vi "Omniax_mDrive_XYZR_MM_BR_RES_2.vi"() -> ()   [LabVIEW 2009]
uses:
  <vilib>/Instr/_visa.llb/VISA Configure Serial Port (Instr).vi
panel:
  out "R Backlash steps/sec":i32
  out "R Backlash":i32
  out "R Holding Current %":i32
  out "R Run Current %":i32
  out "R offset deg":dbl
  out "R deg/rev":dbl
  out "R steps/rev":u32
  out "R velocity PV step/sec":i32
  out "R MINPOS":i32=-94296
  out "R MAXPOS":i32=-34296
  out "R COM PORT":refnum<visa-resource-name>="COM5"
  in  "R Scan set":bool
  in  "R Scan Velocity SP deg/sec":dbl
  in  "R Scan Length SP deg":dbl
  in  "R Move Set":bool
  out "Reset R Motor Steps":i32
  in  "Reset R Position deg":dbl
  out "R Velocity MVdeg/sec":dbl
  in  "R Velocity SP deg/sec":dbl
  in  "R Position SP deg":dbl
  out "R Position MV deg":dbl
  out "R Scan velocity MV deg/sec":dbl format="%#_6f"
  out "R Scan length MV deg":dbl
  in  "R Scan Length SP steps":i32 min=0 max=6144000 step=100
  in  "R Scan OK":bool
  in  "R Velocity SP step/sec":i32 min=1 max=102400
  in  "R Scan Velocity SP steps/sec":i32=1 min=1 max=102400 step=1
  in  "R Go":bool
  in  "R Step SP":i32=-20000 min=0 max=6144000 step=500
  out "R Position deg PV":dbl
  out "R Step PV":i32 max=2000
  out "R Backlash corr":bool
  out "R in Motion":bool
  out "R Scan":bool
  out "R in Range":bool
  out "Z COM PORT":refnum<visa-resource-name>="COM5"
  out "Z Backlash steps/sec":i32
  out "Z Backlash":i32
  out "Z Holding Current %":i32
  out "Z Run Current %":i32
  out "Z offset mm":dbl
  out "Z mm/rev":dbl
  out "Z steps/rev":u32
  out "Z  velocity PV step/sec":i32
  out "Z MINPOS":i32=-94296
  out "Z MAXPOS":i32=-34296
  in  "Z Scan set":bool
  in  "Z Scan Velocity SP mm/sec":dbl
  in  "Z Scan Length SP mm":dbl
  in  "Z Move Set":bool
  out "Reset Z Motor Steps":i32
  in  "Reset Z Position mm":dbl
  out "Z Velocity MV mm/sec":dbl
  in  "Z Velocity SP mm/sec":dbl
  in  "Z Position SP mm":dbl
  out "Z Position MV mm":dbl
  out "Z Scan velocity MV mm/sec":dbl format="%#_6f"
  out "Z Scan length MV mm":dbl
  in  "Z Scan Length SP steps":i32 min=0 max=2048000 step=100
  in  "Z Scan OK":bool
  in  "Z Velocity SP step/sec":i32 min=1 max=102400
  in  "Z Scan Velocity SP steps/sec":i32=1 min=1 max=102400 step=1
  in  "Z Go":bool
  in  "Z Step SP":i32=-20000 min=0 max=2048000 step=500
  out "Z Position mm PV":dbl
  out "Z Step PV":i32 max=2000
  out "Z Backlash corr":bool
  out "Z in Motion":bool
  out "Z Scan":bool
  out "Z in Range":bool
  out "Reset X Motor Steps":i32
  in  "Reset X Position mm":dbl
  out "X Backlash corr":bool
  out "X  in Motion":bool
  out "X Scan":bool
  out "X  in Range":bool
  out "X Step PV":i32 max=2000
  out "X Position mm PV":dbl
  out "X velocity PV step/sec":i32
  in  "X Scan set":bool
  in  "X Scan Velocity SP mm/sec":dbl
  in  "X Scan Length SP mm":dbl
  in  "X Move Set":bool
  out "X Velocity MV mm/sec":dbl
  in  "X Velocity SP mm/sec":dbl
  in  "X Position SP mm":dbl
  out "X Position MV mm":dbl
  out "X Scan velocity MV mm/sec":dbl format="%#_6f"
  out "X Scan length MV mm":dbl
  in  "X Scan Length SP steps":i32 min=-460800 max=460800 step=100
  in  "X Scan OK":bool
  in  "X Velocity SP step/sec":i32 min=1 max=102400
  in  "X Scan Velocity SP steps/sec":i32=1 min=1 max=102400 step=1
  in  "X Go":bool
  in  "X Step SP":i32=-20000 min=-460800 max=460800 step=500
  out "X Backlash steps/sec":i32
  out "X Backlash":i32
  out "X Holding Current %":i32
  out "X Run Current %":i32
  out "X offset mm":dbl
  out "X mm/rev":dbl
  out "X steps/rev":u32
  out "X MAXPOS":i32=-34296
  out "X MINPOS":i32=-94296
  out "X COM PORT":refnum<visa-resource-name>="COM5"
  out "Y Backlash corr":bool
  in  "Y Scan set":bool
  in  "Y Scan Velocity SP mm/sec":dbl
  in  "Y Scan Length SP mm":dbl
  in  "Y Move Set":bool
  out "Y Backlash steps/sec":i32
  out "Y Backlash":i32
  out "Y in Motion":bool
  in  "Reset":bool
  out "Reset Y Motor Steps":i32
  in  "Reset Y Position mm":dbl
  out "Y Velocity MV mm/sec":dbl
  in  "Y Velocity SP mm/sec":dbl
  in  "Y Position SP mm":dbl
  out "Y Position MV mm":dbl
  out "Y Holding Current %":i32
  out "Y Run Current %":i32
  out "Y Scan velocity MV mm/sec":dbl format="%#_6f"
  out "Y Scan length MV mm":dbl
  in  "Scan Cancel":bool
  out "Y Position mm PV":dbl
  out "Y offset mm":dbl
  out "Y mm/rev":dbl
  out "Y steps/rev":u32
  out "Y velocity PV step/sec":i32
  in  "Y Scan Length SP steps":i32 min=-460800 max=460800 step=100
  out "Y Scan":bool
  in  "Y Scan OK":bool
  in  "Scan Go":bool
  in  "Y Velocity SP step/sec":i32 min=1 max=102400
  in  "Y Scan Velocity SP steps/sec":i32=1 min=1 max=102400 step=1
  in  "Stop":bool
  out "Y in Range":bool
  out "Y Step PV":i32 max=2000
  in  "Y Go":bool
  in  "Y Step SP":i32=-20000 min=-460800 max=460800 step=500
  out "Y MINPOS":i32=-94296
  out "Y MAXPOS":i32=-34296
  out "Y COM PORT":refnum<visa-resource-name>="COM5"
  # "LM"
  # "MV"
  # "BL"
  # "SC"
  # "MX"
  # "MY"
  # "MZ"
  # "MR"
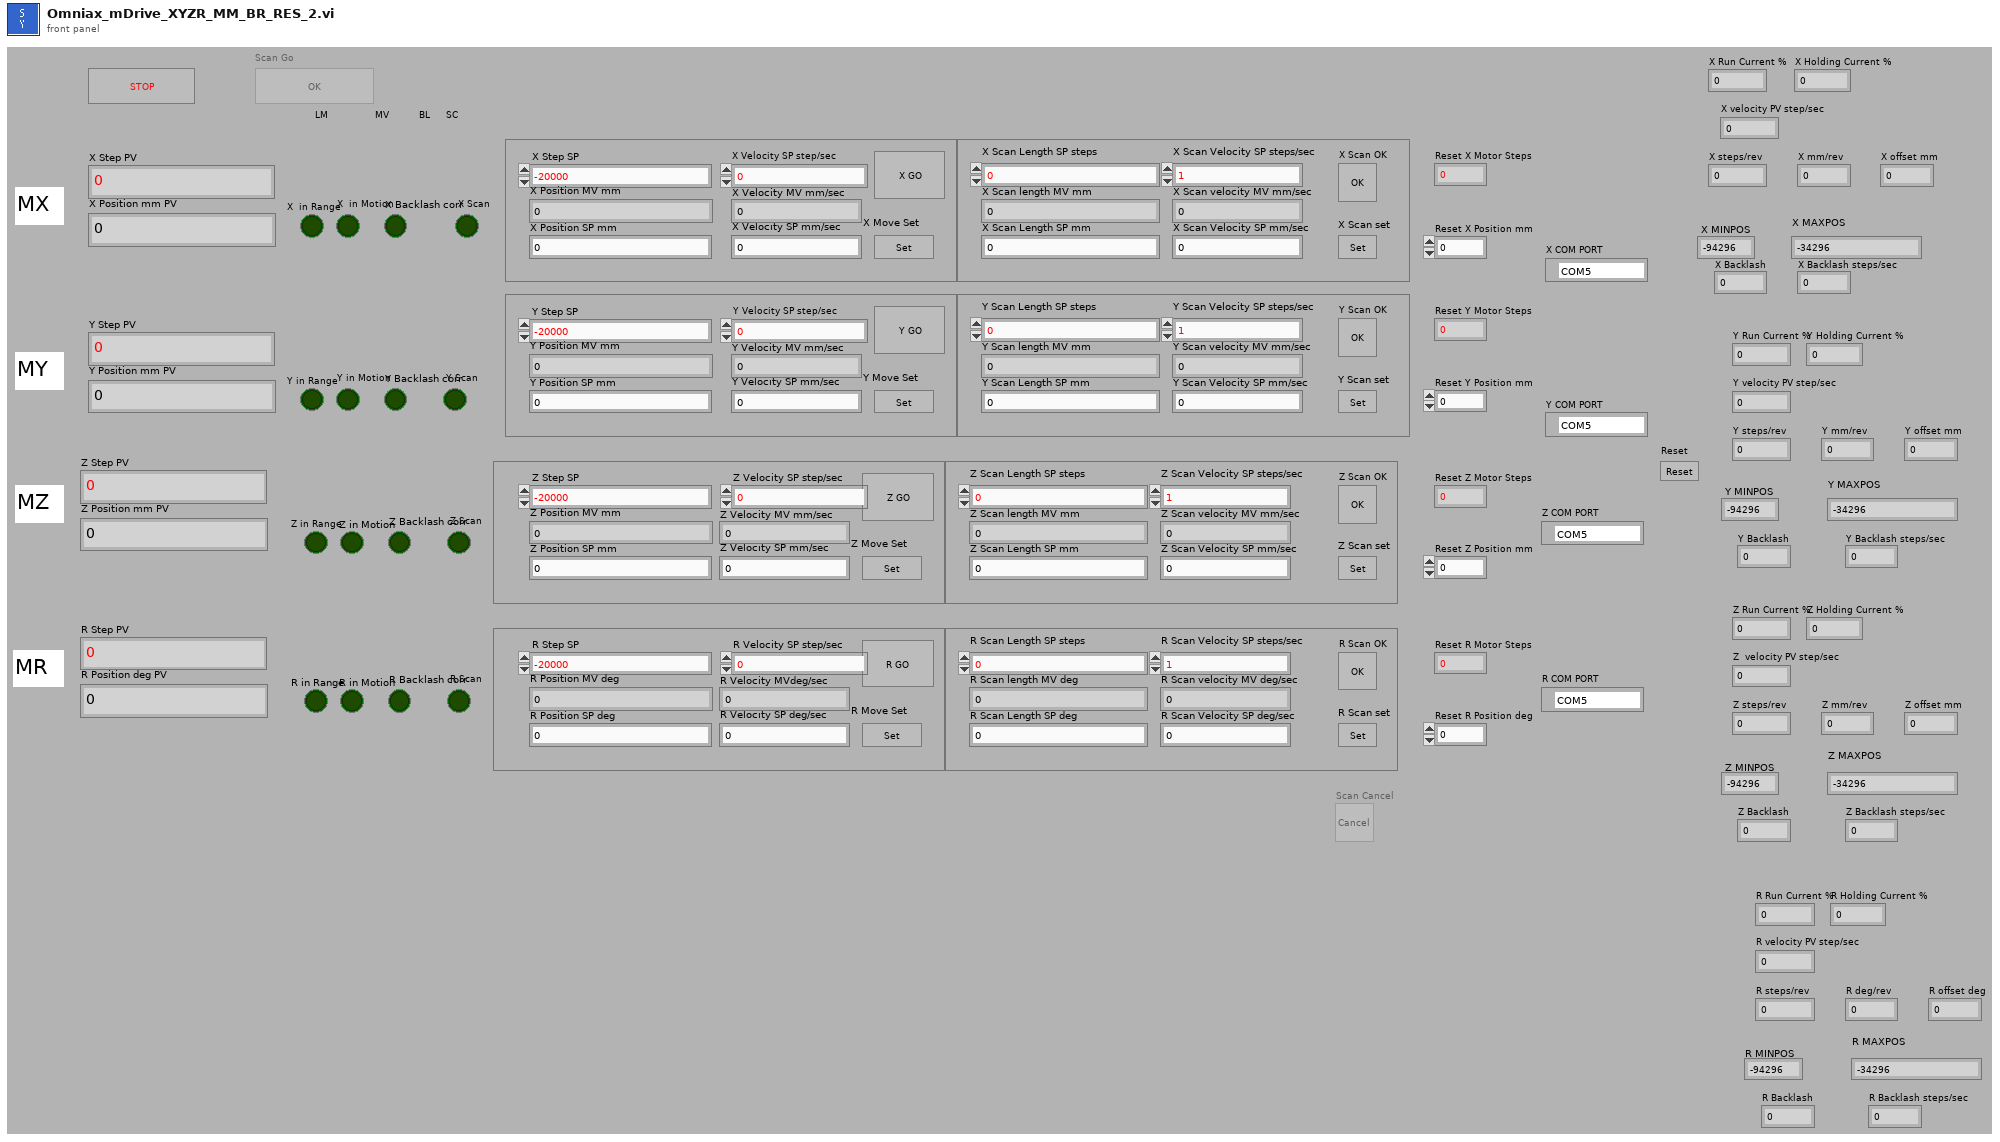
[diagram p1: front panel]
types:
  T1 = enum8{"Enabled", "Disabled", "Disabled and Grayed Out"}
  T2 = enum16{"Stop", "Reset", "Run Current", "Holding Current", "Accel Rate", "Decel Rate", "Move to Relative Position", "Move to Absolute Position", "Echo Mode", "Print Parameter", "Send String", "Microstep Resolution", "Set Current Position", "Max Velocity"}
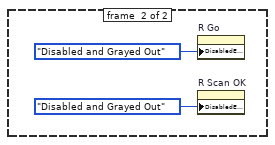
[diagram p2: hidden frame]
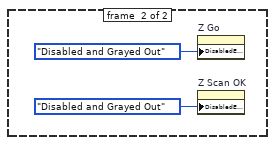
[diagram p5: hidden frame]
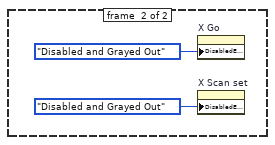
[diagram p8: hidden frame]
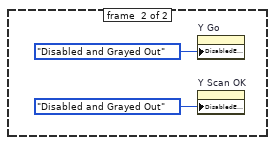
[diagram p11: hidden frame]
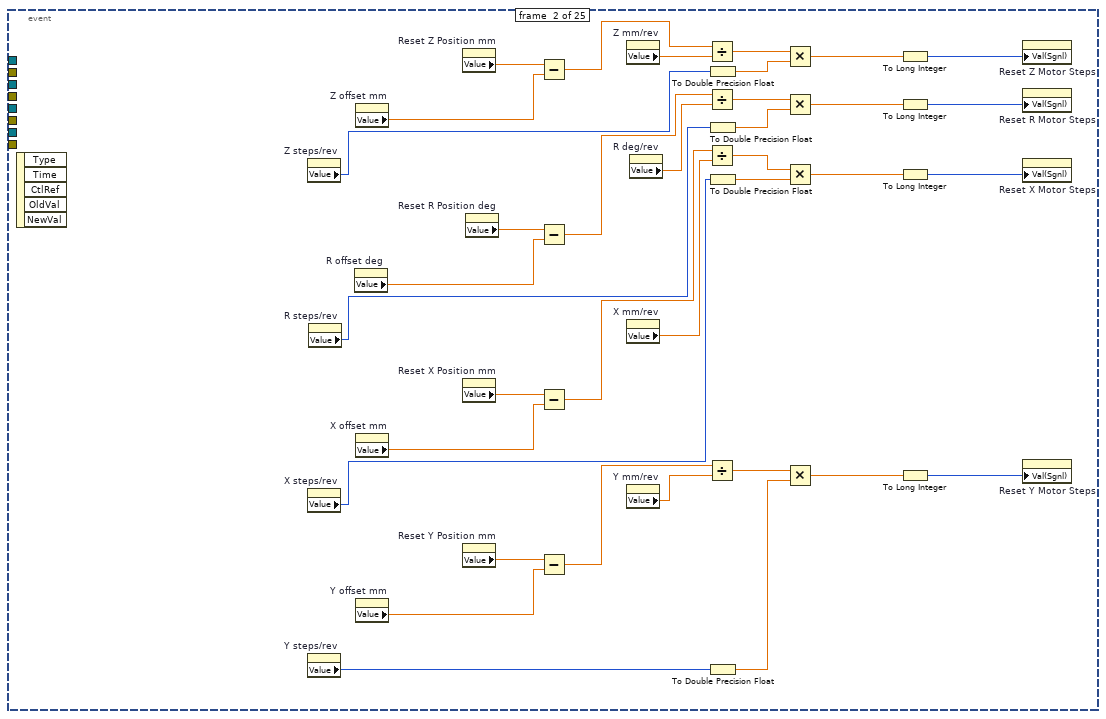
[diagram p14: hidden frame]
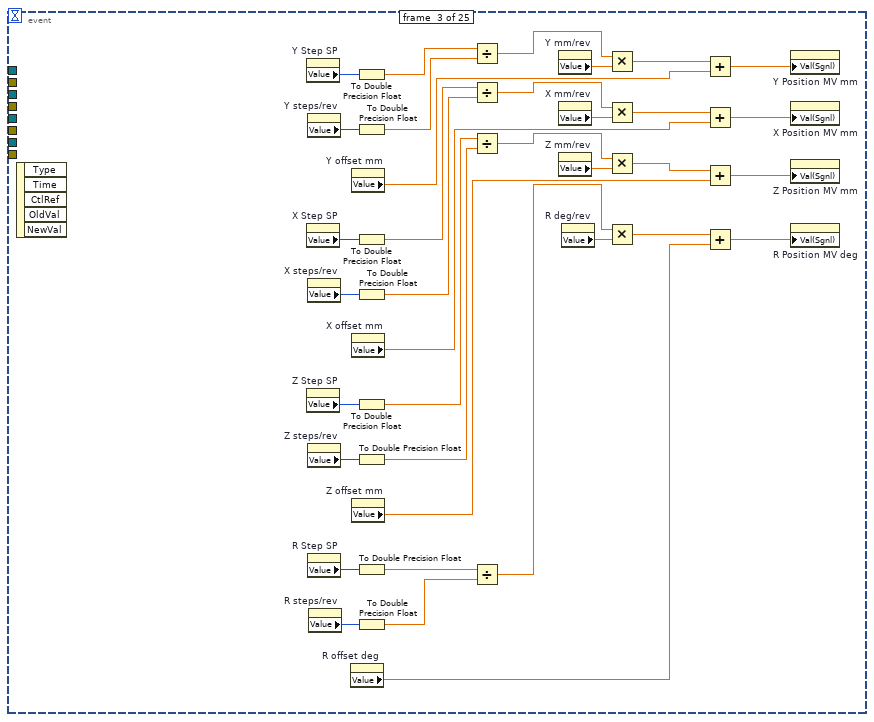
[diagram p15: hidden frame]
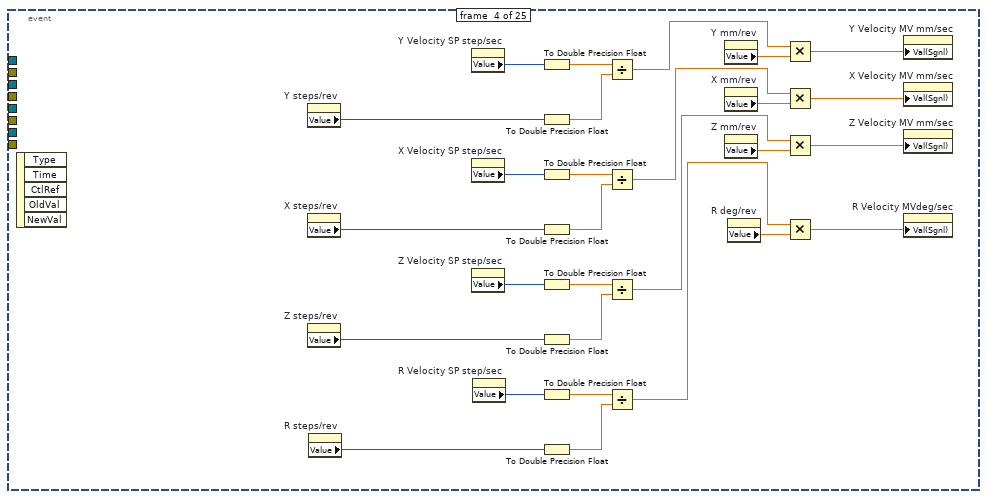
[diagram p16: hidden frame]
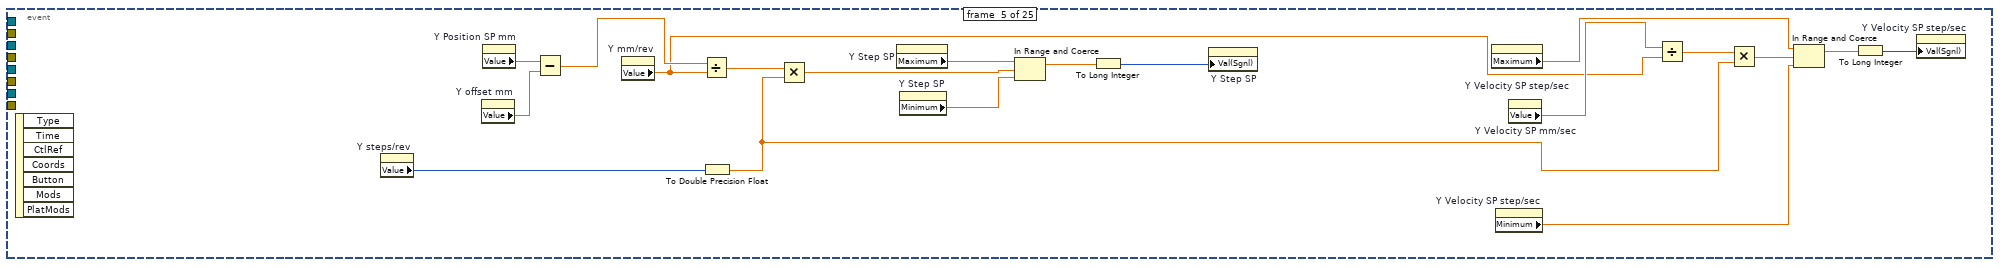
[diagram p17: hidden frame]
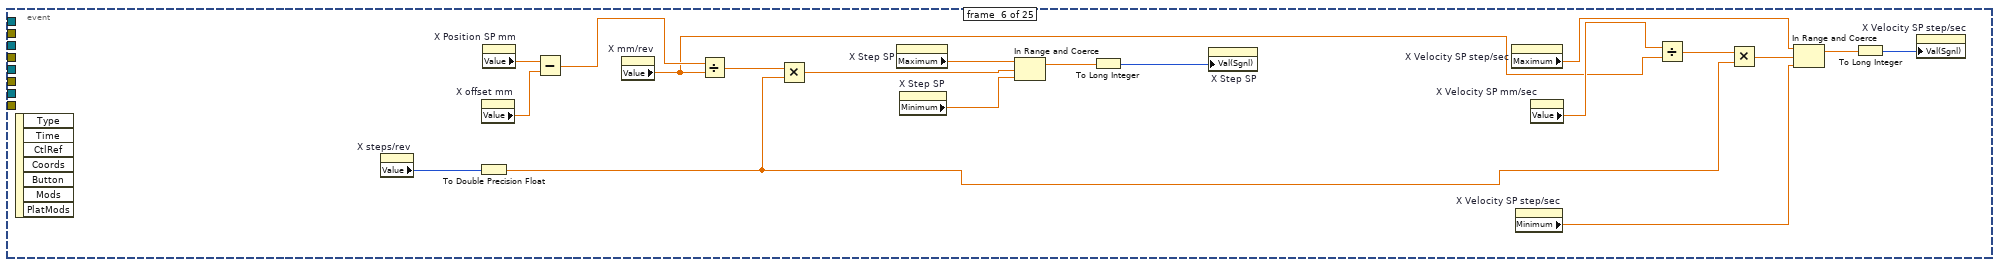
[diagram p18: hidden frame]
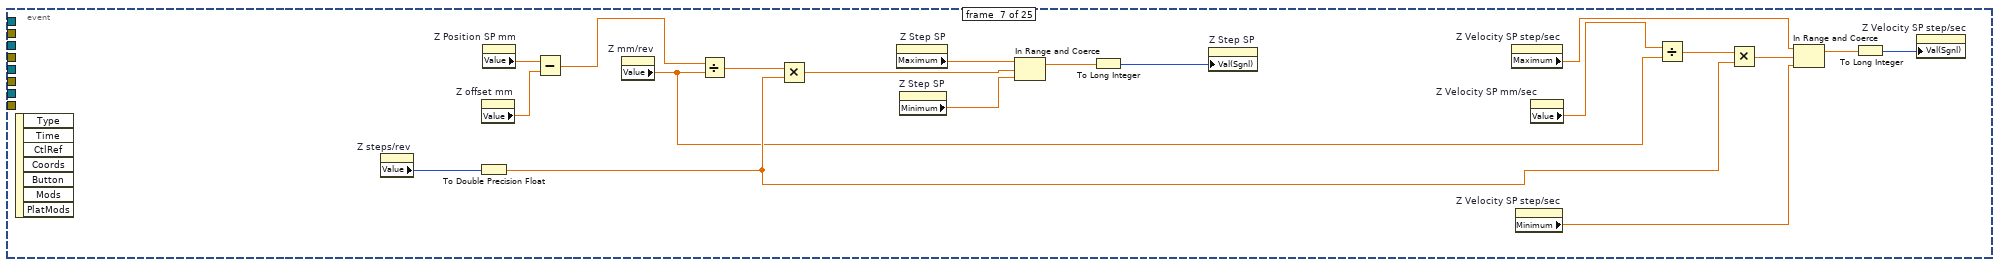
[diagram p19: hidden frame]
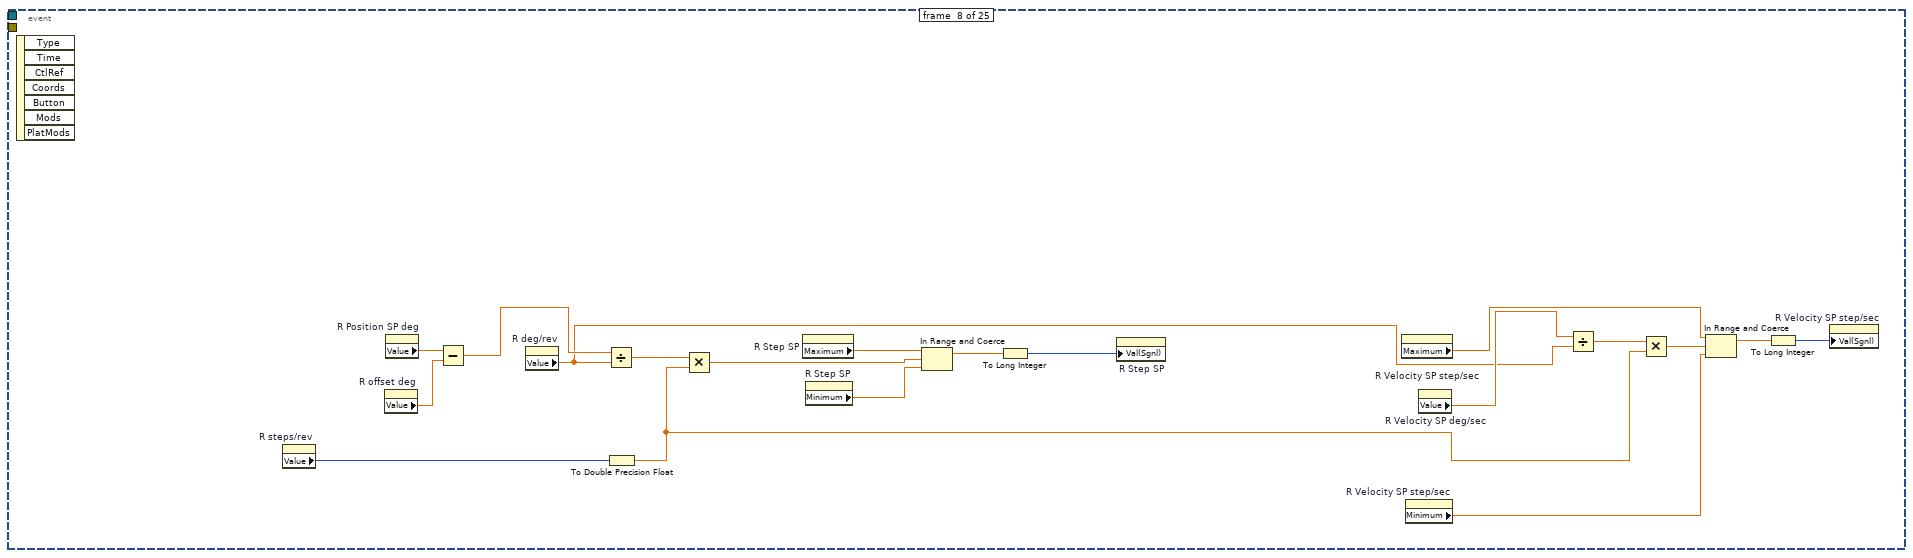
[diagram p20: hidden frame]
diagram:
  w19 = refnum<visa-resource-name> "COM11" ("COM PORT")
  w21 = u16 0 items=["None", "XON/XOFF", "RTS/CTS", "XON/XOFF & RTS/CTS", "DTR/DSR", "XON/XOFF & DTR/DSR"] ("flow control (0:none)")
  w22 = u16 10 items=["1.0"=10, "1.5"=15, "2.0"=20] ("stop bits (10: 1 bit)")
  w52 = refnum<visa-resource-name> "COM10" ("COM PORT")
  w54 = u16 0 items=["None", "XON/XOFF", "RTS/CTS", "XON/XOFF & RTS/CTS", "DTR/DSR", "XON/XOFF & DTR/DSR"] ("flow control (0:none)")
  w55 = u16 10 items=["1.0"=10, "1.5"=15, "2.0"=20] ("stop bits (10: 1 bit)")
  w65 = refnum<visa-resource-name> "COM8" ("COM PORT")
  w67 = u16 0 items=["None", "XON/XOFF", "RTS/CTS", "XON/XOFF & RTS/CTS", "DTR/DSR", "XON/XOFF & DTR/DSR"] ("flow control (0:none)")
  w68 = u16 10 items=["1.0"=10, "1.5"=15, "2.0"=20] ("stop bits (10: 1 bit)")
  w90 = refnum<visa-resource-name> "COM9" ("COM PORT")
  w92 = u16 0 items=["None", "XON/XOFF", "RTS/CTS", "XON/XOFF & RTS/CTS", "DTR/DSR", "XON/XOFF & DTR/DSR"] ("flow control (0:none)")
  w93 = u16 10 items=["1.0"=10, "1.5"=15, "2.0"=20] ("stop bits (10: 1 bit)")
  # "Stop bits"
  # "Stop bits"
  # "Stop bits"
  # "Stop bits"
  n1 = flat-sequence {
    frame #0 {
      w101 = 3.0 ("R deg/rev")
      w99 = u32 51200 ("step/rev")
      w103 = 102400 ("Value (Signaling)")
      n2 = property on="R Velocity SP step/sec" class="DigNum (strict)"("Val(Sgnl)"=w103) -> ()  [unwired: 2 in, 2 out]
      n3 = property on="R Velocity SP step/sec" class="DigNum (strict)"("Minimum"=1.0 ("Data Entry Limits:Minimum")) -> ()  [unwired: 2 in, 2 out]
      n4 = To Double Precision Float(number=w99) -> (double precision float=w100:dbl)
      n5 = To Double Precision Float(number=w103) -> (double precision float=w105:dbl)
      n6 = Divide(x=w105, y=w100) -> (x/y=w104:dbl)
      n7 = property on="R Velocity SP step/sec" class="DigNum (strict)"("Maximum"=w105) -> ()  [unwired: 2 in, 2 out]
      n8 = Multiply(x=w104, y=w101) -> (x*y=w102:dbl)
      n9 = property on="R Velocity SP deg/sec" class="DigNum (strict)"("Val(Sgnl)"=w102) -> ()  [unwired: 2 in, 2 out]
      "R offset deg" <- 0.0 ("R offset deg")
      "R deg/rev" <- w101
      "R steps/rev" <- w99
    }
  }
  n10 = flat-sequence {
    frame #0 {
      w108 = 1.0 ("MM/rev")
      w111 = u32 51200 ("step/rev")
      w106 = 102400 ("Value (Signaling)")
      n11 = property on="X Velocity SP step/sec" class="DigNum (strict)"("Minimum"=1.0 ("Data Entry Limits:Minimum")) -> ()  [unwired: 2 in, 2 out]
      n12 = property on="X Velocity SP step/sec" class="DigNum (strict)"("Val(Sgnl)"=w106) -> ()  [unwired: 2 in, 2 out]
      n13 = To Double Precision Float(number=w111) -> (double precision float=w110:dbl)
      n14 = To Double Precision Float(number=w106) -> (double precision float=w112:dbl)
      n15 = Divide(x=w112, y=w110) -> (x/y=w107:dbl)
      n16 = property on="X Velocity SP step/sec" class="DigNum (strict)"("Maximum"=w112) -> ()  [unwired: 2 in, 2 out]
      n17 = Multiply(x=w107, y=w108) -> (x*y=w109:dbl)
      n18 = property on="X Velocity SP mm/sec" class="DigNum (strict)"("Val(Sgnl)"=w109) -> ()  [unwired: 2 in, 2 out]
      "X offset mm" <- 0.0 ("offset")
      "X steps/rev" <- w111
      "X mm/rev" <- w108
    }
  }
  n19 = flat-sequence {
    frame #0 {
      w116 = 1.0 ("Z mm/rev")
      w115 = u32 51200 ("step/rev")
      w117 = 102400 ("Value (Signaling)")
      n20 = property on="Z Velocity SP step/sec" class="DigNum (strict)"("Val(Sgnl)"=w117) -> ()  [unwired: 2 in, 2 out]
      n21 = property on="Z Velocity SP step/sec" class="DigNum (strict)"("Minimum"=1.0 ("Data Entry Limits:Minimum")) -> ()  [unwired: 2 in, 2 out]
      n22 = To Double Precision Float(number=w115) -> (double precision float=w120:dbl)
      n23 = To Double Precision Float(number=w117) -> (double precision float=w121:dbl)
      n24 = Divide(x=w121, y=w120) -> (x/y=w118:dbl)
      n25 = property on="Z Velocity SP step/sec" class="DigNum (strict)"("Maximum"=w121) -> ()  [unwired: 2 in, 2 out]
      n26 = Multiply(x=w118, y=w116) -> (x*y=w119:dbl)
      n27 = property on="Z Velocity SP mm/sec" class="DigNum (strict)"("Val(Sgnl)"=w119) -> ()  [unwired: 2 in, 2 out]
      "Z offset mm" <- 0.0 ("Z offset mm")
      "Z mm/rev" <- w116
      "Z steps/rev" <- w115
    }
  }
  n28 = flat-sequence {
    frame #0 {
      n29 = property on="X Backlash corr" class="Bool (strict)"("Val(Sgnl)"=FALSE ("Value (Signaling)")) -> ()  [unwired: 2 in, 2 out]
      n30 = property on="R Backlash corr" class="Bool (strict)"("Val(Sgnl)"=FALSE ("Value (Signaling)")) -> ()  [unwired: 2 in, 2 out]
      n31 = property on="Z Backlash corr" class="Bool (strict)"("Val(Sgnl)"=FALSE ("Value (Signaling)")) -> ()  [unwired: 2 in, 2 out]
      n32 = property on="Y Backlash corr" class="Bool (strict)"("Val(Sgnl)"=FALSE ("Value (Signaling)")) -> ()  [unwired: 2 in, 2 out]
      "Z Backlash steps/sec" <- 25600 ("Z Backlash steps/sec")
      "Z Backlash" <- -12800 ("Z Backlash")
      "X Backlash steps/sec" <- 25600 ("Value (Signaling)")
      "X Backlash" <- -5120 ("Backlash2")
      "Y Backlash" <- -5120 ("Backlash2")
      "Y Backlash steps/sec" <- 25600 ("Value (Signaling)")
      "R Backlash steps/sec" <- 25600 ("R Backlash steps/sec")
      "R Backlash" <- -12800 ("R Backlash")
    }
  }
  n33 = flat-sequence {
    frame #0 {
      "Z Holding Current %" <- 25 ("Z Holding Current %")
      "Z Run Current %" <- 60 ("Z Run Current %")
      "X Run Current %" <- 60 ("Run Current %")
      "X Holding Current %" <- 25 ("Holding Current %")
      "Y Run Current %" <- 60 ("Run Current %")
      "Y Holding Current %" <- 25 ("Holding Current %")
      "R Holding Current %" <- 25 ("R Holding Current %")
      "R Run Current %" <- 60 ("R Run Current %")
    }
  }
  n34 = flat-sequence {
    frame #0 {
      n35 = property on="Y Scan" class="Bool (strict)"("Val(Sgnl)"=FALSE ("Value (Signaling)")) -> ()  [unwired: 2 in, 2 out]
      n36 = property on="Y Scan Velocity SP mm/sec" class="DigNum (strict)"("Val(Sgnl)"=0.1 ("Value (Signaling)")) -> ()  [unwired: 2 in, 2 out]
      n37 = property on="Z Scan Velocity SP mm/sec" class="DigNum (strict)"("Val(Sgnl)"=0.1 ("Value (Signaling)")) -> ()  [unwired: 2 in, 2 out]
      n38 = property on="R Scan" class="Bool (strict)"("Val(Sgnl)"=FALSE ("Value (Signaling)")) -> ()  [unwired: 2 in, 2 out]
      n39 = property on="Z Scan" class="Bool (strict)"("Val(Sgnl)"=FALSE ("Value (Signaling)")) -> ()  [unwired: 2 in, 2 out]
      n40 = property on="R Velocity SP deg/sec" class="DigNum (strict)"("Val(Sgnl)"=0.1 ("Value (Signaling)")) -> ()  [unwired: 2 in, 2 out]
      n41 = property on="X Scan" class="Bool (strict)"("Val(Sgnl)"=FALSE ("Value (Signaling)")) -> ()  [unwired: 2 in, 2 out]
      n42 = property on="X Scan Velocity SP mm/sec" class="DigNum (strict)"("Val(Sgnl)"=0.1 ("Value (Signaling)")) -> ()  [unwired: 2 in, 2 out]
      n43 = property on="Scan Go" class="Bool"("DisabledEnum"=T1."Disabled and Grayed Out" ("Disabled")) -> ()  [unwired: 2 in, 2 out]
      n44 = property on="Scan Cancel" class="Bool"("DisabledEnum"=T1."Disabled and Grayed Out" ("Disabled")) -> ()  [unwired: 2 in, 2 out]
    }
  }
  n45 = flat-sequence {
    frame #0 {
      w156 = 1.0 ("MM/rev")
      w159 = u32 51200 ("step/rev")
      w154 = 102400 ("Value (Signaling)")
      n46 = property on="Y Velocity SP step/sec" class="DigNum (strict)"("Minimum"=1.0 ("Data Entry Limits:Minimum")) -> ()  [unwired: 2 in, 2 out]
      n47 = property on="Y Velocity SP step/sec" class="DigNum (strict)"("Val(Sgnl)"=w154) -> ()  [unwired: 2 in, 2 out]
      n48 = To Double Precision Float(number=w159) -> (double precision float=w158:dbl)
      n49 = To Double Precision Float(number=w154) -> (double precision float=w160:dbl)
      n50 = Divide(x=w160, y=w158) -> (x/y=w155:dbl)
      n51 = property on="Y Velocity SP step/sec" class="DigNum (strict)"("Maximum"=w160) -> ()  [unwired: 2 in, 2 out]
      n52 = Multiply(x=w155, y=w156) -> (x*y=w157:dbl)
      n53 = property on="Y Velocity SP mm/sec" class="DigNum (strict)"("Val(Sgnl)"=w157) -> ()  [unwired: 2 in, 2 out]
      "Y offset mm" <- 0.0 ("offset")
      "Y steps/rev" <- w159
      "Y mm/rev" <- w156
    }
  }
  n54 = call-poly "VISA Configure Serial Port"("VISA resource name"=w90, "timeout (10sec)"=u32 10000, "baud rate (9600)"=u32 9600, "data bits (8)"=u16 8, "parity (0:none)"=enum16{"None", "Odd", "Even", "Mark", "Space"}."None", "stop bits (10: 1 bit)"=w93, "flow control (0:none)"=w92) -> ("VISA resource name out"=w83:refnum<visa-resource-name>, "error out"=w82:errorcluster)  [unwired: 7 in]
  n55 = flat-sequence {
    tunnel: w82 -> [w165]
    tunnel: w83 -> [w166]
    tunnel: [w166] -> w4
    tunnel: [w165] -> w3
    tunnel: [w170] -> w81
    tunnel: [w172] -> w79
    tunnel: w4 -> [w171]
    tunnel: w3 -> [w173]
    tunnel: w81 -> [w180]
    tunnel: [w179] -> w80
    tunnel: w79 -> [w177]
    tunnel: [w178] -> w78
    tunnel: [w190] -> w85
    tunnel: [w191] -> w84
    tunnel: w80 -> [w189]
    tunnel: w78 -> [w188]
    tunnel: w85 -> [w201]
    tunnel: w84 -> [w200]
    tunnel: [w203] -> w51
    tunnel: [w202] -> w50
    tunnel: [w197] -> w49
    tunnel: [w208] -> w88
    tunnel: [w209] -> w89
    tunnel: w51 -> [w209]
    tunnel: w50 -> [w208]
    tunnel: w49 -> [w204]
    frame #0 {
      n56 = call "mDrive Send Command.vi"("Extra"="EM=2", "Command"=T2."Send String") -> ()  [unwired: 5 in, 3 out]
    }
    frame #1 {
      # "Run Current %"
      n57 = property on="Y Run Current %" class="DigNum (strict)"() -> ("Value"=w168:i32)  [unwired: 2 in, 2 out]
      n58 = Number To Decimal String(number=w168) -> (decimal integer string=w169:string)  [unwired: 1 in]
      n59 = call "mDrive Send Command.vi"("error in (no error)"=w173, "Extra"=w169, "Command"=T2."Run Current", "VISA resource name"=w171) -> ("error out"=w172:errorcluster, "VISA resource name out"=w170:refnum<visa-resource-name>)  [unwired: 3 in, 1 out]
    }
    frame #2 {
      # "Holding Current %"
      n60 = property on="Y Holding Current %" class="DigNum (strict)"() -> ("Value"=w175:i32)  [unwired: 2 in, 2 out]
      n61 = Number To Decimal String(number=w175) -> (decimal integer string=w176:string)  [unwired: 1 in]
      n62 = call "mDrive Send Command.vi"("error in (no error)"=w177, "Extra"=w176, "Command"=T2."Holding Current", "VISA resource name"=w180) -> ("error out"=w178:errorcluster, "VISA resource name out"=w179:refnum<visa-resource-name>)  [unwired: 3 in, 1 out]
    }
    frame #3 {
      # "Print Velocity Ma"
      # "Velocity Max"
      n63 = property on="Y Velocity SP step/sec" class="DigNum (strict)"() -> ("Value"=w187:i32)  [unwired: 2 in, 2 out]
      n64 = Number To Decimal String(number=w187) -> (decimal integer string=w186:string)  [unwired: 1 in]
      n65 = call "mDrive Send Command.vi"("error in (no error)"=w188, "Extra"=w186, "Command"=T2."Max Velocity", "VISA resource name"=w189) -> ("error out"=w184:errorcluster, "VISA resource name out"=w194:refnum<visa-resource-name>)  [unwired: 3 in, 1 out]
      n66 = call "mDrive Send Command.vi"("error in (no error)"=w184, "Extra"="VM", "Command"=T2."Print Parameter", "VISA resource name"=w194) -> ("error out"=w191:errorcluster, "read buffer"=w192:string, "VISA resource name out"=w190:refnum<visa-resource-name>)  [unwired: 3 in]
      n67 = Decimal String To Number(string=w192, offset=0) -> (number=w185:i32)  [unwired: 1 in, 1 out]
      n68 = property on="Y scan velocity MV step/sec" class="DigNum (strict)"("Val(Sgnl)"=w185) -> ()  [unwired: 2 in, 2 out]
    }
    frame #4 {
      # "PRINT POSITION"
      n69 = call "mDrive Send Command.vi"("error in (no error)"=w200, "Extra"="P", "Command"=T2."Print Parameter", "VISA resource name"=w201) -> ("error out"=w202:errorcluster, "read buffer"=w199:string, "VISA resource name out"=w203:refnum<visa-resource-name>)  [unwired: 3 in]
      n70 = Decimal String To Number(string=w199, offset=0) -> (number=w197:i32)  [unwired: 1 in, 1 out]
    }
    frame #5 {
      w206 = -460800 ("lower limit")
      w207 = 460800 ("upper limit")
      n71 = property on="Y Step SP" class="DigNum (strict)"("Val(Sgnl)"=w204) -> ()  [unwired: 2 in, 2 out]
      n72 = property on="Y Step SP" class="DigNum (strict)"("Maximum"=w207) -> ()  [unwired: 2 in, 2 out]
      n73 = property on="Y Step SP" class="DigNum (strict)"("Minimum"=w206) -> ()  [unwired: 2 in, 2 out]
      n74 = In Range and Coerce(upper limit=w207, x=w204, lower limit=w206) -> (In Range?=w205:bool)  [unwired: 1 out]
      n75 = property on="Y in Range" class="Bool (strict)"("Val(Sgnl)"=w205) -> ()  [unwired: 2 in, 2 out]
      "Y MINPOS" <- w206
      "Y MAXPOS" <- w207
    }
  }
  n76 = call-poly "VISA Configure Serial Port"("VISA resource name"=w65, "timeout (10sec)"=u32 10000, "baud rate (9600)"=u32 9600, "data bits (8)"=u16 8, "parity (0:none)"=enum16{"None", "Odd", "Even", "Mark", "Space"}."None", "stop bits (10: 1 bit)"=w68, "flow control (0:none)"=w67) -> ("VISA resource name out"=w64:refnum<visa-resource-name>, "error out"=w63:errorcluster)  [unwired: 7 in]
  n77 = call-poly "VISA Configure Serial Port"("VISA resource name"=w19, "timeout (10sec)"=u32 10000, "baud rate (9600)"=u32 9600, "data bits (8)"=u16 8, "parity (0:none)"=enum16{"None", "Odd", "Even", "Mark", "Space"}."None", "stop bits (10: 1 bit)"=w22, "flow control (0:none)"=w21) -> ("VISA resource name out"=w18:refnum<visa-resource-name>, "error out"=w17:errorcluster)  [unwired: 7 in]
  n78 = flat-sequence {
    tunnel: w17 -> [w212]
    tunnel: w18 -> [w213]
    tunnel: [w213] -> w8
    tunnel: [w212] -> w7
    tunnel: [w218] -> w34
    tunnel: [w220] -> w33
    tunnel: w8 -> [w219]
    tunnel: w7 -> [w214]
    tunnel: w34 -> [w227]
    tunnel: [w226] -> w32
    tunnel: w33 -> [w224]
    tunnel: [w225] -> w31
    tunnel: [w237] -> w30
    tunnel: [w238] -> w29
    tunnel: w32 -> [w236]
    tunnel: w31 -> [w235]
    tunnel: w30 -> [w248]
    tunnel: w29 -> [w247]
    tunnel: [w250] -> w28
    tunnel: [w249] -> w27
    tunnel: [w244] -> w26
    tunnel: [w255] -> w11
    tunnel: [w256] -> w12
    tunnel: w28 -> [w256]
    tunnel: w27 -> [w255]
    tunnel: w26 -> [w253]
    frame #0 {
      n79 = call "mDrive Send Command.vi"("Extra"="EM=2", "Command"=T2."Send String") -> ()  [unwired: 5 in, 3 out]
    }
    frame #1 {
      # "Run Current %"
      n80 = property on="R Run Current %" class="DigNum (strict)"() -> ("Value"=w216:i32)  [unwired: 2 in, 2 out]
      n81 = Number To Decimal String(number=w216) -> (decimal integer string=w217:string)  [unwired: 1 in]
      n82 = call "mDrive Send Command.vi"("error in (no error)"=w214, "Extra"=w217, "Command"=T2."Run Current", "VISA resource name"=w219) -> ("error out"=w220:errorcluster, "VISA resource name out"=w218:refnum<visa-resource-name>)  [unwired: 3 in, 1 out]
    }
    frame #2 {
      # "Holding Current %"
      n83 = property on="R Holding Current %" class="DigNum (strict)"() -> ("Value"=w222:i32)  [unwired: 2 in, 2 out]
      n84 = Number To Decimal String(number=w222) -> (decimal integer string=w223:string)  [unwired: 1 in]
      n85 = call "mDrive Send Command.vi"("error in (no error)"=w224, "Extra"=w223, "Command"=T2."Holding Current", "VISA resource name"=w227) -> ("error out"=w225:errorcluster, "VISA resource name out"=w226:refnum<visa-resource-name>)  [unwired: 3 in, 1 out]
    }
    frame #3 {
      # "Print Velocity Ma"
      # "Velocity Max"
      n86 = property on="R Velocity SP step/sec" class="DigNum (strict)"() -> ("Value"=w234:i32)  [unwired: 2 in, 2 out]
      n87 = Number To Decimal String(number=w234) -> (decimal integer string=w233:string)  [unwired: 1 in]
      n88 = call "mDrive Send Command.vi"("error in (no error)"=w235, "Extra"=w233, "Command"=T2."Max Velocity", "VISA resource name"=w236) -> ("error out"=w231:errorcluster, "VISA resource name out"=w241:refnum<visa-resource-name>)  [unwired: 3 in, 1 out]
      n89 = call "mDrive Send Command.vi"("error in (no error)"=w231, "Extra"="VM", "Command"=T2."Print Parameter", "VISA resource name"=w241) -> ("error out"=w238:errorcluster, "read buffer"=w239:string, "VISA resource name out"=w237:refnum<visa-resource-name>)  [unwired: 3 in]
      n90 = Decimal String To Number(string=w239, offset=0) -> (number=w232:i32)  [unwired: 1 in, 1 out]
      n91 = property on="R velocity PV step/sec" class="DigNum (strict)"("Val(Sgnl)"=w232) -> ()  [unwired: 2 in, 2 out]
    }
    frame #4 {
      # "PRINT POSITION"
      n92 = call "mDrive Send Command.vi"("error in (no error)"=w247, "Extra"="P", "Command"=T2."Print Parameter", "VISA resource name"=w248) -> ("error out"=w249:errorcluster, "read buffer"=w246:string, "VISA resource name out"=w250:refnum<visa-resource-name>)  [unwired: 3 in]
      n93 = Decimal String To Number(string=w246, offset=0) -> (number=w244:i32)  [unwired: 1 in, 1 out]
    }
    frame #5 {
      w252 = 0 ("lower limit")
      w251 = 6144000 ("upper limit")
      n94 = property on="R Step SP" class="DigNum (strict)"("Val(Sgnl)"=w253) -> ()  [unwired: 2 in, 2 out]
      n95 = property on="R Step SP" class="DigNum (strict)"("Maximum"=w251) -> ()  [unwired: 2 in, 2 out]
      n96 = property on="R Step SP" class="DigNum (strict)"("Minimum"=w252) -> ()  [unwired: 2 in, 2 out]
      n97 = In Range and Coerce(upper limit=w251, x=w253, lower limit=w252) -> (In Range?=w254:bool)  [unwired: 1 out]
      n98 = property on="R in Range" class="Bool (strict)"("Val(Sgnl)"=w254) -> ()  [unwired: 2 in, 2 out]
      "R MINPOS" <- w252
      "R MAXPOS" <- w251
    }
  }
  n99 = flat-sequence {
    tunnel: w63 -> [w259]
    tunnel: w64 -> [w260]
    tunnel: [w260] -> w2
    tunnel: [w259] -> w1
    tunnel: [w264] -> w77
    tunnel: [w266] -> w76
    tunnel: w2 -> [w265]
    tunnel: w1 -> [w267]
    tunnel: w77 -> [w274]
    tunnel: [w273] -> w75
    tunnel: w76 -> [w271]
    tunnel: [w272] -> w74
    tunnel: [w284] -> w73
    tunnel: [w285] -> w72
    tunnel: w75 -> [w283]
    tunnel: w74 -> [w282]
    tunnel: w73 -> [w295]
    tunnel: w72 -> [w294]
    tunnel: [w297] -> w48
    tunnel: [w296] -> w47
    tunnel: [w291] -> w46
    tunnel: [w302] -> w61
    tunnel: [w303] -> w62
    tunnel: w48 -> [w303]
    tunnel: w47 -> [w302]
    tunnel: w46 -> [w298]
    frame #0 {
      n100 = call "mDrive Send Command.vi"("Extra"="EM=2", "Command"=T2."Send String") -> ()  [unwired: 5 in, 3 out]
    }
    frame #1 {
      # "Run Current %"
      n101 = property on="X Run Current %" class="DigNum (strict)"() -> ("Value"=w262:i32)  [unwired: 2 in, 2 out]
      n102 = Number To Decimal String(number=w262) -> (decimal integer string=w263:string)  [unwired: 1 in]
      n103 = call "mDrive Send Command.vi"("error in (no error)"=w267, "Extra"=w263, "Command"=T2."Run Current", "VISA resource name"=w265) -> ("error out"=w266:errorcluster, "VISA resource name out"=w264:refnum<visa-resource-name>)  [unwired: 3 in, 1 out]
    }
    frame #2 {
      # "Holding Current %"
      n104 = property on="X Holding Current %" class="DigNum (strict)"() -> ("Value"=w269:i32)  [unwired: 2 in, 2 out]
      n105 = Number To Decimal String(number=w269) -> (decimal integer string=w270:string)  [unwired: 1 in]
      n106 = call "mDrive Send Command.vi"("error in (no error)"=w271, "Extra"=w270, "Command"=T2."Holding Current", "VISA resource name"=w274) -> ("error out"=w272:errorcluster, "VISA resource name out"=w273:refnum<visa-resource-name>)  [unwired: 3 in, 1 out]
    }
    frame #3 {
      # "Print Velocity Ma"
      # "Velocity Max"
      n107 = property on="X Velocity SP step/sec" class="DigNum (strict)"() -> ("Value"=w281:i32)  [unwired: 2 in, 2 out]
      n108 = Number To Decimal String(number=w281) -> (decimal integer string=w280:string)  [unwired: 1 in]
      n109 = call "mDrive Send Command.vi"("error in (no error)"=w282, "Extra"=w280, "Command"=T2."Max Velocity", "VISA resource name"=w283) -> ("error out"=w278:errorcluster, "VISA resource name out"=w288:refnum<visa-resource-name>)  [unwired: 3 in, 1 out]
      n110 = call "mDrive Send Command.vi"("error in (no error)"=w278, "Extra"="VM", "Command"=T2."Print Parameter", "VISA resource name"=w288) -> ("error out"=w285:errorcluster, "read buffer"=w286:string, "VISA resource name out"=w284:refnum<visa-resource-name>)  [unwired: 3 in]
      n111 = Decimal String To Number(string=w286, offset=0) -> (number=w279:i32)  [unwired: 1 in, 1 out]
      n112 = property on="X velocity PV step/sec" class="DigNum (strict)"("Val(Sgnl)"=w279) -> ()  [unwired: 2 in, 2 out]
    }
    frame #4 {
      # "PRINT POSITION"
      n113 = call "mDrive Send Command.vi"("error in (no error)"=w294, "Extra"="P", "Command"=T2."Print Parameter", "VISA resource name"=w295) -> ("error out"=w296:errorcluster, "read buffer"=w293:string, "VISA resource name out"=w297:refnum<visa-resource-name>)  [unwired: 3 in]
      n114 = Decimal String To Number(string=w293, offset=0) -> (number=w291:i32)  [unwired: 1 in, 1 out]
    }
    frame #5 {
      w300 = -460800 ("lower limit")
      w301 = 460800 ("upper limit")
      n115 = property on="X Step SP" class="DigNum (strict)"("Val(Sgnl)"=w298) -> ()  [unwired: 2 in, 2 out]
      n116 = property on="X Step SP" class="DigNum (strict)"("Maximum"=w301) -> ()  [unwired: 2 in, 2 out]
      n117 = property on="X Step SP" class="DigNum (strict)"("Minimum"=w300) -> ()  [unwired: 2 in, 2 out]
      n118 = In Range and Coerce(upper limit=w301, x=w298, lower limit=w300) -> (In Range?=w299:bool)  [unwired: 1 out]
      n119 = property on="X  in Range" class="Bool (strict)"("Val(Sgnl)"=w299) -> ()  [unwired: 2 in, 2 out]
      "X MINPOS" <- w300
      "X MAXPOS" <- w301
    }
  }
  n120 = call-poly "VISA Configure Serial Port"("VISA resource name"=w52, "timeout (10sec)"=u32 10000, "baud rate (9600)"=u32 9600, "data bits (8)"=u16 8, "parity (0:none)"=enum16{"None", "Odd", "Even", "Mark", "Space"}."None", "stop bits (10: 1 bit)"=w55, "flow control (0:none)"=w54) -> ("VISA resource name out"=w36:refnum<visa-resource-name>, "error out"=w35:errorcluster)  [unwired: 7 in]
  n121 = flat-sequence {
    tunnel: w35 -> [w306]
    tunnel: w36 -> [w307]
    tunnel: [w307] -> w6
    tunnel: [w306] -> w5
    tunnel: [w311] -> w45
    tunnel: [w313] -> w44
    tunnel: w6 -> [w312]
    tunnel: w5 -> [w314]
    tunnel: w45 -> [w321]
    tunnel: [w320] -> w43
    tunnel: w44 -> [w318]
    tunnel: [w319] -> w42
    tunnel: [w331] -> w41
    tunnel: [w332] -> w40
    tunnel: w43 -> [w330]
    tunnel: w42 -> [w329]
    tunnel: w41 -> [w342]
    tunnel: w40 -> [w341]
    tunnel: [w344] -> w39
    tunnel: [w343] -> w38
    tunnel: [w338] -> w37
    tunnel: [w349] -> w15
    tunnel: [w350] -> w16
    tunnel: w39 -> [w350]
    tunnel: w38 -> [w349]
    tunnel: w37 -> [w347]
    frame #0 {
      n122 = call "mDrive Send Command.vi"("Extra"="EM=2", "Command"=T2."Send String") -> ()  [unwired: 5 in, 3 out]
    }
    frame #1 {
      # "Run Current %"
      n123 = property on="Z Run Current %" class="DigNum (strict)"() -> ("Value"=w309:i32)  [unwired: 2 in, 2 out]
      n124 = Number To Decimal String(number=w309) -> (decimal integer string=w310:string)  [unwired: 1 in]
      n125 = call "mDrive Send Command.vi"("error in (no error)"=w314, "Extra"=w310, "Command"=T2."Run Current", "VISA resource name"=w312) -> ("error out"=w313:errorcluster, "VISA resource name out"=w311:refnum<visa-resource-name>)  [unwired: 3 in, 1 out]
    }
    frame #2 {
      # "Holding Current %"
      n126 = property on="Z Run Current %" class="DigNum (strict)"() -> ("Value"=w316:i32)  [unwired: 2 in, 2 out]
      n127 = Number To Decimal String(number=w316) -> (decimal integer string=w317:string)  [unwired: 1 in]
      n128 = call "mDrive Send Command.vi"("error in (no error)"=w318, "Extra"=w317, "Command"=T2."Holding Current", "VISA resource name"=w321) -> ("error out"=w319:errorcluster, "VISA resource name out"=w320:refnum<visa-resource-name>)  [unwired: 3 in, 1 out]
    }
    frame #3 {
      # "Print Velocity Ma"
      # "Velocity Max"
      n129 = property on="Z Velocity SP step/sec" class="DigNum (strict)"() -> ("Value"=w328:i32)  [unwired: 2 in, 2 out]
      n130 = Number To Decimal String(number=w328) -> (decimal integer string=w327:string)  [unwired: 1 in]
      n131 = call "mDrive Send Command.vi"("error in (no error)"=w329, "Extra"=w327, "Command"=T2."Max Velocity", "VISA resource name"=w330) -> ("error out"=w325:errorcluster, "VISA resource name out"=w335:refnum<visa-resource-name>)  [unwired: 3 in, 1 out]
      n132 = call "mDrive Send Command.vi"("error in (no error)"=w325, "Extra"="VM", "Command"=T2."Print Parameter", "VISA resource name"=w335) -> ("error out"=w332:errorcluster, "read buffer"=w333:string, "VISA resource name out"=w331:refnum<visa-resource-name>)  [unwired: 3 in]
      n133 = Decimal String To Number(string=w333, offset=0) -> (number=w326:i32)  [unwired: 1 in, 1 out]
      n134 = property on="Z  velocity PV step/sec" class="DigNum (strict)"("Val(Sgnl)"=w326) -> ()  [unwired: 2 in, 2 out]
    }
    frame #4 {
      # "PRINT POSITION"
      n135 = call "mDrive Send Command.vi"("error in (no error)"=w341, "Extra"="P", "Command"=T2."Print Parameter", "VISA resource name"=w342) -> ("error out"=w343:errorcluster, "read buffer"=w340:string, "VISA resource name out"=w344:refnum<visa-resource-name>)  [unwired: 3 in]
      n136 = Decimal String To Number(string=w340, offset=0) -> (number=w338:i32)  [unwired: 1 in, 1 out]
    }
    frame #5 {
      w345 = 0 ("lower limit")
      w346 = 2048000 ("upper limit")
      n137 = property on="Z Step SP" class="DigNum (strict)"("Val(Sgnl)"=w347) -> ()  [unwired: 2 in, 2 out]
      n138 = property on="Z Step SP" class="DigNum (strict)"("Maximum"=w346) -> ()  [unwired: 2 in, 2 out]
      n139 = property on="Z Step SP" class="DigNum (strict)"("Minimum"=w345) -> ()  [unwired: 2 in, 2 out]
      n140 = In Range and Coerce(upper limit=w346, x=w347, lower limit=w345) -> (In Range?=w348:bool)  [unwired: 1 out]
      n141 = property on="Z in Range" class="Bool (strict)"("Val(Sgnl)"=w348) -> ()  [unwired: 2 in, 2 out]
      "Z MINPOS" <- w345
      "Z MAXPOS" <- w346
    }
  }
  n142 = while {
    tunnel: w89 -> [w364]
    tunnel: w88 -> [w367]
    tunnel: [w368] -> w86
    tunnel: [w366] -> w87
    tunnel: w62 -> [w362]
    tunnel: w61 -> [w361]
    tunnel: [w360] -> w60
    tunnel: [w359] -> w59
    tunnel: w16 -> [w358]
    tunnel: w15 -> [w357]
    tunnel: [w356] -> w14
    tunnel: [w355] -> w13
    tunnel: w12 -> [w354]
    tunnel: w11 -> [w353]
    tunnel: [w352] -> w10
    tunnel: [w351] -> w9
    stop <- w363 stop-if-true
    n143 = event shown="[15] \"X Go\": Mouse Up" {
      selector: _ -> [_ _ _ _ _ _ _ _ _ _ _ _ _ _ _ _ _ _ _ _ _ _ _ _ _]
      dyn-events: _ -> [_ _ _ _ _ _ _ _ _ _ _ _ _ _ _ _ _ _ _ _ _ _ _ _ _]
      timeout: 500 -> [_ _ _ _ _ _ _ _ _ _ _ _ _ _ _ _ _ _ _ _ _ _ _ _ _]
      tunnel: w367 -> [w436 _ _ _ _ _ _ _ _ _ _ _ w1277 _ _ _ _ w1526 _ _ w1622 w1638 w1682 w1754 w1818]
      tunnel: [w435 _ _ _ _ _ _ _ _ _ _ _ w1283 _ _ _ _ w1524 _ _ w1622 w1636 w1684 w1751 w1816] -> w368
      tunnel: w364 -> [w433 _ _ _ _ _ _ _ _ _ _ _ w1278 _ _ _ _ w1525 _ _ w1623 w1639 w1683 w1753 w1819]
      tunnel: [w434 _ _ _ _ _ _ _ _ _ _ _ w1284 _ _ _ _ w1521 _ _ w1623 w1637 w1685 w1752 w1817] -> w366
      tunnel: [_ _ _ _ _ _ _ _ _ _ _ _ _ _ _ _ _ _ _ _ TRUE _ _ _ _] -> w363
      tunnel: w362 -> [w406 _ _ _ _ _ _ _ _ _ _ _ _ _ _ w1435 w1490 _ _ _ _ w1633 w1675 _ w1815]
      tunnel: w361 -> [w405 _ _ _ _ _ _ _ _ _ _ _ _ _ _ w1434 w1489 _ _ _ _ w1632 w1674 _ w1814]
      tunnel: [w404 _ _ _ _ _ _ _ _ _ _ _ _ _ _ w1433 w1488 _ _ _ _ w1635 w1673 _ w1813] -> w360
      tunnel: [w403 _ _ _ _ _ _ _ _ _ _ _ _ _ _ w1432 w1487 _ _ _ _ w1634 w1672 _ w1812] -> w359
      tunnel: w358 -> [w373 _ _ _ _ _ _ _ _ _ _ _ _ w1329 _ _ _ _ w1556 _ _ w1631 w1669 _ w1811]
      tunnel: w357 -> [w376 _ _ _ _ _ _ _ _ _ _ _ _ w1328 _ _ _ _ w1555 _ _ w1630 w1668 _ w1810]
      tunnel: [w375 _ _ _ _ _ _ _ _ _ _ _ _ w1326 _ _ _ _ w1553 _ _ w1629 w1667 _ w1807] -> w356
      tunnel: [w374 _ _ _ _ _ _ _ _ _ _ _ _ w1327 _ _ _ _ w1554 _ _ w1628 w1666 _ w1806] -> w355
      tunnel: w354 -> [w372 _ _ _ _ _ _ _ _ _ _ _ _ _ w1382 _ _ _ _ w1590 _ w1627 w1663 _ w1809]
      tunnel: w353 -> [w371 _ _ _ _ _ _ _ _ _ _ _ _ _ w1381 _ _ _ _ w1589 _ w1626 w1662 _ w1808]
      tunnel: [w370 _ _ _ _ _ _ _ _ _ _ _ _ _ w1379 _ _ _ _ w1588 _ w1625 w1661 _ w1805] -> w352
      tunnel: [w369 _ _ _ _ _ _ _ _ _ _ _ _ _ w1380 _ _ _ _ w1587 _ w1624 w1660 _ w1804] -> w351
      event #0 {
        n144 = event-data() -> ()  [unwired: 1 in, 2 out]
        n145 = flat-sequence {
          tunnel: [w768] -> w419
          tunnel: [w744] -> w418
          tunnel: [w757] -> w417
          tunnel: [w735] -> w416
          tunnel: w406 -> [w734]
          tunnel: w405 -> [w733]
          tunnel: w419 -> [w774]
          tunnel: [w774] -> w415
          tunnel: w418 -> [w773]
          tunnel: [w773] -> w414
          tunnel: w417 -> [w772]
          tunnel: [w772] -> w413
          tunnel: w416 -> [w769]
          tunnel: [w769] -> w412
          tunnel: w415 -> [w781]
          tunnel: [w782] -> w411
          tunnel: w414 -> [w784]
          tunnel: [w783] -> w410
          tunnel: w413 -> [w780]
          tunnel: [w779] -> w409
          tunnel: w412 -> [w779]
          tunnel: w411 -> [w794]
          tunnel: w410 -> [w795]
          tunnel: [w793] -> w408
          tunnel: w409 -> [w797]
          tunnel: [w792] -> w407
          tunnel: [w880] -> w403
          tunnel: w408 -> [w880]
          tunnel: w407 -> [w860]
          tunnel: [w860] -> w404
          frame #0 {
            w739 = 0.1 ("Delay Time (s)")
            n146 = property on="X Step SP" class="DigNum (strict)"() -> ("Maximum"=w759:dbl)  [unwired: 2 in, 2 out]
            n147 = property on="X Step SP" class="DigNum (strict)"() -> ("Minimum"=w761:dbl)  [unwired: 2 in, 2 out]
            n148 = property on="X steps/rev" class="DigNum (strict)"() -> ("Value"=w755:u32)  [unwired: 2 in, 2 out]
            n149 = property on="X offset mm" class="DigNum (strict)"() -> ("Value"=w751:dbl)  [unwired: 2 in, 2 out]
            n150 = call "mDrive Send Command.vi"("error in (no error)"=w733, "Extra"="P", "Command"=T2."Print Parameter", "VISA resource name"=w734) -> ("error out"=w763:errorcluster, "read buffer"=w767:string, "VISA resource name out"=w765:refnum<visa-resource-name>)  [unwired: 3 in]
            n151 = call "Time Delay12"("error in (no error)"=w763, "Delay Time (s)"=w739) -> ("error out"=w762:errorcluster)  [unwired: 9 in]
            n152 = Decimal String To Number(string=w767, offset=0) -> (number=w747:i32)  [unwired: 1 in, 1 out]
            n153 = To Long Integer(number=w747) -> (32bit integer=w749:i32)
            n154 = property on="X Step PV" class="DigNum (strict)"("Val(Sgnl)"=w749) -> ()  [unwired: 2 in, 2 out]
            n155 = To Long Integer(number=w759) -> (32bit integer=w758:i32)
            n156 = To Long Integer(number=w761) -> (32bit integer=w760:i32)
            n157 = call "mDrive Send Command.vi"("error in (no error)"=w762, "Extra"="MV", "Command"=T2."Print Parameter", "VISA resource name"=w765) -> ("error out"=w764:errorcluster, "read buffer"=w745:string, "VISA resource name out"=w768:refnum<visa-resource-name>)  [unwired: 3 in]
            n158 = call "Time Delay11"("error in (no error)"=w764, "Delay Time (s)"=w739) -> ("error out"=w744:errorcluster)  [unwired: 9 in]
            n159 = In Range and Coerce(upper limit=w758, x=w749, lower limit=w760) -> (In Range?=w757:bool)  [unwired: 1 out]
            n160 = To Double Precision Float(number=w749) -> (double precision float=w750:dbl)
            n161 = To Double Precision Float(number=w755) -> (double precision float=w756:dbl)
            n162 = Decimal String To Number(string=w745, offset=0 ("offset (0)")) -> (number=w738:i32)  [unwired: 1 in, 1 out]
            n163 = property on="X  in Range" class="Bool (strict)"("Val(Sgnl)"=w757) -> ()  [unwired: 2 in, 2 out]
            n164 = Divide(x=w750, y=w756) -> (x/y=w754:dbl)
            n165 = Number To Boolean Array(number=w738) -> (Boolean array=w737:bool[])
            n166 = property on="X mm/rev" class="DigNum (strict)"() -> ("Value"=w753:dbl)  [unwired: 2 in, 2 out]
            n167 = Index Array(array=w737, index=0) -> (element=w735:bool)
            n168 = property on="X  in Motion" class="Bool (strict)"("Val(Sgnl)"=w735) -> ()  [unwired: 2 in, 2 out]
            n169 = Multiply(x=w754, y=w753) -> (x*y=w752:dbl)
            n170 = Add(x=w752, y=w751) -> (x+y=w748:dbl)
            n171 = property on="X Position mm PV" class="DigNum (strict)"("Val(Sgnl)"=w748) -> ()  [unwired: 2 in, 2 out]
          }
          frame #1 {
            n172 = property on="X Scan" class="Bool (strict)"() -> ("Value"=w770:bool)  [unwired: 2 in, 2 out]
            n173 = Or(x=w769, y=w770) -> (x .or. y?=w771:bool)
            n174 = case shown="False" w771 {
              frame #0 {
                n175 = property on="X Go" class="Bool"("DisabledEnum"=T1."Enabled" ("Disabled")) -> ()  [unwired: 2 in, 2 out]
                n176 = property on="X Scan OK" class="Bool"("DisabledEnum"=T1."Enabled" ("Disabled")) -> ()  [unwired: 2 in, 2 out]
              }
              frame #1 {
                n177 = property on="X Go" class="Bool"("DisabledEnum"=T1."Disabled and Grayed Out" ("Disabled")) -> ()  [unwired: 2 in, 2 out]
                n178 = property on="X Scan set" class="Bool"("DisabledEnum"=T1."Disabled and Grayed Out" ("Disabled")) -> ()  [unwired: 2 in, 2 out]
              }
            }
          }
          frame #2 {
            n179 = case shown="False" w780 {
              tunnel: w781 -> [w787 w791]
              tunnel: [w788 w791] -> w782
              tunnel: [w789 w790] -> w783
              tunnel: w784 -> [w786 w790]
              frame #0 {
                n180 = call "mDrive Send Command.vi"("error in (no error)"=w786, "Command"=T2."Stop", "VISA resource name"=w787) -> ("error out"=w789:errorcluster, "VISA resource name out"=w788:refnum<visa-resource-name>)  [unwired: 4 in, 1 out]
              }
              frame #1 {
              }
            }
          }
          frame #3 {
            n181 = property on="X Backlash corr" class="Bool (strict)"() -> ("Value"=w798:bool)  [unwired: 2 in, 2 out]
            n182 = Implies(1:w797, 2:w798) -> (0:w796:bool)
            n183 = case shown="False" w796 {
              tunnel: w795 -> [w805 w858]
              tunnel: w794 -> [w804 w859]
              tunnel: [w803 w858] -> w793
              tunnel: [w802 w859] -> w792
              frame #0 {
                # "Backlash"
                n184 = flat-sequence {
                  tunnel: [w820] -> w817
                  tunnel: [w822] -> w816
                  tunnel: [w821] -> w815
                  tunnel: w805 -> [w819]
                  tunnel: w804 -> [w818]
                  tunnel: w817 -> [w830]
                  tunnel: [w830] -> w814
                  tunnel: w816 -> [w829]
                  tunnel: w815 -> [w828]
                  tunnel: [w827] -> w813
                  tunnel: [w826] -> w812
                  tunnel: [w825] -> w801
                  tunnel: w814 -> [w840]
                  tunnel: w813 -> [w839]
                  tunnel: w812 -> [w837]
                  tunnel: [w838] -> w811
                  tunnel: [w837] -> w810
                  tunnel: [w836] -> w807
                  tunnel: [w835] -> w806
                  tunnel: w801 -> [w835]
                  tunnel: w811 -> [w851]
                  tunnel: w810 -> [w844]
                  tunnel: [w851] -> w809
                  tunnel: [w850] -> w808
                  tunnel: w807 -> [w850]
                  tunnel: w806 -> [w846]
                  tunnel: [w845] -> w799
                  tunnel: w809 -> [w855]
                  tunnel: w808 -> [w854]
                  tunnel: [w853] -> w803
                  tunnel: [w852] -> w800
                  tunnel: w799 -> [w852]
                  tunnel: [w857] -> w802
                  tunnel: w800 -> [w857]
                  frame #0 {
                    n185 = property on="X Backlash steps/sec" class="DigNum (strict)"() -> ("Value"=w820:i32)  [unwired: 2 in, 2 out]
                    n186 = Number To Decimal String(number=w820) -> (decimal integer string=w823:string)  [unwired: 1 in]
                    n187 = call "mDrive Send Command.vi"("error in (no error)"=w819, "Extra"=w823, "Command"=T2."Max Velocity", "VISA resource name"=w818) -> ("error out"=w821:errorcluster, "VISA resource name out"=w822:refnum<visa-resource-name>)  [unwired: 3 in, 1 out]
                  }
                  frame #1 {
                    n188 = property on="X Backlash" class="DigNum (strict)"() -> ("Value"=w825:i32)  [unwired: 2 in, 2 out]
                    n189 = Number To Decimal String(number=w825) -> (decimal integer string=w831:string)  [unwired: 1 in]
                    n190 = call "mDrive Send Command.vi"("error in (no error)"=w828, "Extra"=w831, "Command"=T2."Move to Relative Position", "VISA resource name"=w829) -> ("error out"=w827:errorcluster, "VISA resource name out"=w826:refnum<visa-resource-name>)  [unwired: 3 in, 1 out]
                  }
                  frame #2 {
                    n191 = To Double Precision Float(number=w835) -> (double precision float=w833:dbl)
                    n192 = To Double Precision Float(number=w840) -> (double precision float=w842:dbl)
                    n193 = Absolute Value(x=w833) -> (abs(x)=w834:dbl)
                    n194 = Divide(x=w834, y=w842) -> (x/y=w843:dbl)
                    n195 = Add(x=w843, y=0.3) -> (x+y=w836:dbl)
                    n196 = call "Time Delay13"("error in (no error)"=w839, "Delay Time (s)"=w836) -> ("error out"=w838:errorcluster)  [unwired: 9 in]
                  }
                  frame #3 {
                    n197 = Negate(x=w846) -> (-x=w847:i32)
                    n198 = Number To Decimal String(number=w847) -> (decimal integer string=w848:string)  [unwired: 1 in]
                    n199 = call "mDrive Send Command.vi"("Extra"=w848, "Command"=T2."Move to Relative Position", "VISA resource name"=w844) -> ("VISA resource name out"=w845:refnum<visa-resource-name>)  [unwired: 4 in, 2 out]
                  }
                  frame #4 {
                    n200 = call "Time Delay14"("error in (no error)"=w855, "Delay Time (s)"=w854) -> ("error out"=w853:errorcluster)  [unwired: 9 in]
                  }
                  frame #5 {
                    n201 = property on="X Backlash corr" class="Bool (strict)"("Val(Sgnl)"=FALSE ("Value (Signaling)")) -> ()  [unwired: 2 in, 2 out]
                  }
                }
              }
              frame #1 {
              }
            }
          }
          frame #4 {
            n202 = property on="X Step PV" class="DigNum (strict)"() -> ("Value"=w870:i32)  [unwired: 2 in, 2 out]
            n203 = property on="X Step PV" class="DigNum (strict)"() -> ("Value"=w868:i32)  [unwired: 2 in, 2 out]
            n204 = property on="X steps/rev" class="DigNum (strict)"() -> ("Value"=w872:u32)  [unwired: 2 in, 2 out]
            n205 = To Double Precision Float(number=w872) -> (double precision float=w866:dbl)
            n206 = property on="X Step SP" class="DigNum (strict)"() -> ("Maximum"=w877:dbl)  [unwired: 2 in, 2 out]
            n207 = property on="X Step SP" class="DigNum (strict)"() -> ("Minimum"=w878:dbl)  [unwired: 2 in, 2 out]
            n208 = To Double Precision Float(number=w868) -> (double precision float=w867:dbl)
            n209 = To Double Precision Float(number=w870) -> (double precision float=w869:dbl)
            n210 = Subtract(x=w877, y=w869) -> (x-y=w876:dbl)
            n211 = Subtract(x=w878, y=w867) -> (x-y=w879:dbl)
            n212 = property on="X Scan Length SP steps" class="DigNum (strict)"() -> ("Value"=w865:i32)  [unwired: 2 in, 2 out]
            n213 = property on="X Scan Velocity SP steps/sec" class="DigNum (strict)"() -> ("Value"=w874:i32)  [unwired: 2 in, 2 out]
            n214 = To Double Precision Float(number=w865) -> (double precision float=w864:dbl)
            n215 = property on="X Scan Length SP steps" class="DigNum (strict)"("Maximum"=w876) -> ()  [unwired: 2 in, 2 out]
            n216 = property on="X Scan Length SP steps" class="DigNum (strict)"("Minimum"=w879) -> ()  [unwired: 2 in, 2 out]
            n217 = Divide(x=w864, y=w866) -> (x/y=w863:dbl)
            n218 = To Double Precision Float(number=w874) -> (double precision float=w873:dbl)
            n219 = property on="X mm/rev" class="DigNum (strict)"() -> ("Value"=w871:dbl)  [unwired: 2 in, 2 out]
            n220 = Divide(x=w873, y=w866) -> (x/y=w875:dbl)
            n221 = Multiply(x=w871, y=w863) -> (x*y=w861:dbl)
            n222 = Multiply(x=w875, y=w871) -> (x*y=w862:dbl)
            n223 = property on="X Scan length MV mm" class="DigNum (strict)"("Val(Sgnl)"=w861) -> ()  [unwired: 2 in, 2 out]
            n224 = property on="X Scan velocity MV mm/sec" class="DigNum (strict)"("Value"=w862) -> ()  [unwired: 2 in, 2 out]
          }
        }
        n225 = flat-sequence {
          tunnel: w436 -> [w911]
          tunnel: w433 -> [w910]
          tunnel: [w916] -> w432
          tunnel: [w890] -> w430
          tunnel: [w903] -> w428
          tunnel: [w881] -> w426
          tunnel: w432 -> [w922]
          tunnel: [w922] -> w431
          tunnel: w430 -> [w921]
          tunnel: [w921] -> w429
          tunnel: w428 -> [w920]
          tunnel: [w920] -> w427
          tunnel: w426 -> [w917]
          tunnel: [w917] -> w421
          tunnel: w431 -> [w929]
          tunnel: [w930] -> w425
          tunnel: w429 -> [w932]
          tunnel: [w931] -> w424
          tunnel: w427 -> [w928]
          tunnel: [w927] -> w422
          tunnel: w421 -> [w927]
          tunnel: w425 -> [w942]
          tunnel: w424 -> [w943]
          tunnel: [w941] -> w423
          tunnel: w422 -> [w945]
          tunnel: [w940] -> w420
          tunnel: [w1027] -> w435
          tunnel: [w1028] -> w434
          tunnel: w423 -> [w1027]
          tunnel: w420 -> [w1028]
          frame #0 {
            w885 = 0.1 ("Delay Time (s)")
            n226 = property on="Y Step SP" class="DigNum (strict)"() -> ("Maximum"=w905:dbl)  [unwired: 2 in, 2 out]
            n227 = property on="Y Step SP" class="DigNum (strict)"() -> ("Minimum"=w907:dbl)  [unwired: 2 in, 2 out]
            n228 = property on="Y steps/rev" class="DigNum (strict)"() -> ("Value"=w901:u32)  [unwired: 2 in, 2 out]
            n229 = property on="Y offset mm" class="DigNum (strict)"() -> ("Value"=w897:dbl)  [unwired: 2 in, 2 out]
            n230 = call "mDrive Send Command.vi"("error in (no error)"=w911, "Extra"="P", "Command"=T2."Print Parameter", "VISA resource name"=w910) -> ("error out"=w909:errorcluster, "read buffer"=w915:string, "VISA resource name out"=w913:refnum<visa-resource-name>)  [unwired: 3 in]
            n231 = call "Time Delay4"("error in (no error)"=w909, "Delay Time (s)"=w885) -> ("error out"=w908:errorcluster)  [unwired: 9 in]
            n232 = Decimal String To Number(string=w915, offset=0) -> (number=w893:i32)  [unwired: 1 in, 1 out]
            n233 = To Long Integer(number=w893) -> (32bit integer=w895:i32)
            n234 = property on="Y Step PV" class="DigNum (strict)"("Val(Sgnl)"=w895) -> ()  [unwired: 2 in, 2 out]
            n235 = To Long Integer(number=w905) -> (32bit integer=w904:i32)
            n236 = To Long Integer(number=w907) -> (32bit integer=w906:i32)
            n237 = call "mDrive Send Command.vi"("error in (no error)"=w908, "Extra"="MV", "Command"=T2."Print Parameter", "VISA resource name"=w913) -> ("error out"=w912:errorcluster, "read buffer"=w891:string, "VISA resource name out"=w916:refnum<visa-resource-name>)  [unwired: 3 in]
            n238 = call "Time Delay3"("error in (no error)"=w912, "Delay Time (s)"=w885) -> ("error out"=w890:errorcluster)  [unwired: 9 in]
            n239 = In Range and Coerce(upper limit=w904, x=w895, lower limit=w906) -> (In Range?=w903:bool)  [unwired: 1 out]
            n240 = To Double Precision Float(number=w895) -> (double precision float=w896:dbl)
            n241 = To Double Precision Float(number=w901) -> (double precision float=w902:dbl)
            n242 = Decimal String To Number(string=w891, offset=0 ("offset (0)")) -> (number=w884:i32)  [unwired: 1 in, 1 out]
            n243 = property on="Y in Range" class="Bool (strict)"("Val(Sgnl)"=w903) -> ()  [unwired: 2 in, 2 out]
            n244 = Divide(x=w896, y=w902) -> (x/y=w900:dbl)
            n245 = Number To Boolean Array(number=w884) -> (Boolean array=w883:bool[])
            n246 = property on="Y mm/rev" class="DigNum (strict)"() -> ("Value"=w899:dbl)  [unwired: 2 in, 2 out]
            n247 = Index Array(array=w883, index=0) -> (element=w881:bool)
            n248 = property on="Y in Motion" class="Bool (strict)"("Val(Sgnl)"=w881) -> ()  [unwired: 2 in, 2 out]
            n249 = Multiply(x=w900, y=w899) -> (x*y=w898:dbl)
            n250 = Add(x=w898, y=w897) -> (x+y=w894:dbl)
            n251 = property on="Y Position mm PV" class="DigNum (strict)"("Val(Sgnl)"=w894) -> ()  [unwired: 2 in, 2 out]
          }
          frame #1 {
            n252 = property on="Y Scan" class="Bool (strict)"() -> ("Value"=w918:bool)  [unwired: 2 in, 2 out]
            n253 = Or(x=w917, y=w918) -> (x .or. y?=w919:bool)
            n254 = case shown="True" w919 {
              frame #0 {
                n255 = property on="Y Go" class="Bool"("DisabledEnum"=T1."Enabled" ("Disabled")) -> ()  [unwired: 2 in, 2 out]
                n256 = property on="Y Scan OK" class="Bool"("DisabledEnum"=T1."Enabled" ("Disabled")) -> ()  [unwired: 2 in, 2 out]
              }
              frame #1 {
                n257 = property on="Y Go" class="Bool"("DisabledEnum"=T1."Disabled and Grayed Out" ("Disabled")) -> ()  [unwired: 2 in, 2 out]
                n258 = property on="Y Scan OK" class="Bool"("DisabledEnum"=T1."Disabled and Grayed Out" ("Disabled")) -> ()  [unwired: 2 in, 2 out]
              }
            }
          }
          frame #2 {
            n259 = case shown="False" w928 {
              tunnel: w929 -> [w935 w939]
              tunnel: [w936 w939] -> w930
              tunnel: [w937 w938] -> w931
              tunnel: w932 -> [w934 w938]
              frame #0 {
                n260 = call "mDrive Send Command.vi"("error in (no error)"=w934, "Command"=T2."Stop", "VISA resource name"=w935) -> ("error out"=w937:errorcluster, "VISA resource name out"=w936:refnum<visa-resource-name>)  [unwired: 4 in, 1 out]
              }
              frame #1 {
              }
            }
          }
          frame #3 {
            n261 = property on="Y Backlash corr" class="Bool (strict)"() -> ("Value"=w946:bool)  [unwired: 2 in, 2 out]
            n262 = Implies(1:w945, 2:w946) -> (0:w944:bool)
            n263 = case shown="False" w944 {
              tunnel: w943 -> [w953 w1006]
              tunnel: w942 -> [w952 w1007]
              tunnel: [w951 w1006] -> w941
              tunnel: [w950 w1007] -> w940
              frame #0 {
                # "Backlash"
                n264 = flat-sequence {
                  tunnel: [w968] -> w965
                  tunnel: [w970] -> w964
                  tunnel: [w969] -> w963
                  tunnel: w953 -> [w967]
                  tunnel: w952 -> [w966]
                  tunnel: w965 -> [w978]
                  tunnel: [w978] -> w962
                  tunnel: w964 -> [w977]
                  tunnel: w963 -> [w976]
                  tunnel: [w975] -> w961
                  tunnel: [w974] -> w960
                  tunnel: [w973] -> w949
                  tunnel: w962 -> [w988]
                  tunnel: w961 -> [w987]
                  tunnel: w960 -> [w985]
                  tunnel: [w986] -> w959
                  tunnel: [w985] -> w958
                  tunnel: [w984] -> w955
                  tunnel: [w983] -> w954
                  tunnel: w949 -> [w983]
                  tunnel: w959 -> [w999]
                  tunnel: w958 -> [w992]
                  tunnel: [w999] -> w957
                  tunnel: [w998] -> w956
                  tunnel: w955 -> [w998]
                  tunnel: w954 -> [w994]
                  tunnel: [w993] -> w947
                  tunnel: w957 -> [w1003]
                  tunnel: w956 -> [w1002]
                  tunnel: [w1001] -> w951
                  tunnel: [w1000] -> w948
                  tunnel: w947 -> [w1000]
                  tunnel: [w1005] -> w950
                  tunnel: w948 -> [w1005]
                  frame #0 {
                    n265 = property on="Y Backlash steps/sec" class="DigNum (strict)"() -> ("Value"=w968:i32)  [unwired: 2 in, 2 out]
                    n266 = Number To Decimal String(number=w968) -> (decimal integer string=w971:string)  [unwired: 1 in]
                    n267 = call "mDrive Send Command.vi"("error in (no error)"=w967, "Extra"=w971, "Command"=T2."Max Velocity", "VISA resource name"=w966) -> ("error out"=w969:errorcluster, "VISA resource name out"=w970:refnum<visa-resource-name>)  [unwired: 3 in, 1 out]
                  }
                  frame #1 {
                    n268 = property on="Y Backlash" class="DigNum (strict)"() -> ("Value"=w973:i32)  [unwired: 2 in, 2 out]
                    n269 = Number To Decimal String(number=w973) -> (decimal integer string=w979:string)  [unwired: 1 in]
                    n270 = call "mDrive Send Command.vi"("error in (no error)"=w976, "Extra"=w979, "Command"=T2."Move to Relative Position", "VISA resource name"=w977) -> ("error out"=w975:errorcluster, "VISA resource name out"=w974:refnum<visa-resource-name>)  [unwired: 3 in, 1 out]
                  }
                  frame #2 {
                    n271 = To Double Precision Float(number=w983) -> (double precision float=w981:dbl)
                    n272 = To Double Precision Float(number=w988) -> (double precision float=w990:dbl)
                    n273 = Absolute Value(x=w981) -> (abs(x)=w982:dbl)
                    n274 = Divide(x=w982, y=w990) -> (x/y=w991:dbl)
                    n275 = Add(x=w991, y=0.3) -> (x+y=w984:dbl)
                    n276 = call "Time Delay8"("error in (no error)"=w987, "Delay Time (s)"=w984) -> ("error out"=w986:errorcluster)  [unwired: 9 in]
                  }
                  frame #3 {
                    n277 = Negate(x=w994) -> (-x=w995:i32)
                    n278 = Number To Decimal String(number=w995) -> (decimal integer string=w996:string)  [unwired: 1 in]
                    n279 = call "mDrive Send Command.vi"("Extra"=w996, "Command"=T2."Move to Relative Position", "VISA resource name"=w992) -> ("VISA resource name out"=w993:refnum<visa-resource-name>)  [unwired: 4 in, 2 out]
                  }
                  frame #4 {
                    n280 = call "Time Delay2"("error in (no error)"=w1003, "Delay Time (s)"=w1002) -> ("error out"=w1001:errorcluster)  [unwired: 9 in]
                  }
                  frame #5 {
                    n281 = property on="Y Backlash corr" class="Bool (strict)"("Val(Sgnl)"=FALSE ("Value (Signaling)")) -> ()  [unwired: 2 in, 2 out]
                  }
                }
              }
              frame #1 {
              }
            }
          }
          frame #4 {
            n282 = property on="Y Step PV" class="DigNum (strict)"() -> ("Value"=w1017:i32)  [unwired: 2 in, 2 out]
            n283 = property on="Y Step PV" class="DigNum (strict)"() -> ("Value"=w1015:i32)  [unwired: 2 in, 2 out]
            n284 = property on="Y steps/rev" class="DigNum (strict)"() -> ("Value"=w1019:u32)  [unwired: 2 in, 2 out]
            n285 = To Double Precision Float(number=w1019) -> (double precision float=w1013:dbl)
            n286 = property on="Y Step SP" class="DigNum (strict)"() -> ("Maximum"=w1024:dbl)  [unwired: 2 in, 2 out]
            n287 = property on="Y Step SP" class="DigNum (strict)"() -> ("Minimum"=w1025:dbl)  [unwired: 2 in, 2 out]
            n288 = To Double Precision Float(number=w1015) -> (double precision float=w1014:dbl)
            n289 = To Double Precision Float(number=w1017) -> (double precision float=w1016:dbl)
            n290 = Subtract(x=w1024, y=w1016) -> (x-y=w1023:dbl)
            n291 = Subtract(x=w1025, y=w1014) -> (x-y=w1026:dbl)
            n292 = property on="Y Scan Length SP steps" class="DigNum (strict)"() -> ("Value"=w1021:i32)  [unwired: 2 in, 2 out]
            n293 = property on="Y Scan Velocity SP steps/sec" class="DigNum (strict)"() -> ("Value"=w1012:i32)  [unwired: 2 in, 2 out]
            n294 = To Double Precision Float(number=w1021) -> (double precision float=w1020:dbl)
            n295 = property on="Y Scan Length SP steps" class="DigNum (strict)"("Maximum"=w1023) -> ()  [unwired: 2 in, 2 out]
            n296 = property on="Y Scan Length SP steps" class="DigNum (strict)"("Minimum"=w1026) -> ()  [unwired: 2 in, 2 out]
            n297 = Divide(x=w1020, y=w1013) -> (x/y=w1022:dbl)
            n298 = To Double Precision Float(number=w1012) -> (double precision float=w1011:dbl)
            n299 = property on="Y mm/rev" class="DigNum (strict)"() -> ("Value"=w1018:dbl)  [unwired: 2 in, 2 out]
            n300 = Multiply(x=w1022, y=w1018) -> (x*y=w1009:dbl)
            n301 = Divide(x=w1011, y=w1013) -> (x/y=w1010:dbl)
            n302 = Multiply(x=w1018, y=w1010) -> (x*y=w1008:dbl)
            n303 = property on="Y Scan length MV mm" class="DigNum (strict)"("Value"=w1009) -> ()  [unwired: 2 in, 2 out]
            n304 = property on="Y Scan velocity MV mm/sec" class="DigNum (strict)"("Val(Sgnl)"=w1008) -> ()  [unwired: 2 in, 2 out]
          }
        }
        n305 = flat-sequence {
          tunnel: [w620] -> w402
          tunnel: [w596] -> w401
          tunnel: [w609] -> w400
          tunnel: [w587] -> w399
          tunnel: w373 -> [w586]
          tunnel: w376 -> [w585]
          tunnel: w402 -> [w626]
          tunnel: [w626] -> w398
          tunnel: w401 -> [w625]
          tunnel: [w625] -> w397
          tunnel: w400 -> [w624]
          tunnel: [w624] -> w396
          tunnel: w399 -> [w621]
          tunnel: [w621] -> w395
          tunnel: w398 -> [w633]
          tunnel: [w634] -> w394
          tunnel: w397 -> [w636]
          tunnel: [w635] -> w393
          tunnel: w396 -> [w632]
          tunnel: [w631] -> w392
          tunnel: w395 -> [w631]
          tunnel: w394 -> [w646]
          tunnel: w393 -> [w647]
          tunnel: [w645] -> w391
          tunnel: w392 -> [w649]
          tunnel: [w644] -> w390
          tunnel: [w732] -> w374
          tunnel: w391 -> [w732]
          tunnel: w390 -> [w712]
          tunnel: [w712] -> w375
          frame #0 {
            w591 = 0.1 ("Delay Time (s)")
            n306 = property on="Z Step SP" class="DigNum (strict)"() -> ("Maximum"=w611:dbl)  [unwired: 2 in, 2 out]
            n307 = property on="Z Step SP" class="DigNum (strict)"() -> ("Minimum"=w613:dbl)  [unwired: 2 in, 2 out]
            n308 = property on="Z steps/rev" class="DigNum (strict)"() -> ("Value"=w607:u32)  [unwired: 2 in, 2 out]
            n309 = property on="Z offset mm" class="DigNum (strict)"() -> ("Value"=w603:dbl)  [unwired: 2 in, 2 out]
            n310 = To Long Integer(number=w611) -> (32bit integer=w610:i32)
            n311 = To Long Integer(number=w613) -> (32bit integer=w612:i32)
            n312 = To Double Precision Float(number=w607) -> (double precision float=w608:dbl)
            n313 = call "mDrive Send Command.vi"("error in (no error)"=w585, "Extra"="P", "Command"=T2."Print Parameter", "VISA resource name"=w586) -> ("error out"=w615:errorcluster, "read buffer"=w619:string, "VISA resource name out"=w617:refnum<visa-resource-name>)  [unwired: 3 in]
            n314 = call "Time Delay17"("error in (no error)"=w615, "Delay Time (s)"=w591) -> ("error out"=w614:errorcluster)  [unwired: 9 in]
            n315 = Decimal String To Number(string=w619, offset=0) -> (number=w599:i32)  [unwired: 1 in, 1 out]
            n316 = To Long Integer(number=w599) -> (32bit integer=w601:i32)
            n317 = property on="Z Step PV" class="DigNum (strict)"("Val(Sgnl)"=w601) -> ()  [unwired: 2 in, 2 out]
            n318 = call "mDrive Send Command.vi"("error in (no error)"=w614, "Extra"="MV", "Command"=T2."Print Parameter", "VISA resource name"=w617) -> ("error out"=w616:errorcluster, "read buffer"=w597:string, "VISA resource name out"=w620:refnum<visa-resource-name>)  [unwired: 3 in]
            n319 = call "Time Delay16"("error in (no error)"=w616, "Delay Time (s)"=w591) -> ("error out"=w596:errorcluster)  [unwired: 9 in]
            n320 = In Range and Coerce(upper limit=w610, x=w601, lower limit=w612) -> (In Range?=w609:bool)  [unwired: 1 out]
            n321 = To Double Precision Float(number=w601) -> (double precision float=w602:dbl)
            n322 = Decimal String To Number(string=w597, offset=0 ("offset (0)")) -> (number=w590:i32)  [unwired: 1 in, 1 out]
            n323 = property on="Z in Range" class="Bool (strict)"("Val(Sgnl)"=w609) -> ()  [unwired: 2 in, 2 out]
            n324 = Divide(x=w602, y=w608) -> (x/y=w606:dbl)
            n325 = Number To Boolean Array(number=w590) -> (Boolean array=w589:bool[])
            n326 = property on="Z mm/rev" class="DigNum (strict)"() -> ("Value"=w605:dbl)  [unwired: 2 in, 2 out]
            n327 = Index Array(array=w589, index=0) -> (element=w587:bool)
            n328 = property on="Z in Motion" class="Bool (strict)"("Val(Sgnl)"=w587) -> ()  [unwired: 2 in, 2 out]
            n329 = Multiply(x=w606, y=w605) -> (x*y=w604:dbl)
            n330 = Add(x=w604, y=w603) -> (x+y=w600:dbl)
            n331 = property on="Z Position mm PV" class="DigNum (strict)"("Val(Sgnl)"=w600) -> ()  [unwired: 2 in, 2 out]
          }
          frame #1 {
            n332 = property on="Z Scan" class="Bool (strict)"() -> ("Value"=w622:bool)  [unwired: 2 in, 2 out]
            n333 = Or(x=w621, y=w622) -> (x .or. y?=w623:bool)
            n334 = case shown="True" w623 {
              frame #0 {
                n335 = property on="Z Go" class="Bool"("DisabledEnum"=T1."Enabled" ("Disabled")) -> ()  [unwired: 2 in, 2 out]
                n336 = property on="Z Scan OK" class="Bool"("DisabledEnum"=T1."Enabled" ("Disabled")) -> ()  [unwired: 2 in, 2 out]
              }
              frame #1 {
                n337 = property on="Z Go" class="Bool"("DisabledEnum"=T1."Disabled and Grayed Out" ("Disabled")) -> ()  [unwired: 2 in, 2 out]
                n338 = property on="Z Scan OK" class="Bool"("DisabledEnum"=T1."Disabled and Grayed Out" ("Disabled")) -> ()  [unwired: 2 in, 2 out]
              }
            }
          }
          frame #2 {
            n339 = case shown="False" w632 {
              tunnel: w633 -> [w639 w643]
              tunnel: [w640 w643] -> w634
              tunnel: [w641 w642] -> w635
              tunnel: w636 -> [w638 w642]
              frame #0 {
                n340 = call "mDrive Send Command.vi"("error in (no error)"=w638, "Command"=T2."Stop", "VISA resource name"=w639) -> ("error out"=w641:errorcluster, "VISA resource name out"=w640:refnum<visa-resource-name>)  [unwired: 4 in, 1 out]
              }
              frame #1 {
              }
            }
          }
          frame #3 {
            n341 = property on="Z Backlash corr" class="Bool (strict)"() -> ("Value"=w650:bool)  [unwired: 2 in, 2 out]
            n342 = Implies(1:w649, 2:w650) -> (0:w648:bool)
            n343 = case shown="False" w648 {
              tunnel: w647 -> [w657 w710]
              tunnel: w646 -> [w656 w711]
              tunnel: [w655 w710] -> w645
              tunnel: [w654 w711] -> w644
              frame #0 {
                # "Backlash"
                n344 = flat-sequence {
                  tunnel: [w672] -> w669
                  tunnel: [w674] -> w668
                  tunnel: [w673] -> w667
                  tunnel: w657 -> [w671]
                  tunnel: w656 -> [w670]
                  tunnel: w669 -> [w682]
                  tunnel: [w682] -> w666
                  tunnel: w668 -> [w681]
                  tunnel: w667 -> [w680]
                  tunnel: [w679] -> w665
                  tunnel: [w678] -> w664
                  tunnel: [w677] -> w653
                  tunnel: w666 -> [w692]
                  tunnel: w665 -> [w691]
                  tunnel: w664 -> [w689]
                  tunnel: [w690] -> w663
                  tunnel: [w689] -> w662
                  tunnel: [w688] -> w659
                  tunnel: [w687] -> w658
                  tunnel: w653 -> [w687]
                  tunnel: w663 -> [w703]
                  tunnel: w662 -> [w696]
                  tunnel: [w703] -> w661
                  tunnel: [w702] -> w660
                  tunnel: w659 -> [w702]
                  tunnel: w658 -> [w698]
                  tunnel: [w697] -> w651
                  tunnel: w661 -> [w707]
                  tunnel: w660 -> [w706]
                  tunnel: [w705] -> w655
                  tunnel: [w704] -> w652
                  tunnel: w651 -> [w704]
                  tunnel: [w709] -> w654
                  tunnel: w652 -> [w709]
                  frame #0 {
                    n345 = property on="Z Backlash steps/sec" class="DigNum (strict)"() -> ("Value"=w672:i32)  [unwired: 2 in, 2 out]
                    n346 = Number To Decimal String(number=w672) -> (decimal integer string=w675:string)  [unwired: 1 in]
                    n347 = call "mDrive Send Command.vi"("error in (no error)"=w671, "Extra"=w675, "Command"=T2."Max Velocity", "VISA resource name"=w670) -> ("error out"=w673:errorcluster, "VISA resource name out"=w674:refnum<visa-resource-name>)  [unwired: 3 in, 1 out]
                  }
                  frame #1 {
                    n348 = property on="Z Backlash" class="DigNum (strict)"() -> ("Value"=w677:i32)  [unwired: 2 in, 2 out]
                    n349 = Number To Decimal String(number=w677) -> (decimal integer string=w683:string)  [unwired: 1 in]
                    n350 = call "mDrive Send Command.vi"("error in (no error)"=w680, "Extra"=w683, "Command"=T2."Move to Relative Position", "VISA resource name"=w681) -> ("error out"=w679:errorcluster, "VISA resource name out"=w678:refnum<visa-resource-name>)  [unwired: 3 in, 1 out]
                  }
                  frame #2 {
                    n351 = To Double Precision Float(number=w687) -> (double precision float=w685:dbl)
                    n352 = To Double Precision Float(number=w692) -> (double precision float=w694:dbl)
                    n353 = Absolute Value(x=w685) -> (abs(x)=w686:dbl)
                    n354 = Divide(x=w686, y=w694) -> (x/y=w695:dbl)
                    n355 = Add(x=w695, y=0.3) -> (x+y=w688:dbl)
                    n356 = call "Time Delay18"("error in (no error)"=w691, "Delay Time (s)"=w688) -> ("error out"=w690:errorcluster)  [unwired: 9 in]
                  }
                  frame #3 {
                    n357 = Negate(x=w698) -> (-x=w699:i32)
                    n358 = Number To Decimal String(number=w699) -> (decimal integer string=w700:string)  [unwired: 1 in]
                    n359 = call "mDrive Send Command.vi"("Extra"=w700, "Command"=T2."Move to Relative Position", "VISA resource name"=w696) -> ("VISA resource name out"=w697:refnum<visa-resource-name>)  [unwired: 4 in, 2 out]
                  }
                  frame #4 {
                    n360 = call "Time Delay19"("error in (no error)"=w707, "Delay Time (s)"=w706) -> ("error out"=w705:errorcluster)  [unwired: 9 in]
                  }
                  frame #5 {
                    n361 = property on="Z Backlash corr" class="Bool (strict)"("Val(Sgnl)"=FALSE ("Value (Signaling)")) -> ()  [unwired: 2 in, 2 out]
                  }
                }
              }
              frame #1 {
              }
            }
          }
          frame #4 {
            n362 = property on="Z Step PV" class="DigNum (strict)"() -> ("Value"=w720:i32)  [unwired: 2 in, 2 out]
            n363 = property on="Z Step PV" class="DigNum (strict)"() -> ("Value"=w722:i32)  [unwired: 2 in, 2 out]
            n364 = property on="Z steps/rev" class="DigNum (strict)"() -> ("Value"=w724:u32)  [unwired: 2 in, 2 out]
            n365 = To Double Precision Float(number=w724) -> (double precision float=w718:dbl)
            n366 = property on="Z Step SP" class="DigNum (strict)"() -> ("Maximum"=w729:dbl)  [unwired: 2 in, 2 out]
            n367 = property on="Z Step SP" class="DigNum (strict)"() -> ("Minimum"=w730:dbl)  [unwired: 2 in, 2 out]
            n368 = To Double Precision Float(number=w720) -> (double precision float=w719:dbl)
            n369 = To Double Precision Float(number=w722) -> (double precision float=w721:dbl)
            n370 = Subtract(x=w730, y=w719) -> (x-y=w731:dbl)
            n371 = Subtract(x=w729, y=w721) -> (x-y=w728:dbl)
            n372 = property on="Z Velocity SP step/sec" class="DigNum (strict)"() -> ("Value"=w717:i32)  [unwired: 2 in, 2 out]
            n373 = property on="Z Scan Length SP steps" class="DigNum (strict)"() -> ("Value"=w726:i32)  [unwired: 2 in, 2 out]
            n374 = To Double Precision Float(number=w726) -> (double precision float=w725:dbl)
            n375 = To Double Precision Float(number=w717) -> (double precision float=w716:dbl)
            n376 = property on="Z Scan Length SP steps" class="DigNum (strict)"("Minimum"=w731) -> ()  [unwired: 2 in, 2 out]
            n377 = property on="Z Scan Length SP steps" class="DigNum (strict)"("Maximum"=w728) -> ()  [unwired: 2 in, 2 out]
            n378 = Divide(x=w725, y=w718) -> (x/y=w727:dbl)
            n379 = Divide(x=w716, y=w718) -> (x/y=w715:dbl)
            n380 = property on="Z mm/rev" class="DigNum (strict)"() -> ("Value"=w723:dbl)  [unwired: 2 in, 2 out]
            n381 = Multiply(x=w727, y=w723) -> (x*y=w714:dbl)
            n382 = Multiply(x=w723, y=w715) -> (x*y=w713:dbl)
            n383 = property on="Z Scan length MV mm" class="DigNum (strict)"("Value"=w714) -> ()  [unwired: 2 in, 2 out]
            n384 = property on="Z Scan velocity MV mm/sec" class="DigNum (strict)"("Val(Sgnl)"=w713) -> ()  [unwired: 2 in, 2 out]
          }
        }
        n385 = flat-sequence {
          tunnel: [w472] -> w389
          tunnel: [w448] -> w388
          tunnel: [w461] -> w387
          tunnel: [w439] -> w386
          tunnel: w372 -> [w438]
          tunnel: w371 -> [w437]
          tunnel: w389 -> [w478]
          tunnel: [w478] -> w385
          tunnel: w388 -> [w477]
          tunnel: [w477] -> w384
          tunnel: w387 -> [w476]
          tunnel: [w476] -> w383
          tunnel: w386 -> [w473]
          tunnel: [w473] -> w382
          tunnel: w385 -> [w485]
          tunnel: [w486] -> w381
          tunnel: w384 -> [w488]
          tunnel: [w487] -> w380
          tunnel: w383 -> [w484]
          tunnel: [w483] -> w379
          tunnel: w382 -> [w483]
          tunnel: w381 -> [w498]
          tunnel: w380 -> [w499]
          tunnel: [w497] -> w378
          tunnel: w379 -> [w501]
          tunnel: [w496] -> w377
          tunnel: [w584] -> w369
          tunnel: w378 -> [w584]
          tunnel: w377 -> [w564]
          tunnel: [w564] -> w370
          frame #0 {
            w443 = 0.1 ("Delay Time (s)")
            n386 = property on="R Step SP" class="DigNum (strict)"() -> ("Maximum"=w463:dbl)  [unwired: 2 in, 2 out]
            n387 = property on="R Step SP" class="DigNum (strict)"() -> ("Minimum"=w465:dbl)  [unwired: 2 in, 2 out]
            n388 = property on="R steps/rev" class="DigNum (strict)"() -> ("Value"=w459:u32)  [unwired: 2 in, 2 out]
            n389 = property on="R offset deg" class="DigNum (strict)"() -> ("Value"=w455:dbl)  [unwired: 2 in, 2 out]
            n390 = To Long Integer(number=w463) -> (32bit integer=w462:i32)
            n391 = To Long Integer(number=w465) -> (32bit integer=w464:i32)
            n392 = To Double Precision Float(number=w459) -> (double precision float=w460:dbl)
            n393 = call "mDrive Send Command.vi"("error in (no error)"=w437, "Extra"="P", "Command"=T2."Print Parameter", "VISA resource name"=w438) -> ("error out"=w467:errorcluster, "read buffer"=w471:string, "VISA resource name out"=w469:refnum<visa-resource-name>)  [unwired: 3 in]
            n394 = call "Time Delay21"("error in (no error)"=w467, "Delay Time (s)"=w443) -> ("error out"=w466:errorcluster)  [unwired: 9 in]
            n395 = Decimal String To Number(string=w471, offset=0) -> (number=w451:i32)  [unwired: 1 in, 1 out]
            n396 = To Long Integer(number=w451) -> (32bit integer=w453:i32)
            n397 = property on="R Step PV" class="DigNum (strict)"("Val(Sgnl)"=w453) -> ()  [unwired: 2 in, 2 out]
            n398 = call "mDrive Send Command.vi"("error in (no error)"=w466, "Extra"="MV", "Command"=T2."Print Parameter", "VISA resource name"=w469) -> ("error out"=w468:errorcluster, "read buffer"=w449:string, "VISA resource name out"=w472:refnum<visa-resource-name>)  [unwired: 3 in]
            n399 = call "Time Delay20"("error in (no error)"=w468, "Delay Time (s)"=w443) -> ("error out"=w448:errorcluster)  [unwired: 9 in]
            n400 = In Range and Coerce(upper limit=w462, x=w453, lower limit=w464) -> (In Range?=w461:bool)  [unwired: 1 out]
            n401 = To Double Precision Float(number=w453) -> (double precision float=w454:dbl)
            n402 = Decimal String To Number(string=w449, offset=0 ("offset (0)")) -> (number=w442:i32)  [unwired: 1 in, 1 out]
            n403 = property on="R in Range" class="Bool (strict)"("Val(Sgnl)"=w461) -> ()  [unwired: 2 in, 2 out]
            n404 = Divide(x=w454, y=w460) -> (x/y=w458:dbl)
            n405 = Number To Boolean Array(number=w442) -> (Boolean array=w441:bool[])
            n406 = property on="R deg/rev" class="DigNum (strict)"() -> ("Value"=w457:dbl)  [unwired: 2 in, 2 out]
            n407 = Index Array(array=w441, index=0) -> (element=w439:bool)
            n408 = property on="R in Motion" class="Bool (strict)"("Val(Sgnl)"=w439) -> ()  [unwired: 2 in, 2 out]
            n409 = Multiply(x=w458, y=w457) -> (x*y=w456:dbl)
            n410 = Add(x=w456, y=w455) -> (x+y=w452:dbl)
            n411 = property on="R Position deg PV" class="DigNum (strict)"("Val(Sgnl)"=w452) -> ()  [unwired: 2 in, 2 out]
          }
          frame #1 {
            n412 = property on="R Scan" class="Bool (strict)"() -> ("Value"=w474:bool)  [unwired: 2 in, 2 out]
            n413 = Or(x=w473, y=w474) -> (x .or. y?=w475:bool)
            n414 = case shown="True" w475 {
              frame #0 {
                n415 = property on="R Go" class="Bool"("DisabledEnum"=T1."Enabled" ("Disabled")) -> ()  [unwired: 2 in, 2 out]
                n416 = property on="R Scan OK" class="Bool"("DisabledEnum"=T1."Enabled" ("Disabled")) -> ()  [unwired: 2 in, 2 out]
              }
              frame #1 {
                n417 = property on="R Go" class="Bool"("DisabledEnum"=T1."Disabled and Grayed Out" ("Disabled")) -> ()  [unwired: 2 in, 2 out]
                n418 = property on="R Scan OK" class="Bool"("DisabledEnum"=T1."Disabled and Grayed Out" ("Disabled")) -> ()  [unwired: 2 in, 2 out]
              }
            }
          }
          frame #2 {
            n419 = case shown="False" w484 {
              tunnel: w485 -> [w491 w495]
              tunnel: [w492 w495] -> w486
              tunnel: [w493 w494] -> w487
              tunnel: w488 -> [w490 w494]
              frame #0 {
                n420 = call "mDrive Send Command.vi"("error in (no error)"=w490, "Command"=T2."Stop", "VISA resource name"=w491) -> ("error out"=w493:errorcluster, "VISA resource name out"=w492:refnum<visa-resource-name>)  [unwired: 4 in, 1 out]
              }
              frame #1 {
              }
            }
          }
          frame #3 {
            n421 = property on="R Backlash corr" class="Bool (strict)"() -> ("Value"=w502:bool)  [unwired: 2 in, 2 out]
            n422 = Implies(1:w501, 2:w502) -> (0:w500:bool)
            n423 = case shown="False" w500 {
              tunnel: w499 -> [w509 w562]
              tunnel: w498 -> [w508 w563]
              tunnel: [w507 w562] -> w497
              tunnel: [w506 w563] -> w496
              frame #0 {
                # "Backlash"
                n424 = flat-sequence {
                  tunnel: [w524] -> w521
                  tunnel: [w526] -> w520
                  tunnel: [w525] -> w519
                  tunnel: w509 -> [w523]
                  tunnel: w508 -> [w522]
                  tunnel: w521 -> [w534]
                  tunnel: [w534] -> w518
                  tunnel: w520 -> [w533]
                  tunnel: w519 -> [w532]
                  tunnel: [w531] -> w517
                  tunnel: [w530] -> w516
                  tunnel: [w529] -> w505
                  tunnel: w518 -> [w544]
                  tunnel: w517 -> [w543]
                  tunnel: w516 -> [w541]
                  tunnel: [w542] -> w515
                  tunnel: [w541] -> w514
                  tunnel: [w540] -> w511
                  tunnel: [w539] -> w510
                  tunnel: w505 -> [w539]
                  tunnel: w515 -> [w555]
                  tunnel: w514 -> [w548]
                  tunnel: [w555] -> w513
                  tunnel: [w554] -> w512
                  tunnel: w511 -> [w554]
                  tunnel: w510 -> [w550]
                  tunnel: [w549] -> w503
                  tunnel: w513 -> [w559]
                  tunnel: w512 -> [w558]
                  tunnel: [w557] -> w507
                  tunnel: [w556] -> w504
                  tunnel: w503 -> [w556]
                  tunnel: [w561] -> w506
                  tunnel: w504 -> [w561]
                  frame #0 {
                    n425 = property on="R Backlash steps/sec" class="DigNum (strict)"() -> ("Value"=w524:i32)  [unwired: 2 in, 2 out]
                    n426 = Number To Decimal String(number=w524) -> (decimal integer string=w527:string)  [unwired: 1 in]
                    n427 = call "mDrive Send Command.vi"("error in (no error)"=w523, "Extra"=w527, "Command"=T2."Max Velocity", "VISA resource name"=w522) -> ("error out"=w525:errorcluster, "VISA resource name out"=w526:refnum<visa-resource-name>)  [unwired: 3 in, 1 out]
                  }
                  frame #1 {
                    n428 = property on="R Backlash" class="DigNum (strict)"() -> ("Value"=w529:i32)  [unwired: 2 in, 2 out]
                    n429 = Number To Decimal String(number=w529) -> (decimal integer string=w535:string)  [unwired: 1 in]
                    n430 = call "mDrive Send Command.vi"("error in (no error)"=w532, "Extra"=w535, "Command"=T2."Move to Relative Position", "VISA resource name"=w533) -> ("error out"=w531:errorcluster, "VISA resource name out"=w530:refnum<visa-resource-name>)  [unwired: 3 in, 1 out]
                  }
                  frame #2 {
                    n431 = To Double Precision Float(number=w539) -> (double precision float=w537:dbl)
                    n432 = To Double Precision Float(number=w544) -> (double precision float=w546:dbl)
                    n433 = Absolute Value(x=w537) -> (abs(x)=w538:dbl)
                    n434 = Divide(x=w538, y=w546) -> (x/y=w547:dbl)
                    n435 = Add(x=w547, y=0.3) -> (x+y=w540:dbl)
                    n436 = call "Time Delay22"("error in (no error)"=w543, "Delay Time (s)"=w540) -> ("error out"=w542:errorcluster)  [unwired: 9 in]
                  }
                  frame #3 {
                    n437 = Negate(x=w550) -> (-x=w551:i32)
                    n438 = Number To Decimal String(number=w551) -> (decimal integer string=w552:string)  [unwired: 1 in]
                    n439 = call "mDrive Send Command.vi"("Extra"=w552, "Command"=T2."Move to Relative Position", "VISA resource name"=w548) -> ("VISA resource name out"=w549:refnum<visa-resource-name>)  [unwired: 4 in, 2 out]
                  }
                  frame #4 {
                    n440 = call "Time Delay23"("error in (no error)"=w559, "Delay Time (s)"=w558) -> ("error out"=w557:errorcluster)  [unwired: 9 in]
                  }
                  frame #5 {
                    n441 = property on="R Backlash corr" class="Bool (strict)"("Val(Sgnl)"=FALSE ("Value (Signaling)")) -> ()  [unwired: 2 in, 2 out]
                  }
                }
              }
              frame #1 {
              }
            }
          }
          frame #4 {
            n442 = property on="R Step PV" class="DigNum (strict)"() -> ("Value"=w572:i32)  [unwired: 2 in, 2 out]
            n443 = property on="R Step PV" class="DigNum (strict)"() -> ("Value"=w574:i32)  [unwired: 2 in, 2 out]
            n444 = property on="R steps/rev" class="DigNum (strict)"() -> ("Value"=w576:u32)  [unwired: 2 in, 2 out]
            n445 = To Double Precision Float(number=w576) -> (double precision float=w570:dbl)
            n446 = property on="R Step SP" class="DigNum (strict)"() -> ("Maximum"=w581:dbl)  [unwired: 2 in, 2 out]
            n447 = property on="R Step SP" class="DigNum (strict)"() -> ("Minimum"=w582:dbl)  [unwired: 2 in, 2 out]
            n448 = To Double Precision Float(number=w572) -> (double precision float=w571:dbl)
            n449 = To Double Precision Float(number=w574) -> (double precision float=w573:dbl)
            n450 = Subtract(x=w582, y=w571) -> (x-y=w583:dbl)
            n451 = Subtract(x=w581, y=w573) -> (x-y=w580:dbl)
            n452 = property on="R Velocity SP step/sec" class="DigNum (strict)"() -> ("Value"=w569:i32)  [unwired: 2 in, 2 out]
            n453 = property on="R Scan Length SP steps" class="DigNum (strict)"() -> ("Value"=w578:i32)  [unwired: 2 in, 2 out]
            n454 = To Double Precision Float(number=w578) -> (double precision float=w577:dbl)
            n455 = To Double Precision Float(number=w569) -> (double precision float=w568:dbl)
            n456 = property on="R Scan Length SP steps" class="DigNum (strict)"("Minimum"=w583) -> ()  [unwired: 2 in, 2 out]
            n457 = property on="R Scan Length SP steps" class="DigNum (strict)"("Maximum"=w580) -> ()  [unwired: 2 in, 2 out]
            n458 = Divide(x=w577, y=w570) -> (x/y=w579:dbl)
            n459 = Divide(x=w568, y=w570) -> (x/y=w567:dbl)
            n460 = property on="R deg/rev" class="DigNum (strict)"() -> ("Value"=w575:dbl)  [unwired: 2 in, 2 out]
            n461 = Multiply(x=w579, y=w575) -> (x*y=w566:dbl)
            n462 = Multiply(x=w575, y=w567) -> (x*y=w565:dbl)
            n463 = property on="R Scan length MV deg" class="DigNum (strict)"("Value"=w566) -> ()  [unwired: 2 in, 2 out]
            n464 = property on="R Scan Velocity SP deg/sec" class="DigNum (strict)"("Val(Sgnl)"=w565) -> ()  [unwired: 2 in, 2 out]
          }
        }
      }
      event #1 {
        n465 = event-data() -> ()  [unwired: 1 in, 5 out]
        n466 = property on="Z steps/rev" class="DigNum (strict)"() -> ("Value"=w1040:u32)  [unwired: 2 in, 2 out]
        n467 = property on="X steps/rev" class="DigNum (strict)"() -> ("Value"=w1049:u32)  [unwired: 2 in, 2 out]
        n468 = property on="Y steps/rev" class="DigNum (strict)"() -> ("Value"=w1058:u32)  [unwired: 2 in, 2 out]
        n469 = property on="R steps/rev" class="DigNum (strict)"() -> ("Value"=w1031:u32)  [unwired: 2 in, 2 out]
        n470 = property on="R offset deg" class="DigNum (strict)"() -> ("Value"=w1029:dbl)  [unwired: 2 in, 2 out]
        n471 = property on="Z offset mm" class="DigNum (strict)"() -> ("Value"=w1038:dbl)  [unwired: 2 in, 2 out]
        n472 = property on="X offset mm" class="DigNum (strict)"() -> ("Value"=w1047:dbl)  [unwired: 2 in, 2 out]
        n473 = property on="Y offset mm" class="DigNum (strict)"() -> ("Value"=w1056:dbl)  [unwired: 2 in, 2 out]
        n474 = property on="Reset Z Position mm" class="DigNum (strict)"() -> ("Value"=w1046:dbl)  [unwired: 2 in, 2 out]
        n475 = property on="Reset X Position mm" class="DigNum (strict)"() -> ("Value"=w1055:dbl)  [unwired: 2 in, 2 out]
        n476 = property on="Reset Y Position mm" class="DigNum (strict)"() -> ("Value"=w1064:dbl)  [unwired: 2 in, 2 out]
        n477 = property on="Reset R Position deg" class="DigNum (strict)"() -> ("Value"=w1037:dbl)  [unwired: 2 in, 2 out]
        n478 = Subtract(x=w1046, y=w1038) -> (x-y=w1045:dbl)
        n479 = Subtract(x=w1037, y=w1029) -> (x-y=w1036:dbl)
        n480 = Subtract(x=w1055, y=w1047) -> (x-y=w1054:dbl)
        n481 = Subtract(x=w1064, y=w1056) -> (x-y=w1063:dbl)
        n482 = property on="Z mm/rev" class="DigNum (strict)"() -> ("Value"=w1039:dbl)  [unwired: 2 in, 2 out]
        n483 = property on="X mm/rev" class="DigNum (strict)"() -> ("Value"=w1048:dbl)  [unwired: 2 in, 2 out]
        n484 = property on="Y mm/rev" class="DigNum (strict)"() -> ("Value"=w1057:dbl)  [unwired: 2 in, 2 out]
        n485 = property on="R deg/rev" class="DigNum (strict)"() -> ("Value"=w1030:dbl)  [unwired: 2 in, 2 out]
        n486 = Divide(x=w1045, y=w1039) -> (x/y=w1044:dbl)
        n487 = Divide(x=w1036, y=w1030) -> (x/y=w1035:dbl)
        n488 = Divide(x=w1054, y=w1048) -> (x/y=w1053:dbl)
        n489 = Divide(x=w1063, y=w1057) -> (x/y=w1062:dbl)
        n490 = To Double Precision Float(number=w1040) -> (double precision float=w1043:dbl)
        n491 = To Double Precision Float(number=w1031) -> (double precision float=w1034:dbl)
        n492 = To Double Precision Float(number=w1049) -> (double precision float=w1052:dbl)
        n493 = To Double Precision Float(number=w1058) -> (double precision float=w1061:dbl)
        n494 = Multiply(x=w1044, y=w1043) -> (x*y=w1042:dbl)
        n495 = Multiply(x=w1035, y=w1034) -> (x*y=w1033:dbl)
        n496 = Multiply(x=w1053, y=w1052) -> (x*y=w1051:dbl)
        n497 = Multiply(x=w1062, y=w1061) -> (x*y=w1060:dbl)
        n498 = To Long Integer(number=w1042) -> (32bit integer=w1041:i32)
        n499 = To Long Integer(number=w1033) -> (32bit integer=w1032:i32)
        n500 = To Long Integer(number=w1051) -> (32bit integer=w1050:i32)
        n501 = To Long Integer(number=w1060) -> (32bit integer=w1059:i32)
        n502 = property on="Reset Z Motor Steps" class="DigNum (strict)"("Val(Sgnl)"=w1041) -> ()  [unwired: 2 in, 2 out]
        n503 = property on="Reset R Motor Steps" class="DigNum (strict)"("Val(Sgnl)"=w1032) -> ()  [unwired: 2 in, 2 out]
        n504 = property on="Reset X Motor Steps" class="DigNum (strict)"("Val(Sgnl)"=w1050) -> ()  [unwired: 2 in, 2 out]
        n505 = property on="Reset Y Motor Steps" class="DigNum (strict)"("Val(Sgnl)"=w1059) -> ()  [unwired: 2 in, 2 out]
      }
      event #2 {
        n506 = event-data() -> ()  [unwired: 1 in, 5 out]
        n507 = property on="Y Step SP" class="DigNum (strict)"() -> ("Value"=w1096:i32)  [unwired: 2 in, 2 out]
        n508 = property on="X Step SP" class="DigNum (strict)"() -> ("Value"=w1087:i32)  [unwired: 2 in, 2 out]
        n509 = property on="Z Step SP" class="DigNum (strict)"() -> ("Value"=w1078:i32)  [unwired: 2 in, 2 out]
        n510 = property on="Y steps/rev" class="DigNum (strict)"() -> ("Value"=w1094:u32)  [unwired: 2 in, 2 out]
        n511 = property on="X steps/rev" class="DigNum (strict)"() -> ("Value"=w1085:u32)  [unwired: 2 in, 2 out]
        n512 = property on="Z steps/rev" class="DigNum (strict)"() -> ("Value"=w1076:u32)  [unwired: 2 in, 2 out]
        n513 = property on="R Step SP" class="DigNum (strict)"() -> ("Value"=w1069:i32)  [unwired: 2 in, 2 out]
        n514 = property on="R steps/rev" class="DigNum (strict)"() -> ("Value"=w1067:u32)  [unwired: 2 in, 2 out]
        n515 = property on="R offset deg" class="DigNum (strict)"() -> ("Value"=w1065:dbl)  [unwired: 2 in, 2 out]
        n516 = property on="Y offset mm" class="DigNum (strict)"() -> ("Value"=w1092:dbl)  [unwired: 2 in, 2 out]
        n517 = property on="X offset mm" class="DigNum (strict)"() -> ("Value"=w1083:dbl)  [unwired: 2 in, 2 out]
        n518 = property on="Z offset mm" class="DigNum (strict)"() -> ("Value"=w1074:dbl)  [unwired: 2 in, 2 out]
        n519 = To Double Precision Float(number=w1096) -> (double precision float=w1097:dbl)
        n520 = To Double Precision Float(number=w1094) -> (double precision float=w1100:dbl)
        n521 = To Double Precision Float(number=w1087) -> (double precision float=w1088:dbl)
        n522 = To Double Precision Float(number=w1085) -> (double precision float=w1091:dbl)
        n523 = To Double Precision Float(number=w1078) -> (double precision float=w1079:dbl)
        n524 = To Double Precision Float(number=w1076) -> (double precision float=w1082:dbl)
        n525 = To Double Precision Float(number=w1069) -> (double precision float=w1070:dbl)
        n526 = To Double Precision Float(number=w1067) -> (double precision float=w1073:dbl)
        n527 = Divide(x=w1097, y=w1100) -> (x/y=w1099:dbl)
        n528 = Divide(x=w1088, y=w1091) -> (x/y=w1090:dbl)
        n529 = Divide(x=w1079, y=w1082) -> (x/y=w1081:dbl)
        n530 = Divide(x=w1070, y=w1073) -> (x/y=w1072:dbl)
        n531 = property on="Y mm/rev" class="DigNum (strict)"() -> ("Value"=w1093:dbl)  [unwired: 2 in, 2 out]
        n532 = property on="X mm/rev" class="DigNum (strict)"() -> ("Value"=w1084:dbl)  [unwired: 2 in, 2 out]
        n533 = property on="Z mm/rev" class="DigNum (strict)"() -> ("Value"=w1075:dbl)  [unwired: 2 in, 2 out]
        n534 = property on="R deg/rev" class="DigNum (strict)"() -> ("Value"=w1066:dbl)  [unwired: 2 in, 2 out]
        n535 = Multiply(x=w1099, y=w1093) -> (x*y=w1098:dbl)
        n536 = Multiply(x=w1090, y=w1084) -> (x*y=w1089:dbl)
        n537 = Multiply(x=w1081, y=w1075) -> (x*y=w1080:dbl)
        n538 = Multiply(x=w1072, y=w1066) -> (x*y=w1071:dbl)
        n539 = Add(x=w1098, y=w1092) -> (x+y=w1095:dbl)
        n540 = Add(x=w1089, y=w1083) -> (x+y=w1086:dbl)
        n541 = Add(x=w1080, y=w1074) -> (x+y=w1077:dbl)
        n542 = Add(x=w1071, y=w1065) -> (x+y=w1068:dbl)
        n543 = property on="Y Position MV mm" class="DigNum (strict)"("Val(Sgnl)"=w1095) -> ()  [unwired: 2 in, 2 out]
        n544 = property on="X Position MV mm" class="DigNum (strict)"("Val(Sgnl)"=w1086) -> ()  [unwired: 2 in, 2 out]
        n545 = property on="Z Position MV mm" class="DigNum (strict)"("Val(Sgnl)"=w1077) -> ()  [unwired: 2 in, 2 out]
        n546 = property on="R Position MV deg" class="DigNum (strict)"("Val(Sgnl)"=w1068) -> ()  [unwired: 2 in, 2 out]
      }
      event #3 {
        n547 = event-data() -> ()  [unwired: 1 in, 5 out]
        n548 = property on="Y steps/rev" class="DigNum (strict)"() -> ("Value"=w1123:u32)  [unwired: 2 in, 2 out]
        n549 = property on="X steps/rev" class="DigNum (strict)"() -> ("Value"=w1116:u32)  [unwired: 2 in, 2 out]
        n550 = property on="Z steps/rev" class="DigNum (strict)"() -> ("Value"=w1109:u32)  [unwired: 2 in, 2 out]
        n551 = property on="R steps/rev" class="DigNum (strict)"() -> ("Value"=w1102:u32)  [unwired: 2 in, 2 out]
        n552 = property on="Y Velocity SP step/sec" class="DigNum (strict)"() -> ("Value"=w1125:i32)  [unwired: 2 in, 2 out]
        n553 = property on="X Velocity SP step/sec" class="DigNum (strict)"() -> ("Value"=w1118:i32)  [unwired: 2 in, 2 out]
        n554 = property on="Z Velocity SP step/sec" class="DigNum (strict)"() -> ("Value"=w1111:i32)  [unwired: 2 in, 2 out]
        n555 = property on="R Velocity SP step/sec" class="DigNum (strict)"() -> ("Value"=w1104:i32)  [unwired: 2 in, 2 out]
        n556 = To Double Precision Float(number=w1125) -> (double precision float=w1126:dbl)
        n557 = To Double Precision Float(number=w1123) -> (double precision float=w1128:dbl)
        n558 = To Double Precision Float(number=w1118) -> (double precision float=w1119:dbl)
        n559 = To Double Precision Float(number=w1116) -> (double precision float=w1121:dbl)
        n560 = To Double Precision Float(number=w1111) -> (double precision float=w1112:dbl)
        n561 = To Double Precision Float(number=w1109) -> (double precision float=w1114:dbl)
        n562 = To Double Precision Float(number=w1104) -> (double precision float=w1105:dbl)
        n563 = To Double Precision Float(number=w1102) -> (double precision float=w1107:dbl)
        n564 = Divide(x=w1126, y=w1128) -> (x/y=w1127:dbl)
        n565 = Divide(x=w1119, y=w1121) -> (x/y=w1120:dbl)
        n566 = Divide(x=w1112, y=w1114) -> (x/y=w1113:dbl)
        n567 = Divide(x=w1105, y=w1107) -> (x/y=w1106:dbl)
        n568 = property on="Y mm/rev" class="DigNum (strict)"() -> ("Value"=w1122:dbl)  [unwired: 2 in, 2 out]
        n569 = property on="X mm/rev" class="DigNum (strict)"() -> ("Value"=w1115:dbl)  [unwired: 2 in, 2 out]
        n570 = property on="Z mm/rev" class="DigNum (strict)"() -> ("Value"=w1108:dbl)  [unwired: 2 in, 2 out]
        n571 = property on="R deg/rev" class="DigNum (strict)"() -> ("Value"=w1101:dbl)  [unwired: 2 in, 2 out]
        n572 = Multiply(x=w1127, y=w1122) -> (x*y=w1124:dbl)
        n573 = Multiply(x=w1120, y=w1115) -> (x*y=w1117:dbl)
        n574 = Multiply(x=w1113, y=w1108) -> (x*y=w1110:dbl)
        n575 = Multiply(x=w1106, y=w1101) -> (x*y=w1103:dbl)
        n576 = property on="Y Velocity MV mm/sec" class="DigNum (strict)"("Val(Sgnl)"=w1124) -> ()  [unwired: 2 in, 2 out]
        n577 = property on="X Velocity MV mm/sec" class="DigNum (strict)"("Val(Sgnl)"=w1117) -> ()  [unwired: 2 in, 2 out]
        n578 = property on="Z Velocity MV mm/sec" class="DigNum (strict)"("Val(Sgnl)"=w1110) -> ()  [unwired: 2 in, 2 out]
        n579 = property on="R Velocity MVdeg/sec" class="DigNum (strict)"("Val(Sgnl)"=w1103) -> ()  [unwired: 2 in, 2 out]
      }
      event #4 {
        n580 = event-data() -> ()  [unwired: 1 in, 7 out]
        n581 = property on="Y steps/rev" class="DigNum (strict)"() -> ("Value"=w1145:u32)  [unwired: 2 in, 2 out]
        n582 = property on="Y offset mm" class="DigNum (strict)"() -> ("Value"=w1143:dbl)  [unwired: 2 in, 2 out]
        n583 = property on="Y Position SP mm" class="DigNum (strict)"() -> ("Value"=w1142:dbl)  [unwired: 2 in, 2 out]
        n584 = Subtract(x=w1142, y=w1143) -> (x-y=w1146:dbl)
        n585 = property on="Y mm/rev" class="DigNum (strict)"() -> ("Value"=w1129:dbl)  [unwired: 2 in, 2 out]
        n586 = Divide(x=w1146, y=w1129) -> (x/y=w1147:dbl)
        n587 = To Double Precision Float(number=w1145) -> (double precision float=w1130:dbl)
        n588 = Multiply(x=w1147, y=w1130) -> (x*y=w1141:dbl)
        n589 = property on="Y Step SP" class="DigNum (strict)"() -> ("Maximum"=w1139:dbl)  [unwired: 2 in, 2 out]
        n590 = property on="Y Step SP" class="DigNum (strict)"() -> ("Minimum"=w1138:dbl)  [unwired: 2 in, 2 out]
        n591 = In Range and Coerce(upper limit=w1139, x=w1141, lower limit=w1138) -> (coerced(x)=w1140:dbl)  [unwired: 1 out]
        n592 = To Long Integer(number=w1140) -> (32bit integer=w1144:i32)
        n593 = property on="Y Step SP" class="DigNum (strict)"("Val(Sgnl)"=w1144) -> ()  [unwired: 2 in, 2 out]
        n594 = property on="Y Velocity SP step/sec" class="DigNum (strict)"() -> ("Maximum"=w1132:dbl)  [unwired: 2 in, 2 out]
        n595 = property on="Y Velocity SP step/sec" class="DigNum (strict)"() -> ("Minimum"=w1131:dbl)  [unwired: 2 in, 2 out]
        n596 = property on="Y Velocity SP mm/sec" class="DigNum (strict)"() -> ("Value"=w1136:dbl)  [unwired: 2 in, 2 out]
        n597 = Divide(x=w1136, y=w1129) -> (x/y=w1137:dbl)
        n598 = Multiply(x=w1137, y=w1130) -> (x*y=w1134:dbl)
        n599 = In Range and Coerce(upper limit=w1132, x=w1134, lower limit=w1131) -> (coerced(x)=w1133:dbl)  [unwired: 1 out]
        n600 = To Long Integer(number=w1133) -> (32bit integer=w1135:i32)
        n601 = property on="Y Velocity SP step/sec" class="DigNum (strict)"("Val(Sgnl)"=w1135) -> ()  [unwired: 2 in, 2 out]
      }
      event #5 {
        n602 = event-data() -> ()  [unwired: 1 in, 7 out]
        n603 = property on="X steps/rev" class="DigNum (strict)"() -> ("Value"=w1164:u32)  [unwired: 2 in, 2 out]
        n604 = To Double Precision Float(number=w1164) -> (double precision float=w1149:dbl)
        n605 = property on="X offset mm" class="DigNum (strict)"() -> ("Value"=w1162:dbl)  [unwired: 2 in, 2 out]
        n606 = property on="X Position SP mm" class="DigNum (strict)"() -> ("Value"=w1161:dbl)  [unwired: 2 in, 2 out]
        n607 = Subtract(x=w1161, y=w1162) -> (x-y=w1165:dbl)
        n608 = property on="X mm/rev" class="DigNum (strict)"() -> ("Value"=w1148:dbl)  [unwired: 2 in, 2 out]
        n609 = Divide(x=w1165, y=w1148) -> (x/y=w1166:dbl)
        n610 = Multiply(x=w1166, y=w1149) -> (x*y=w1160:dbl)
        n611 = property on="X Step SP" class="DigNum (strict)"() -> ("Maximum"=w1158:dbl)  [unwired: 2 in, 2 out]
        n612 = property on="X Step SP" class="DigNum (strict)"() -> ("Minimum"=w1157:dbl)  [unwired: 2 in, 2 out]
        n613 = In Range and Coerce(upper limit=w1158, x=w1160, lower limit=w1157) -> (coerced(x)=w1159:dbl)  [unwired: 1 out]
        n614 = To Long Integer(number=w1159) -> (32bit integer=w1163:i32)
        n615 = property on="X Step SP" class="DigNum (strict)"("Val(Sgnl)"=w1163) -> ()  [unwired: 2 in, 2 out]
        n616 = property on="X Velocity SP step/sec" class="DigNum (strict)"() -> ("Maximum"=w1151:dbl)  [unwired: 2 in, 2 out]
        n617 = property on="X Velocity SP step/sec" class="DigNum (strict)"() -> ("Minimum"=w1150:dbl)  [unwired: 2 in, 2 out]
        n618 = property on="X Velocity SP mm/sec" class="DigNum (strict)"() -> ("Value"=w1155:dbl)  [unwired: 2 in, 2 out]
        n619 = Divide(x=w1155, y=w1148) -> (x/y=w1156:dbl)
        n620 = Multiply(x=w1156, y=w1149) -> (x*y=w1153:dbl)
        n621 = In Range and Coerce(upper limit=w1151, x=w1153, lower limit=w1150) -> (coerced(x)=w1152:dbl)  [unwired: 1 out]
        n622 = To Long Integer(number=w1152) -> (32bit integer=w1154:i32)
        n623 = property on="X Velocity SP step/sec" class="DigNum (strict)"("Val(Sgnl)"=w1154) -> ()  [unwired: 2 in, 2 out]
      }
      event #6 {
        n624 = event-data() -> ()  [unwired: 1 in, 7 out]
        n625 = property on="Z steps/rev" class="DigNum (strict)"() -> ("Value"=w1181:u32)  [unwired: 2 in, 2 out]
        n626 = To Double Precision Float(number=w1181) -> (double precision float=w1185:dbl)
        n627 = property on="Z offset mm" class="DigNum (strict)"() -> ("Value"=w1179:dbl)  [unwired: 2 in, 2 out]
        n628 = property on="Z Position SP mm" class="DigNum (strict)"() -> ("Value"=w1178:dbl)  [unwired: 2 in, 2 out]
        n629 = Subtract(x=w1178, y=w1179) -> (x-y=w1182:dbl)
        n630 = property on="Z mm/rev" class="DigNum (strict)"() -> ("Value"=w1184:dbl)  [unwired: 2 in, 2 out]
        n631 = Divide(x=w1182, y=w1184) -> (x/y=w1183:dbl)
        n632 = Multiply(x=w1183, y=w1185) -> (x*y=w1177:dbl)
        n633 = property on="Z Step SP" class="DigNum (strict)"() -> ("Maximum"=w1175:dbl)  [unwired: 2 in, 2 out]
        n634 = property on="Z Step SP" class="DigNum (strict)"() -> ("Minimum"=w1174:dbl)  [unwired: 2 in, 2 out]
        n635 = In Range and Coerce(upper limit=w1175, x=w1177, lower limit=w1174) -> (coerced(x)=w1176:dbl)  [unwired: 1 out]
        n636 = To Long Integer(number=w1176) -> (32bit integer=w1180:i32)
        n637 = property on="Z Step SP" class="DigNum (strict)"("Val(Sgnl)"=w1180) -> ()  [unwired: 2 in, 2 out]
        n638 = property on="Z Velocity SP step/sec" class="DigNum (strict)"() -> ("Maximum"=w1168:dbl)  [unwired: 2 in, 2 out]
        n639 = property on="Z Velocity SP step/sec" class="DigNum (strict)"() -> ("Minimum"=w1167:dbl)  [unwired: 2 in, 2 out]
        n640 = property on="Z Velocity SP mm/sec" class="DigNum (strict)"() -> ("Value"=w1172:dbl)  [unwired: 2 in, 2 out]
        n641 = Divide(x=w1172, y=w1184) -> (x/y=w1173:dbl)
        n642 = Multiply(x=w1173, y=w1185) -> (x*y=w1170:dbl)
        n643 = In Range and Coerce(upper limit=w1168, x=w1170, lower limit=w1167) -> (coerced(x)=w1169:dbl)  [unwired: 1 out]
        n644 = To Long Integer(number=w1169) -> (32bit integer=w1171:i32)
        n645 = property on="Z Velocity SP step/sec" class="DigNum (strict)"("Val(Sgnl)"=w1171) -> ()  [unwired: 2 in, 2 out]
      }
      event #7 {
        n646 = event-data() -> ()  [unwired: 1 in, 7 out]
        n647 = property on="R steps/rev" class="DigNum (strict)"() -> ("Value"=w1202:u32)  [unwired: 2 in, 2 out]
        n648 = property on="R offset deg" class="DigNum (strict)"() -> ("Value"=w1200:dbl)  [unwired: 2 in, 2 out]
        n649 = property on="R Position SP deg" class="DigNum (strict)"() -> ("Value"=w1199:dbl)  [unwired: 2 in, 2 out]
        n650 = Subtract(x=w1199, y=w1200) -> (x-y=w1203:dbl)
        n651 = property on="R deg/rev" class="DigNum (strict)"() -> ("Value"=w1186:dbl)  [unwired: 2 in, 2 out]
        n652 = Divide(x=w1203, y=w1186) -> (x/y=w1204:dbl)
        n653 = To Double Precision Float(number=w1202) -> (double precision float=w1187:dbl)
        n654 = Multiply(x=w1204, y=w1187) -> (x*y=w1198:dbl)
        n655 = property on="R Step SP" class="DigNum (strict)"() -> ("Maximum"=w1196:dbl)  [unwired: 2 in, 2 out]
        n656 = property on="R Step SP" class="DigNum (strict)"() -> ("Minimum"=w1195:dbl)  [unwired: 2 in, 2 out]
        n657 = In Range and Coerce(upper limit=w1196, x=w1198, lower limit=w1195) -> (coerced(x)=w1197:dbl)  [unwired: 1 out]
        n658 = To Long Integer(number=w1197) -> (32bit integer=w1201:i32)
        n659 = property on="R Step SP" class="DigNum (strict)"("Val(Sgnl)"=w1201) -> ()  [unwired: 2 in, 2 out]
        n660 = property on="R Velocity SP step/sec" class="DigNum (strict)"() -> ("Maximum"=w1189:dbl)  [unwired: 2 in, 2 out]
        n661 = property on="R Velocity SP step/sec" class="DigNum (strict)"() -> ("Minimum"=w1188:dbl)  [unwired: 2 in, 2 out]
        n662 = property on="R Velocity SP deg/sec" class="DigNum (strict)"() -> ("Value"=w1193:dbl)  [unwired: 2 in, 2 out]
        n663 = Divide(x=w1193, y=w1186) -> (x/y=w1194:dbl)
        n664 = Multiply(x=w1194, y=w1187) -> (x*y=w1191:dbl)
        n665 = In Range and Coerce(upper limit=w1189, x=w1191, lower limit=w1188) -> (coerced(x)=w1190:dbl)  [unwired: 1 out]
        n666 = To Long Integer(number=w1190) -> (32bit integer=w1192:i32)
        n667 = property on="R Velocity SP step/sec" class="DigNum (strict)"("Val(Sgnl)"=w1192) -> ()  [unwired: 2 in, 2 out]
      }
      event #8 {
        n668 = event-data() -> ()  [unwired: 1 in, 7 out]
        n669 = property on="Y steps/rev" class="DigNum (strict)"() -> ("Value"=w1220:u32)  [unwired: 2 in, 2 out]
        n670 = To Double Precision Float(number=w1220) -> (double precision float=w1206:dbl)
        n671 = property on="Y Scan Length SP mm" class="DigNum (strict)"() -> ("Value"=w1218:dbl)  [unwired: 2 in, 2 out]
        n672 = property on="Y mm/rev" class="DigNum (strict)"() -> ("Value"=w1205:dbl)  [unwired: 2 in, 2 out]
        n673 = Divide(x=w1218, y=w1205) -> (x/y=w1221:dbl)
        n674 = Multiply(x=w1221, y=w1206) -> (x*y=w1217:dbl)
        n675 = property on="Y Step SP" class="DigNum (strict)"() -> ("Maximum"=w1214:dbl)  [unwired: 2 in, 2 out]
        n676 = property on="Y Step SP" class="DigNum (strict)"() -> ("Minimum"=w1215:dbl)  [unwired: 2 in, 2 out]
        n677 = In Range and Coerce(upper limit=w1214, x=w1217, lower limit=w1215) -> (coerced(x)=w1216:dbl)  [unwired: 1 out]
        n678 = To Long Integer(number=w1216) -> (32bit integer=w1219:i32)
        n679 = property on="Y Scan Length SP steps" class="DigNum (strict)"("Val(Sgnl)"=w1219) -> ()  [unwired: 2 in, 2 out]
        n680 = property on="Y Scan Velocity SP mm/sec" class="DigNum (strict)"() -> ("Value"=w1212:dbl)  [unwired: 2 in, 2 out]
        n681 = property on="Y Scan Velocity SP steps/sec" class="DigNum (strict)"() -> ("Maximum"=w1208:dbl)  [unwired: 2 in, 2 out]
        n682 = property on="Y Scan Velocity SP steps/sec" class="DigNum (strict)"() -> ("Minimum"=w1207:dbl)  [unwired: 2 in, 2 out]
        n683 = Divide(x=w1212, y=w1205) -> (x/y=w1213:dbl)
        n684 = Multiply(x=w1213, y=w1206) -> (x*y=w1210:dbl)
        n685 = In Range and Coerce(upper limit=w1208, x=w1210, lower limit=w1207) -> (coerced(x)=w1209:dbl)  [unwired: 1 out]
        n686 = To Long Integer(number=w1209) -> (32bit integer=w1211:i32)
        n687 = property on="Y Scan Velocity SP steps/sec" class="DigNum (strict)"("Val(Sgnl)"=w1211) -> ()  [unwired: 2 in, 2 out]
      }
      event #9 {
        n688 = event-data() -> ()  [unwired: 1 in, 7 out]
        n689 = property on="X steps/rev" class="DigNum (strict)"() -> ("Value"=w1237:u32)  [unwired: 2 in, 2 out]
        n690 = To Double Precision Float(number=w1237) -> (double precision float=w1223:dbl)
        n691 = property on="X Scan Length SP mm" class="DigNum (strict)"() -> ("Value"=w1235:dbl)  [unwired: 2 in, 2 out]
        n692 = property on="X mm/rev" class="DigNum (strict)"() -> ("Value"=w1222:dbl)  [unwired: 2 in, 2 out]
        n693 = Divide(x=w1235, y=w1222) -> (x/y=w1238:dbl)
        n694 = Multiply(x=w1238, y=w1223) -> (x*y=w1234:dbl)
        n695 = property on="X Step SP" class="DigNum (strict)"() -> ("Maximum"=w1231:dbl)  [unwired: 2 in, 2 out]
        n696 = property on="X Step SP" class="DigNum (strict)"() -> ("Minimum"=w1232:dbl)  [unwired: 2 in, 2 out]
        n697 = In Range and Coerce(upper limit=w1231, x=w1234, lower limit=w1232) -> (coerced(x)=w1233:dbl)  [unwired: 1 out]
        n698 = To Long Integer(number=w1233) -> (32bit integer=w1236:i32)
        n699 = property on="X Scan Length SP steps" class="DigNum (strict)"("Val(Sgnl)"=w1236) -> ()  [unwired: 2 in, 2 out]
        n700 = property on="X Scan Velocity SP mm/sec" class="DigNum (strict)"() -> ("Value"=w1229:dbl)  [unwired: 2 in, 2 out]
        n701 = property on="X Scan Velocity SP steps/sec" class="DigNum (strict)"() -> ("Maximum"=w1225:dbl)  [unwired: 2 in, 2 out]
        n702 = property on="X Scan Velocity SP steps/sec" class="DigNum (strict)"() -> ("Minimum"=w1224:dbl)  [unwired: 2 in, 2 out]
        n703 = Divide(x=w1229, y=w1222) -> (x/y=w1230:dbl)
        n704 = Multiply(x=w1230, y=w1223) -> (x*y=w1227:dbl)
        n705 = In Range and Coerce(upper limit=w1225, x=w1227, lower limit=w1224) -> (coerced(x)=w1226:dbl)  [unwired: 1 out]
        n706 = To Long Integer(number=w1226) -> (32bit integer=w1228:i32)
        n707 = property on="X Scan Velocity SP steps/sec" class="DigNum (strict)"("Val(Sgnl)"=w1228) -> ()  [unwired: 2 in, 2 out]
      }
      event #10 {
        n708 = event-data() -> ()  [unwired: 1 in, 7 out]
        n709 = property on="Z steps/rev" class="DigNum (strict)"() -> ("Value"=w1254:u32)  [unwired: 2 in, 2 out]
        n710 = To Double Precision Float(number=w1254) -> (double precision float=w1240:dbl)
        n711 = property on="Z Scan Length SP mm" class="DigNum (strict)"() -> ("Value"=w1252:dbl)  [unwired: 2 in, 2 out]
        n712 = property on="Z mm/rev" class="DigNum (strict)"() -> ("Value"=w1239:dbl)  [unwired: 2 in, 2 out]
        n713 = Divide(x=w1252, y=w1239) -> (x/y=w1255:dbl)
        n714 = Multiply(x=w1255, y=w1240) -> (x*y=w1251:dbl)
        n715 = property on="Z Step SP" class="DigNum (strict)"() -> ("Maximum"=w1248:dbl)  [unwired: 2 in, 2 out]
        n716 = property on="Z Step SP" class="DigNum (strict)"() -> ("Minimum"=w1249:dbl)  [unwired: 2 in, 2 out]
        n717 = In Range and Coerce(upper limit=w1248, x=w1251, lower limit=w1249) -> (coerced(x)=w1250:dbl)  [unwired: 1 out]
        n718 = To Long Integer(number=w1250) -> (32bit integer=w1253:i32)
        n719 = property on="Z Scan Length SP steps" class="DigNum (strict)"("Val(Sgnl)"=w1253) -> ()  [unwired: 2 in, 2 out]
        n720 = property on="Z Scan Velocity SP mm/sec" class="DigNum (strict)"() -> ("Value"=w1246:dbl)  [unwired: 2 in, 2 out]
        n721 = property on="Z Scan Velocity SP steps/sec" class="DigNum (strict)"() -> ("Maximum"=w1242:dbl)  [unwired: 2 in, 2 out]
        n722 = property on="Z Scan Velocity SP steps/sec" class="DigNum (strict)"() -> ("Minimum"=w1241:dbl)  [unwired: 2 in, 2 out]
        n723 = Divide(x=w1246, y=w1239) -> (x/y=w1247:dbl)
        n724 = Multiply(x=w1247, y=w1240) -> (x*y=w1244:dbl)
        n725 = In Range and Coerce(upper limit=w1242, x=w1244, lower limit=w1241) -> (coerced(x)=w1243:dbl)  [unwired: 1 out]
        n726 = To Long Integer(number=w1243) -> (32bit integer=w1245:i32)
        n727 = property on="Z Scan Velocity SP steps/sec" class="DigNum (strict)"("Val(Sgnl)"=w1245) -> ()  [unwired: 2 in, 2 out]
      }
      event #11 {
        n728 = event-data() -> ()  [unwired: 1 in, 7 out]
        n729 = property on="R steps/rev" class="DigNum (strict)"() -> ("Value"=w1271:u32)  [unwired: 2 in, 2 out]
        n730 = To Double Precision Float(number=w1271) -> (double precision float=w1257:dbl)
        n731 = property on="R Scan Length SP deg" class="DigNum (strict)"() -> ("Value"=w1269:dbl)  [unwired: 2 in, 2 out]
        n732 = property on="R deg/rev" class="DigNum (strict)"() -> ("Value"=w1256:dbl)  [unwired: 2 in, 2 out]
        n733 = Divide(x=w1269, y=w1256) -> (x/y=w1272:dbl)
        n734 = Multiply(x=w1272, y=w1257) -> (x*y=w1268:dbl)
        n735 = property on="R Step SP" class="DigNum (strict)"() -> ("Maximum"=w1265:dbl)  [unwired: 2 in, 2 out]
        n736 = property on="R Step SP" class="DigNum (strict)"() -> ("Minimum"=w1266:dbl)  [unwired: 2 in, 2 out]
        n737 = In Range and Coerce(upper limit=w1265, x=w1268, lower limit=w1266) -> (coerced(x)=w1267:dbl)  [unwired: 1 out]
        n738 = To Long Integer(number=w1267) -> (32bit integer=w1270:i32)
        n739 = property on="R Scan Length SP steps" class="DigNum (strict)"("Val(Sgnl)"=w1270) -> ()  [unwired: 2 in, 2 out]
        n740 = property on="R Scan Velocity SP deg/sec" class="DigNum (strict)"() -> ("Value"=w1263:dbl)  [unwired: 2 in, 2 out]
        n741 = property on="R Velocity SP step/sec" class="DigNum (strict)"() -> ("Maximum"=w1259:dbl)  [unwired: 2 in, 2 out]
        n742 = property on="R Scan Velocity SP steps/sec" class="DigNum (strict)"() -> ("Minimum"=w1258:dbl)  [unwired: 2 in, 2 out]
        n743 = Divide(x=w1263, y=w1256) -> (x/y=w1264:dbl)
        n744 = Multiply(x=w1264, y=w1257) -> (x*y=w1261:dbl)
        n745 = In Range and Coerce(upper limit=w1259, x=w1261, lower limit=w1258) -> (coerced(x)=w1260:dbl)  [unwired: 1 out]
        n746 = To Long Integer(number=w1260) -> (32bit integer=w1262:i32)
        n747 = property on="R Scan Velocity SP steps/sec" class="DigNum (strict)"("Val(Sgnl)"=w1262) -> ()  [unwired: 2 in, 2 out]
      }
      event #12 {
        n748 = event-data() -> ()  [unwired: 1 in, 7 out]
        n749 = flat-sequence {
          tunnel: w1277 -> [w1287]
          tunnel: w1278 -> [w1288]
          tunnel: [w1288] -> w1274
          tunnel: [w1287] -> w1273
          tunnel: [w1291] -> w1276
          tunnel: [w1290] -> w1275
          tunnel: w1274 -> [w1293]
          tunnel: w1273 -> [w1292]
          tunnel: [w1311] -> w1280
          tunnel: [w1310] -> w1279
          tunnel: w1276 -> [w1309]
          tunnel: w1275 -> [w1308]
          tunnel: [w1318] -> w1282
          tunnel: [w1317] -> w1281
          tunnel: w1280 -> [w1316]
          tunnel: w1279 -> [w1315]
          tunnel: [w1324] -> w1283
          tunnel: [w1325] -> w1284
          tunnel: w1282 -> [w1325]
          tunnel: w1281 -> [w1323]
          frame #0 {
            n750 = property on="Scan Go" class="Bool"("DisabledEnum"=T1."Disabled and Grayed Out" ("Disabled")) -> ()  [unwired: 2 in, 2 out]
            n751 = property on="Y Go" class="Bool"("DisabledEnum"=T1."Disabled and Grayed Out" ("Disabled")) -> ()  [unwired: 2 in, 2 out]
          }
          frame #1 {
            n752 = property on="Y Step SP" class="DigNum (strict)"() -> ("Value"=w1301:i32)  [unwired: 2 in, 2 out]
            n753 = property on="Y Step PV" class="DigNum (strict)"() -> ("Value"=w1300:i32)  [unwired: 2 in, 2 out]
            n754 = property on="Y Backlash" class="DigNum (strict)"() -> ("Value"=w1289:i32)  [unwired: 2 in, 2 out]
            n755 = Subtract(x=w1301, y=w1300) -> (x-y=w1299:i32)
            n756 = Sign(1:w1289) -> (0:w1297:i32)
            n757 = Sign(1:w1299) -> (0:w1298:i32)
            n758 = Multiply(x=w1298, y=w1297) -> (x*y=w1296:i32)
            n759 = Equal?(x=w1296, y=1) -> (x = y?=w1294:bool)
            n760 = case shown="False" w1294 {
              tunnel: w1293 -> [w1304 w1306]
              tunnel: w1292 -> [w1303 w1305]
              tunnel: [w1303 w1305] -> w1291
              tunnel: [w1304 w1306] -> w1290
              frame #0 {
                n761 = property on="Y Backlash corr" class="Bool (strict)"("Val(Sgnl)"=FALSE ("Value (Signaling)")) -> ()  [unwired: 2 in, 2 out]
              }
              frame #1 {
                n762 = property on="Y Backlash corr" class="Bool (strict)"("Val(Sgnl)"=TRUE ("Value (Signaling)")) -> ()  [unwired: 2 in, 2 out]
              }
            }
          }
          frame #2 {
            # "Velocity Setting"
            n763 = property on="Y Velocity SP step/sec" class="DigNum (strict)"() -> ("Value"=w1312:i32)  [unwired: 2 in, 2 out]
            n764 = Number To Decimal String(number=w1312) -> (decimal integer string=w1313:string)  [unwired: 1 in]
            n765 = call "mDrive Send Command.vi"("error in (no error)"=w1309, "Extra"=w1313, "Command"=T2."Max Velocity", "VISA resource name"=w1308) -> ("error out"=w1310:errorcluster, "VISA resource name out"=w1311:refnum<visa-resource-name>)  [unwired: 3 in, 1 out]
          }
          frame #3 {
            # "Move to Abs Position"
            n766 = property on="Y Step SP" class="DigNum (strict)"() -> ("Value"=w1321:i32)  [unwired: 2 in, 2 out]
            n767 = Number To Decimal String(number=w1321) -> (decimal integer string=w1320:string)  [unwired: 1 in]
            n768 = call "mDrive Send Command.vi"("error in (no error)"=w1315, "Extra"=w1320, "Command"=T2."Move to Absolute Position", "VISA resource name"=w1316) -> ("error out"=w1317:errorcluster, "VISA resource name out"=w1318:refnum<visa-resource-name>)  [unwired: 3 in, 1 out]
          }
          frame #4 {
            n769 = call "Time Delay"("error in (no error)"=w1323, "Delay Time (s)"=0.1) -> ("error out"=w1324:errorcluster)  [unwired: 9 in]
          }
        }
      }
      event #13 {
        n770 = event-data() -> ()  [unwired: 1 in, 7 out]
        n771 = flat-sequence {
          tunnel: w1328 -> [w1340]
          tunnel: w1329 -> [w1341]
          tunnel: [w1341] -> w1331
          tunnel: [w1340] -> w1330
          tunnel: [w1344] -> w1333
          tunnel: [w1343] -> w1332
          tunnel: w1331 -> [w1346]
          tunnel: w1330 -> [w1345]
          tunnel: [w1364] -> w1335
          tunnel: [w1363] -> w1334
          tunnel: w1333 -> [w1362]
          tunnel: w1332 -> [w1361]
          tunnel: [w1371] -> w1337
          tunnel: [w1370] -> w1336
          tunnel: w1335 -> [w1369]
          tunnel: w1334 -> [w1368]
          tunnel: [w1377] -> w1327
          tunnel: [w1378] -> w1326
          tunnel: w1337 -> [w1378]
          tunnel: w1336 -> [w1376]
          frame #0 {
            n772 = property on="Scan Go" class="Bool"("DisabledEnum"=T1."Disabled and Grayed Out" ("Disabled")) -> ()  [unwired: 2 in, 2 out]
            n773 = property on="Z Go" class="Bool"("DisabledEnum"=T1."Disabled and Grayed Out" ("Disabled")) -> ()  [unwired: 2 in, 2 out]
          }
          frame #1 {
            n774 = property on="Z Step SP" class="DigNum (strict)"() -> ("Value"=w1354:i32)  [unwired: 2 in, 2 out]
            n775 = property on="Z Step PV" class="DigNum (strict)"() -> ("Value"=w1353:i32)  [unwired: 2 in, 2 out]
            n776 = property on="Z Backlash" class="DigNum (strict)"() -> ("Value"=w1342:i32)  [unwired: 2 in, 2 out]
            n777 = Subtract(x=w1354, y=w1353) -> (x-y=w1352:i32)
            n778 = Sign(1:w1342) -> (0:w1350:i32)
            n779 = Sign(1:w1352) -> (0:w1351:i32)
            n780 = Multiply(x=w1351, y=w1350) -> (x*y=w1349:i32)
            n781 = Equal?(x=w1349, y=1) -> (x = y?=w1347:bool)
            n782 = case shown="False" w1347 {
              tunnel: w1346 -> [w1357 w1359]
              tunnel: w1345 -> [w1356 w1358]
              tunnel: [w1356 w1358] -> w1344
              tunnel: [w1357 w1359] -> w1343
              frame #0 {
                n783 = property on="Z Backlash corr" class="Bool (strict)"("Val(Sgnl)"=FALSE ("Value (Signaling)")) -> ()  [unwired: 2 in, 2 out]
              }
              frame #1 {
                n784 = property on="Y Backlash corr" class="Bool (strict)"("Val(Sgnl)"=TRUE ("Value (Signaling)")) -> ()  [unwired: 2 in, 2 out]
              }
            }
          }
          frame #2 {
            # "Velocity Setting"
            n785 = property on="Z Velocity SP step/sec" class="DigNum (strict)"() -> ("Value"=w1365:i32)  [unwired: 2 in, 2 out]
            n786 = Number To Decimal String(number=w1365) -> (decimal integer string=w1366:string)  [unwired: 1 in]
            n787 = call "mDrive Send Command.vi"("error in (no error)"=w1362, "Extra"=w1366, "Command"=T2."Max Velocity", "VISA resource name"=w1361) -> ("error out"=w1363:errorcluster, "VISA resource name out"=w1364:refnum<visa-resource-name>)  [unwired: 3 in, 1 out]
          }
          frame #3 {
            # "Move to Abs Position"
            n788 = property on="Z Step SP" class="DigNum (strict)"() -> ("Value"=w1374:i32)  [unwired: 2 in, 2 out]
            n789 = Number To Decimal String(number=w1374) -> (decimal integer string=w1373:string)  [unwired: 1 in]
            n790 = call "mDrive Send Command.vi"("error in (no error)"=w1368, "Extra"=w1373, "Command"=T2."Move to Absolute Position", "VISA resource name"=w1369) -> ("error out"=w1370:errorcluster, "VISA resource name out"=w1371:refnum<visa-resource-name>)  [unwired: 3 in, 1 out]
          }
          frame #4 {
            n791 = call "Time Delay28"("error in (no error)"=w1376, "Delay Time (s)"=0.1) -> ("error out"=w1377:errorcluster)  [unwired: 9 in]
          }
        }
      }
      event #14 {
        n792 = event-data() -> ()  [unwired: 1 in, 7 out]
        n793 = flat-sequence {
          tunnel: w1381 -> [w1393]
          tunnel: w1382 -> [w1394]
          tunnel: [w1394] -> w1384
          tunnel: [w1393] -> w1383
          tunnel: [w1397] -> w1386
          tunnel: [w1396] -> w1385
          tunnel: w1384 -> [w1399]
          tunnel: w1383 -> [w1398]
          tunnel: [w1417] -> w1388
          tunnel: [w1416] -> w1387
          tunnel: w1386 -> [w1415]
          tunnel: w1385 -> [w1414]
          tunnel: [w1424] -> w1390
          tunnel: [w1423] -> w1389
          tunnel: w1388 -> [w1422]
          tunnel: w1387 -> [w1421]
          tunnel: [w1430] -> w1380
          tunnel: [w1431] -> w1379
          tunnel: w1390 -> [w1431]
          tunnel: w1389 -> [w1429]
          frame #0 {
            n794 = property on="Scan Go" class="Bool"("DisabledEnum"=T1."Disabled and Grayed Out" ("Disabled")) -> ()  [unwired: 2 in, 2 out]
            n795 = property on="R Go" class="Bool"("DisabledEnum"=T1."Disabled and Grayed Out" ("Disabled")) -> ()  [unwired: 2 in, 2 out]
          }
          frame #1 {
            n796 = property on="R Step SP" class="DigNum (strict)"() -> ("Value"=w1407:i32)  [unwired: 2 in, 2 out]
            n797 = property on="R Step PV" class="DigNum (strict)"() -> ("Value"=w1406:i32)  [unwired: 2 in, 2 out]
            n798 = property on="R Backlash" class="DigNum (strict)"() -> ("Value"=w1395:i32)  [unwired: 2 in, 2 out]
            n799 = Subtract(x=w1407, y=w1406) -> (x-y=w1405:i32)
            n800 = Sign(1:w1395) -> (0:w1403:i32)
            n801 = Sign(1:w1405) -> (0:w1404:i32)
            n802 = Multiply(x=w1404, y=w1403) -> (x*y=w1402:i32)
            n803 = Equal?(x=w1402, y=1) -> (x = y?=w1400:bool)
            n804 = case shown="False" w1400 {
              tunnel: w1399 -> [w1410 w1412]
              tunnel: w1398 -> [w1409 w1411]
              tunnel: [w1409 w1411] -> w1397
              tunnel: [w1410 w1412] -> w1396
              frame #0 {
                n805 = property on="R Backlash corr" class="Bool (strict)"("Val(Sgnl)"=FALSE ("Value (Signaling)")) -> ()  [unwired: 2 in, 2 out]
              }
              frame #1 {
                n806 = property on="Y Backlash corr" class="Bool (strict)"("Val(Sgnl)"=TRUE ("Value (Signaling)")) -> ()  [unwired: 2 in, 2 out]
              }
            }
          }
          frame #2 {
            # "Velocity Setting"
            n807 = property on="R Velocity SP step/sec" class="DigNum (strict)"() -> ("Value"=w1418:i32)  [unwired: 2 in, 2 out]
            n808 = Number To Decimal String(number=w1418) -> (decimal integer string=w1419:string)  [unwired: 1 in]
            n809 = call "mDrive Send Command.vi"("error in (no error)"=w1415, "Extra"=w1419, "Command"=T2."Max Velocity", "VISA resource name"=w1414) -> ("error out"=w1416:errorcluster, "VISA resource name out"=w1417:refnum<visa-resource-name>)  [unwired: 3 in, 1 out]
          }
          frame #3 {
            # "Move to Abs Position"
            n810 = property on="R Step SP" class="DigNum (strict)"() -> ("Value"=w1427:i32)  [unwired: 2 in, 2 out]
            n811 = Number To Decimal String(number=w1427) -> (decimal integer string=w1426:string)  [unwired: 1 in]
            n812 = call "mDrive Send Command.vi"("error in (no error)"=w1421, "Extra"=w1426, "Command"=T2."Move to Absolute Position", "VISA resource name"=w1422) -> ("error out"=w1423:errorcluster, "VISA resource name out"=w1424:refnum<visa-resource-name>)  [unwired: 3 in, 1 out]
          }
          frame #4 {
            n813 = call "Time Delay29"("error in (no error)"=w1429, "Delay Time (s)"=0.1) -> ("error out"=w1430:errorcluster)  [unwired: 9 in]
          }
        }
      }
      event #15 {
        n814 = event-data() -> ()  [unwired: 1 in, 7 out]
        n815 = flat-sequence {
          tunnel: [w1445] -> w1437
          tunnel: [w1444] -> w1436
          tunnel: w1435 -> [w1445]
          tunnel: w1434 -> [w1444]
          tunnel: [w1450] -> w1439
          tunnel: [w1449] -> w1438
          tunnel: w1437 -> [w1452]
          tunnel: w1436 -> [w1451]
          tunnel: [w1470] -> w1441
          tunnel: [w1469] -> w1440
          tunnel: w1439 -> [w1468]
          tunnel: w1438 -> [w1467]
          tunnel: [w1477] -> w1443
          tunnel: [w1476] -> w1442
          tunnel: w1441 -> [w1475]
          tunnel: w1440 -> [w1474]
          tunnel: [w1483] -> w1432
          tunnel: [w1484] -> w1433
          tunnel: w1443 -> [w1484]
          tunnel: w1442 -> [w1482]
          frame #0 {
            n816 = property on="Scan Go" class="Bool"("DisabledEnum"=T1."Disabled and Grayed Out" ("Disabled")) -> ()  [unwired: 2 in, 2 out]
            n817 = property on="X Go" class="Bool"("DisabledEnum"=T1."Disabled and Grayed Out" ("Disabled")) -> ()  [unwired: 2 in, 2 out]
          }
          frame #1 {
            n818 = property on="X Step SP" class="DigNum (strict)"() -> ("Value"=w1460:i32)  [unwired: 2 in, 2 out]
            n819 = property on="X Step PV" class="DigNum (strict)"() -> ("Value"=w1459:i32)  [unwired: 2 in, 2 out]
            n820 = property on="X Backlash" class="DigNum (strict)"() -> ("Value"=w1448:i32)  [unwired: 2 in, 2 out]
            n821 = Subtract(x=w1460, y=w1459) -> (x-y=w1458:i32)
            n822 = Sign(1:w1448) -> (0:w1456:i32)
            n823 = Sign(1:w1458) -> (0:w1457:i32)
            n824 = Multiply(x=w1457, y=w1456) -> (x*y=w1455:i32)
            n825 = Equal?(x=w1455, y=1) -> (x = y?=w1453:bool)
            n826 = case shown="False" w1453 {
              tunnel: w1452 -> [w1463 w1465]
              tunnel: w1451 -> [w1462 w1464]
              tunnel: [w1462 w1464] -> w1450
              tunnel: [w1463 w1465] -> w1449
              frame #0 {
                n827 = property on="X Backlash corr" class="Bool (strict)"("Val(Sgnl)"=FALSE ("Value (Signaling)")) -> ()  [unwired: 2 in, 2 out]
              }
              frame #1 {
                n828 = property on="Y Backlash corr" class="Bool (strict)"("Val(Sgnl)"=TRUE ("Value (Signaling)")) -> ()  [unwired: 2 in, 2 out]
              }
            }
          }
          frame #2 {
            # "Velocity Setting"
            n829 = property on="X Scan Velocity SP steps/sec" class="DigNum (strict)"() -> ("Value"=w1471:i32)  [unwired: 2 in, 2 out]
            n830 = Number To Decimal String(number=w1471) -> (decimal integer string=w1472:string)  [unwired: 1 in]
            n831 = call "mDrive Send Command.vi"("error in (no error)"=w1468, "Extra"=w1472, "Command"=T2."Max Velocity", "VISA resource name"=w1467) -> ("error out"=w1469:errorcluster, "VISA resource name out"=w1470:refnum<visa-resource-name>)  [unwired: 3 in, 1 out]
          }
          frame #3 {
            # "Move to Abs Position"
            n832 = property on="X Step SP" class="DigNum (strict)"() -> ("Value"=w1480:i32)  [unwired: 2 in, 2 out]
            n833 = Number To Decimal String(number=w1480) -> (decimal integer string=w1479:string)  [unwired: 1 in]
            n834 = call "mDrive Send Command.vi"("error in (no error)"=w1474, "Extra"=w1479, "Command"=T2."Move to Absolute Position", "VISA resource name"=w1475) -> ("error out"=w1476:errorcluster, "VISA resource name out"=w1477:refnum<visa-resource-name>)  [unwired: 3 in, 1 out]
          }
          frame #4 {
            n835 = call "Time Delay15"("error in (no error)"=w1482, "Delay Time (s)"=0.1) -> ("error out"=w1483:errorcluster)  [unwired: 9 in]
          }
        }
      }
      event #16 {
        n836 = event-data() -> ()  [unwired: 1 in, 7 out]
        n837 = flat-sequence {
          tunnel: [w1500] -> w1492
          tunnel: [w1498] -> w1491
          tunnel: w1490 -> [w1494]
          tunnel: w1489 -> [w1493]
          tunnel: w1492 -> [w1515]
          tunnel: w1491 -> [w1514]
          tunnel: [w1515] -> w1486
          tunnel: [w1514] -> w1485
          tunnel: [w1517] -> w1487
          tunnel: [w1518] -> w1488
          tunnel: w1486 -> [w1518]
          tunnel: w1485 -> [w1517]
          frame #0 {
            # "VELOCITY"
            n838 = property on="X Scan Velocity SP steps/sec" class="DigNum (strict)"() -> ("Value"=w1501:i32)  [unwired: 2 in, 2 out]
            n839 = Number To Decimal String(number=w1501) -> (decimal integer string=w1502:string)  [unwired: 1 in]
            n840 = call "mDrive Send Command.vi"("error in (no error)"=w1493, "Extra"=w1502, "Command"=T2."Max Velocity", "VISA resource name"=w1494) -> ("error out"=w1503:errorcluster, "VISA resource name out"=w1508:refnum<visa-resource-name>)  [unwired: 3 in, 1 out]
            n841 = call "Time Delay9"("error in (no error)"=w1503) -> ("error out"=w1506:errorcluster)  [unwired: 10 in]
            n842 = call "mDrive Send Command.vi"("error in (no error)"=w1506, "Extra"="VM", "Command"=T2."Print Parameter", "VISA resource name"=w1508) -> ("error out"=w1499:errorcluster, "read buffer"=w1504:string, "VISA resource name out"=w1500:refnum<visa-resource-name>)  [unwired: 3 in]
            n843 = call "Time Delay10"("error in (no error)"=w1499) -> ("error out"=w1498:errorcluster)  [unwired: 10 in]
            n844 = Decimal String To Number(string=w1504, offset=0) -> (number=w1507:i32)  [unwired: 1 in, 1 out]
            n845 = property on="X velocity PV step/sec" class="DigNum (strict)"("Val(Sgnl)"=w1507) -> ()  [unwired: 2 in, 2 out]
          }
          frame #1 {
            n846 = property on="X Scan" class="Bool (strict)"("Val(Sgnl)"=TRUE ("Slew Ready 2")) -> ()  [unwired: 2 in, 2 out]
            n847 = property on="Scan Go" class="Bool"("DisabledEnum"=T1."Enabled" ("Disabled")) -> ()  [unwired: 2 in, 2 out]
            n848 = property on="Scan Cancel" class="Bool"("DisabledEnum"=T1."Enabled" ("Disabled")) -> ()  [unwired: 2 in, 2 out]
            n849 = property on="X Scan Length SP steps" class="DigNum (strict)"("DisabledEnum"=T1."Disabled and Grayed Out" ("Disabled")) -> ()  [unwired: 2 in, 2 out]
            n850 = property on="X Scan Velocity SP steps/sec" class="DigNum (strict)"("DisabledEnum"=T1."Disabled and Grayed Out" ("Disabled")) -> ()  [unwired: 2 in, 2 out]
          }
          frame #2 {
            n851 = property on="X Go" class="Bool"("DisabledEnum"=T1."Disabled and Grayed Out" ("Disabled")) -> ()  [unwired: 2 in, 2 out]
          }
        }
      }
      event #17 {
        n852 = event-data() -> ()  [unwired: 1 in, 7 out]
        n853 = flat-sequence {
          tunnel: w1526 -> [w1536]
          tunnel: w1525 -> [w1535]
          tunnel: [w1532] -> w1523
          tunnel: [w1530] -> w1522
          tunnel: w1523 -> [w1549]
          tunnel: w1522 -> [w1548]
          tunnel: [w1549] -> w1520
          tunnel: [w1548] -> w1519
          tunnel: [w1551] -> w1524
          tunnel: [w1552] -> w1521
          tunnel: w1520 -> [w1552]
          tunnel: w1519 -> [w1551]
          frame #0 {
            # "VELOCITY"
            n854 = property on="Y Scan Velocity SP steps/sec" class="DigNum (strict)"() -> ("Value"=w1533:i32)  [unwired: 2 in, 2 out]
            n855 = Number To Decimal String(number=w1533) -> (decimal integer string=w1534:string)  [unwired: 1 in]
            n856 = call "mDrive Send Command.vi"("error in (no error)"=w1536, "Extra"=w1534, "Command"=T2."Max Velocity", "VISA resource name"=w1535) -> ("error out"=w1537:errorcluster, "VISA resource name out"=w1542:refnum<visa-resource-name>)  [unwired: 3 in, 1 out]
            n857 = call "Time Delay5"("error in (no error)"=w1537) -> ("error out"=w1540:errorcluster)  [unwired: 10 in]
            n858 = call "mDrive Send Command.vi"("error in (no error)"=w1540, "Extra"="VM", "Command"=T2."Print Parameter", "VISA resource name"=w1542) -> ("error out"=w1531:errorcluster, "read buffer"=w1538:string, "VISA resource name out"=w1532:refnum<visa-resource-name>)  [unwired: 3 in]
            n859 = call "Time Delay6"("error in (no error)"=w1531) -> ("error out"=w1530:errorcluster)  [unwired: 10 in]
            n860 = Decimal String To Number(string=w1538, offset=0) -> (number=w1541:i32)  [unwired: 1 in, 1 out]
            n861 = property on="Y velocity PV step/sec" class="DigNum (strict)"("Val(Sgnl)"=w1541) -> ()  [unwired: 2 in, 2 out]
          }
          frame #1 {
            n862 = property on="Y Scan" class="Bool (strict)"("Val(Sgnl)"=TRUE ("Slew Ready 2")) -> ()  [unwired: 2 in, 2 out]
            n863 = property on="Scan Go" class="Bool"("DisabledEnum"=T1."Enabled" ("Disabled")) -> ()  [unwired: 2 in, 2 out]
            n864 = property on="Scan Cancel" class="Bool"("DisabledEnum"=T1."Enabled" ("Disabled")) -> ()  [unwired: 2 in, 2 out]
            n865 = property on="Y Scan Length SP steps" class="DigNum (strict)"("DisabledEnum"=T1."Disabled and Grayed Out" ("Disabled")) -> ()  [unwired: 2 in, 2 out]
            n866 = property on="Y Scan Velocity SP steps/sec" class="DigNum (strict)"("DisabledEnum"=T1."Disabled and Grayed Out" ("Disabled")) -> ()  [unwired: 2 in, 2 out]
          }
          frame #2 {
            n867 = property on="Y Go" class="Bool"("DisabledEnum"=T1."Disabled and Grayed Out" ("Disabled")) -> ()  [unwired: 2 in, 2 out]
          }
        }
      }
      event #18 {
        n868 = event-data() -> ()  [unwired: 1 in, 7 out]
        n869 = flat-sequence {
          tunnel: [w1568] -> w1560
          tunnel: [w1566] -> w1559
          tunnel: w1556 -> [w1562]
          tunnel: w1555 -> [w1561]
          tunnel: w1560 -> [w1583]
          tunnel: w1559 -> [w1582]
          tunnel: [w1583] -> w1558
          tunnel: [w1582] -> w1557
          tunnel: [w1585] -> w1554
          tunnel: [w1586] -> w1553
          tunnel: w1558 -> [w1586]
          tunnel: w1557 -> [w1585]
          frame #0 {
            # "VELOCITY"
            n870 = property on="Z Scan Velocity SP steps/sec" class="DigNum (strict)"() -> ("Value"=w1569:i32)  [unwired: 2 in, 2 out]
            n871 = Number To Decimal String(number=w1569) -> (decimal integer string=w1570:string)  [unwired: 1 in]
            n872 = call "mDrive Send Command.vi"("error in (no error)"=w1561, "Extra"=w1570, "Command"=T2."Max Velocity", "VISA resource name"=w1562) -> ("error out"=w1571:errorcluster, "VISA resource name out"=w1576:refnum<visa-resource-name>)  [unwired: 3 in, 1 out]
            n873 = call "Time Delay24"("error in (no error)"=w1571) -> ("error out"=w1574:errorcluster)  [unwired: 10 in]
            n874 = call "mDrive Send Command.vi"("error in (no error)"=w1574, "Extra"="VM", "Command"=T2."Print Parameter", "VISA resource name"=w1576) -> ("error out"=w1567:errorcluster, "read buffer"=w1572:string, "VISA resource name out"=w1568:refnum<visa-resource-name>)  [unwired: 3 in]
            n875 = call "Time Delay25"("error in (no error)"=w1567) -> ("error out"=w1566:errorcluster)  [unwired: 10 in]
            n876 = Decimal String To Number(string=w1572, offset=0) -> (number=w1575:i32)  [unwired: 1 in, 1 out]
            n877 = property on="Z  velocity PV step/sec" class="DigNum (strict)"("Val(Sgnl)"=w1575) -> ()  [unwired: 2 in, 2 out]
          }
          frame #1 {
            n878 = property on="Z Scan" class="Bool (strict)"("Val(Sgnl)"=TRUE ("Slew Ready 2")) -> ()  [unwired: 2 in, 2 out]
            n879 = property on="Scan Go" class="Bool"("DisabledEnum"=T1."Enabled" ("Disabled")) -> ()  [unwired: 2 in, 2 out]
            n880 = property on="Scan Cancel" class="Bool"("DisabledEnum"=T1."Enabled" ("Disabled")) -> ()  [unwired: 2 in, 2 out]
            n881 = property on="Z Scan Length SP steps" class="DigNum (strict)"("DisabledEnum"=T1."Disabled and Grayed Out" ("Disabled")) -> ()  [unwired: 2 in, 2 out]
            n882 = property on="Z Scan Velocity SP steps/sec" class="DigNum (strict)"("DisabledEnum"=T1."Disabled and Grayed Out" ("Disabled")) -> ()  [unwired: 2 in, 2 out]
          }
          frame #2 {
            n883 = property on="Z Go" class="Bool"("DisabledEnum"=T1."Disabled and Grayed Out" ("Disabled")) -> ()  [unwired: 2 in, 2 out]
          }
        }
      }
      event #19 {
        n884 = event-data() -> ()  [unwired: 1 in, 7 out]
        n885 = flat-sequence {
          tunnel: [w1602] -> w1594
          tunnel: [w1600] -> w1593
          tunnel: w1590 -> [w1596]
          tunnel: w1589 -> [w1595]
          tunnel: w1594 -> [w1617]
          tunnel: w1593 -> [w1616]
          tunnel: [w1617] -> w1592
          tunnel: [w1616] -> w1591
          tunnel: [w1619] -> w1587
          tunnel: [w1620] -> w1588
          tunnel: w1592 -> [w1620]
          tunnel: w1591 -> [w1619]
          frame #0 {
            # "VELOCITY"
            n886 = property on="R Scan Velocity SP steps/sec" class="DigNum (strict)"() -> ("Value"=w1603:i32)  [unwired: 2 in, 2 out]
            n887 = Number To Decimal String(number=w1603) -> (decimal integer string=w1604:string)  [unwired: 1 in]
            n888 = call "mDrive Send Command.vi"("error in (no error)"=w1595, "Extra"=w1604, "Command"=T2."Max Velocity", "VISA resource name"=w1596) -> ("error out"=w1605:errorcluster, "VISA resource name out"=w1610:refnum<visa-resource-name>)  [unwired: 3 in, 1 out]
            n889 = call "Time Delay26"("error in (no error)"=w1605) -> ("error out"=w1608:errorcluster)  [unwired: 10 in]
            n890 = call "mDrive Send Command.vi"("error in (no error)"=w1608, "Extra"="VM", "Command"=T2."Print Parameter", "VISA resource name"=w1610) -> ("error out"=w1601:errorcluster, "read buffer"=w1606:string, "VISA resource name out"=w1602:refnum<visa-resource-name>)  [unwired: 3 in]
            n891 = call "Time Delay27"("error in (no error)"=w1601) -> ("error out"=w1600:errorcluster)  [unwired: 10 in]
            n892 = Decimal String To Number(string=w1606, offset=0) -> (number=w1609:i32)  [unwired: 1 in, 1 out]
            n893 = property on="R velocity PV step/sec" class="DigNum (strict)"("Val(Sgnl)"=w1609) -> ()  [unwired: 2 in, 2 out]
          }
          frame #1 {
            n894 = property on="R Scan" class="Bool (strict)"("Val(Sgnl)"=TRUE ("Slew Ready 2")) -> ()  [unwired: 2 in, 2 out]
            n895 = property on="Scan Go" class="Bool"("DisabledEnum"=T1."Enabled" ("Disabled")) -> ()  [unwired: 2 in, 2 out]
            n896 = property on="Scan Cancel" class="Bool"("DisabledEnum"=T1."Enabled" ("Disabled")) -> ()  [unwired: 2 in, 2 out]
            n897 = property on="R Scan Length SP steps" class="DigNum (strict)"("DisabledEnum"=T1."Disabled and Grayed Out" ("Disabled")) -> ()  [unwired: 2 in, 2 out]
            n898 = property on="R Scan Velocity SP steps/sec" class="DigNum (strict)"("DisabledEnum"=T1."Disabled and Grayed Out" ("Disabled")) -> ()  [unwired: 2 in, 2 out]
          }
          frame #2 {
            n899 = property on="R Go" class="Bool"("DisabledEnum"=T1."Disabled and Grayed Out" ("Disabled")) -> ()  [unwired: 2 in, 2 out]
          }
        }
      }
      event #20 {
        n900 = event-data() -> ()  [unwired: 1 in, 4 out]
        n901 = event-data() -> ()  [unwired: 3 in, 1 out]
      }
      event #21 {
        n902 = event-data() -> ()  [unwired: 1 in, 7 out]
        n903 = flat-sequence {
          tunnel: [w1653] -> w1635
          tunnel: [w1652] -> w1634
          tunnel: w1633 -> [w1651]
          tunnel: w1632 -> [w1650]
          frame #0 {
            n904 = call "mDrive Send Command.vi"("error in (no error)"=w1650, "Command"=T2."Stop", "VISA resource name"=w1651) -> ("error out"=w1652:errorcluster, "VISA resource name out"=w1653:refnum<visa-resource-name>)  [unwired: 4 in, 1 out]
          }
        }
        n905 = flat-sequence {
          tunnel: w1639 -> [w1659]
          tunnel: w1638 -> [w1658]
          tunnel: [w1657] -> w1637
          tunnel: [w1656] -> w1636
          frame #0 {
            n906 = call "mDrive Send Command.vi"("error in (no error)"=w1658, "Command"=T2."Stop", "VISA resource name"=w1659) -> ("error out"=w1656:errorcluster, "VISA resource name out"=w1657:refnum<visa-resource-name>)  [unwired: 4 in, 1 out]
          }
        }
        n907 = flat-sequence {
          tunnel: [w1648] -> w1629
          tunnel: [w1647] -> w1628
          tunnel: w1631 -> [w1646]
          tunnel: w1630 -> [w1645]
          frame #0 {
            n908 = call "mDrive Send Command.vi"("error in (no error)"=w1645, "Command"=T2."Stop", "VISA resource name"=w1646) -> ("error out"=w1647:errorcluster, "VISA resource name out"=w1648:refnum<visa-resource-name>)  [unwired: 4 in, 1 out]
          }
        }
        n909 = flat-sequence {
          tunnel: w1627 -> [w1644]
          tunnel: w1626 -> [w1643]
          tunnel: [w1642] -> w1625
          tunnel: [w1640] -> _
          tunnel: [w1640] -> w1624
          frame #0 {
            n910 = call "mDrive Send Command.vi"("error in (no error)"=w1643, "Command"=T2."Stop", "VISA resource name"=w1644) -> ("error out"=w1640:errorcluster, "VISA resource name out"=w1642:refnum<visa-resource-name>)  [unwired: 4 in, 1 out]
          }
        }
      }
      event #22 {
        n911 = event-data() -> ()  [unwired: 1 in, 7 out]
        n912 = property on="Scan Go" class="Bool"("DisabledEnum"=T1."Disabled and Grayed Out" ("Disabled")) -> ()  [unwired: 2 in, 2 out]
        n913 = property on="Scan Cancel" class="Bool"("DisabledEnum"=T1."Disabled and Grayed Out" ("Disabled")) -> ()  [unwired: 2 in, 2 out]
        n914 = flat-sequence {
          tunnel: w1675 -> [w1714]
          tunnel: w1674 -> [w1713]
          tunnel: [w1716] -> w1677
          tunnel: [w1715] -> w1676
          tunnel: [w1723] -> w1672
          tunnel: [w1724] -> w1673
          tunnel: w1677 -> [w1724]
          tunnel: w1676 -> [w1723]
          frame #0 {
            n915 = call "mDrive Send Command.vi"("error in (no error)"=w1713, "Command"=T2."Stop", "VISA resource name"=w1714) -> ("error out"=w1715:errorcluster, "VISA resource name out"=w1716:refnum<visa-resource-name>)  [unwired: 4 in, 1 out]
          }
          frame #1 {
            n916 = property on="X Scan" class="Bool (strict)"("Value"=FALSE ("Slew Ready")) -> ()  [unwired: 2 in, 2 out]
            n917 = property on="X Scan set" class="Bool"("DisabledEnum"=T1."Enabled" ("Disabled")) -> ()  [unwired: 2 in, 2 out]
            n918 = property on="X Scan Velocity SP steps/sec" class="DigNum (strict)"("DisabledEnum"=T1."Enabled" ("Disabled")) -> ()  [unwired: 2 in, 2 out]
            n919 = property on="X Scan Length SP steps" class="DigNum (strict)"("DisabledEnum"=T1."Enabled" ("Disabled")) -> ()  [unwired: 2 in, 2 out]
            n920 = property on="X Go" class="Bool"("DisabledEnum"=T1."Enabled" ("Disabled")) -> ()  [unwired: 2 in, 2 out]
            n921 = property on="X Scan OK" class="Bool"("DisabledEnum"=T1."Enabled" ("Disabled")) -> ()  [unwired: 2 in, 2 out]
          }
        }
        n922 = flat-sequence {
          tunnel: w1683 -> [w1727]
          tunnel: w1682 -> [w1726]
          tunnel: [w1729] -> w1679
          tunnel: [w1728] -> w1678
          tunnel: [w1736] -> w1684
          tunnel: [w1737] -> w1685
          tunnel: w1679 -> [w1737]
          tunnel: w1678 -> [w1736]
          frame #0 {
            n923 = call "mDrive Send Command.vi"("error in (no error)"=w1726, "Command"=T2."Stop", "VISA resource name"=w1727) -> ("error out"=w1728:errorcluster, "VISA resource name out"=w1729:refnum<visa-resource-name>)  [unwired: 4 in, 1 out]
          }
          frame #1 {
            n924 = property on="Y Scan" class="Bool (strict)"("Value"=FALSE ("Slew Ready")) -> ()  [unwired: 2 in, 2 out]
            n925 = property on="Y Scan Velocity SP steps/sec" class="DigNum (strict)"("DisabledEnum"=T1."Enabled" ("Disabled")) -> ()  [unwired: 2 in, 2 out]
            n926 = property on="Y Go" class="Bool"("DisabledEnum"=T1."Enabled" ("Disabled")) -> ()  [unwired: 2 in, 2 out]
            n927 = property on="Y Scan OK" class="Bool"("DisabledEnum"=T1."Enabled" ("Disabled")) -> ()  [unwired: 2 in, 2 out]
            n928 = property on="Y Scan Length SP steps" class="DigNum (strict)"("DisabledEnum"=T1."Enabled" ("Disabled")) -> ()  [unwired: 2 in, 2 out]
            n929 = property on="Y Scan set" class="Bool"("DisabledEnum"=T1."Enabled" ("Disabled")) -> ()  [unwired: 2 in, 2 out]
          }
        }
        n930 = flat-sequence {
          tunnel: [w1703] -> w1671
          tunnel: [w1702] -> w1670
          tunnel: w1669 -> [w1700]
          tunnel: w1668 -> [w1699]
          tunnel: [w1710] -> w1666
          tunnel: [w1711] -> w1667
          tunnel: w1671 -> [w1711]
          tunnel: w1670 -> [w1710]
          frame #0 {
            n931 = call "mDrive Send Command.vi"("error in (no error)"=w1699, "Command"=T2."Stop", "VISA resource name"=w1700) -> ("error out"=w1702:errorcluster, "VISA resource name out"=w1703:refnum<visa-resource-name>)  [unwired: 4 in, 1 out]
          }
          frame #1 {
            n932 = property on="Z Scan" class="Bool (strict)"("Value"=FALSE ("Slew Ready")) -> ()  [unwired: 2 in, 2 out]
            n933 = property on="Z Scan set" class="Bool"("DisabledEnum"=T1."Enabled" ("Disabled")) -> ()  [unwired: 2 in, 2 out]
            n934 = property on="Z Scan Velocity SP steps/sec" class="DigNum (strict)"("DisabledEnum"=T1."Enabled" ("Disabled")) -> ()  [unwired: 2 in, 2 out]
            n935 = property on="Z Scan Length SP steps" class="DigNum (strict)"("DisabledEnum"=T1."Enabled" ("Disabled")) -> ()  [unwired: 2 in, 2 out]
            n936 = property on="Z Go" class="Bool"("DisabledEnum"=T1."Enabled" ("Disabled")) -> ()  [unwired: 2 in, 2 out]
            n937 = property on="Z Scan OK" class="Bool"("DisabledEnum"=T1."Enabled" ("Disabled")) -> ()  [unwired: 2 in, 2 out]
          }
        }
        n938 = flat-sequence {
          tunnel: [w1690] -> w1665
          tunnel: [w1689] -> w1664
          tunnel: w1663 -> [w1687]
          tunnel: w1662 -> [w1686]
          tunnel: [w1697] -> w1660
          tunnel: [w1698] -> w1661
          tunnel: w1665 -> [w1698]
          tunnel: w1664 -> [w1697]
          frame #0 {
            n939 = call "mDrive Send Command.vi"("error in (no error)"=w1686, "Command"=T2."Stop", "VISA resource name"=w1687) -> ("error out"=w1689:errorcluster, "VISA resource name out"=w1690:refnum<visa-resource-name>)  [unwired: 4 in, 1 out]
          }
          frame #1 {
            n940 = property on="R Scan" class="Bool (strict)"("Value"=FALSE ("Slew Ready")) -> ()  [unwired: 2 in, 2 out]
            n941 = property on="R Scan OK" class="Bool"("DisabledEnum"=T1."Enabled" ("Disabled")) -> ()  [unwired: 2 in, 2 out]
            n942 = property on="R Scan Length SP steps" class="DigNum (strict)"("DisabledEnum"=T1."Enabled" ("Disabled")) -> ()  [unwired: 2 in, 2 out]
            n943 = property on="R Scan set" class="Bool"("DisabledEnum"=T1."Enabled" ("Disabled")) -> ()  [unwired: 2 in, 2 out]
            n944 = property on="R Scan Velocity SP steps/sec" class="DigNum (strict)"("DisabledEnum"=T1."Enabled" ("Disabled")) -> ()  [unwired: 2 in, 2 out]
            n945 = property on="R Go" class="Bool"("DisabledEnum"=T1."Enabled" ("Disabled")) -> ()  [unwired: 2 in, 2 out]
          }
        }
      }
      event #23 {
        n946 = event-data() -> ()  [unwired: 1 in, 7 out]
        n947 = property on="Y Scan" class="Bool (strict)"() -> ("Value"=w1741:bool)  [unwired: 2 in, 2 out]
        n948 = flat-sequence {
          tunnel: w1754 -> [w1757]
          tunnel: w1753 -> [w1758]
          tunnel: [w1758] -> w1750
          tunnel: [w1757] -> w1749
          tunnel: [w1756] -> w1748
          tunnel: w1741 -> [w1755]
          tunnel: [w1755] -> w1740
          tunnel: w1750 -> [w1769]
          tunnel: [w1771] -> w1745
          tunnel: w1749 -> [w1768]
          tunnel: [w1770] -> w1743
          tunnel: w1748 -> [w1767]
          tunnel: w1740 -> [w1766]
          tunnel: [w1766] -> w1738
          tunnel: w1745 -> [w1782]
          tunnel: [w1782] -> w1744
          tunnel: w1743 -> [w1781]
          tunnel: [w1781] -> w1742
          tunnel: [w1779] -> w1739
          tunnel: w1738 -> [w1779]
          tunnel: w1744 -> [w1787]
          tunnel: [w1785] -> w1747
          tunnel: w1742 -> [w1786]
          tunnel: [w1784] -> w1746
          tunnel: w1739 -> [w1783]
          tunnel: w1747 -> [w1803]
          tunnel: w1746 -> [w1802]
          tunnel: [w1803] -> w1752
          tunnel: [w1802] -> w1751
          frame #0 {
            n949 = case shown="True" w1755 {
              tunnel: ["" w1760] -> w1756
              frame #0 {
              }
              frame #1 {
                n950 = property on="Y Scan Length SP steps" class="DigNum (strict)"() -> ("Value"=w1765:i32)  [unwired: 2 in, 2 out]
                n951 = Number To Decimal String(number=w1765) -> (decimal integer string=w1762:string)  [unwired: 1 in]
                n952 = call <vilib>:"Space Constant.vi"() -> ("String"=w1763:string)
                n953 = Concatenate Strings("MR", w1763, w1762, "\r") -> (w1760:string)
              }
            }
          }
          frame #1 {
            n954 = case shown="True" w1766 {
              tunnel: [w1773 w1778] -> w1771
              tunnel: [w1772 w1777] -> w1770
              tunnel: w1769 -> [w1773 w1776]
              tunnel: w1768 -> [w1772 w1775]
              tunnel: w1767 -> [_ w1774]
              frame #0 {
              }
              frame #1 {
                n955 = VISA Write(VISA resource name=w1776, write buffer=w1774, error in (no error)=w1775) -> (VISA resource name out=w1778:refnum<visa-resource-name>, error out=w1777:errorcluster)  [unwired: 1 out]
              }
            }
          }
          frame #2 {
            n956 = call "Time Delay7"("Delay Time (s)"=0.1) -> ()  [unwired: 10 in, 1 out]
          }
          frame #3 {
            n957 = case shown="True" w1783 {
              tunnel: w1787 -> [w1789 w1793]
              tunnel: w1786 -> [w1788 w1792]
              tunnel: [w1789 w1791] -> w1785
              tunnel: [w1788 w1790] -> w1784
              frame #0 {
              }
              frame #1 {
                n958 = property class="Instr"(reference=w1793, error in=w1792) -> (reference out=w1795:refnum<visa-resource-name>, error out=w1794:errorcluster, "Serial Settings:Number of Bytes at Serial Port"=w1796:u32)
                n959 = VISA Read(VISA resource name=w1795, byte count=w1796, error in (no error)=w1794) -> (VISA resource name out=w1791:refnum<visa-resource-name>, error out=w1790:errorcluster)  [unwired: 2 out]
              }
            }
          }
          frame #4 {
            n960 = property on="Y Scan" class="Bool (strict)"("Val(Sgnl)"=FALSE ("Slew Ready 2")) -> ()  [unwired: 2 in, 2 out]
            n961 = property on="Slew Velocity" class="DigNum (strict)"("DisabledEnum"=T1."Enabled" ("Disabled")) -> ()  [unwired: 2 in, 2 out]
            n962 = property on="Y Scan Length SP steps" class="DigNum (strict)"("DisabledEnum"=T1."Enabled" ("Disabled")) -> ()  [unwired: 2 in, 2 out]
            n963 = property on="Scan Go" class="Bool"("DisabledEnum"=T1."Disabled and Grayed Out" ("Disabled")) -> ()  [unwired: 2 in, 2 out]
            n964 = property on="Scan Cancel" class="Bool"("DisabledEnum"=T1."Disabled and Grayed Out" ("Disabled")) -> ()  [unwired: 2 in, 2 out]
          }
        }
      }
      event #24 {
        n965 = event-data() -> ()  [unwired: 1 in, 7 out]
        n966 = flat-sequence {
          tunnel: [w1834] -> w1813
          tunnel: w1814 -> [w1837]
          tunnel: [w1836] -> w1812
          tunnel: w1815 -> [w1835]
          frame #0 {
            n967 = property on="Reset X Motor Steps" class="DigNum (strict)"() -> ("Value"=w1838:i32)  [unwired: 2 in, 2 out]
            n968 = Number To Decimal String(number=w1838) -> (decimal integer string=w1839:string)  [unwired: 1 in]
            n969 = call "mDrive Send Command.vi"("error in (no error)"=w1837, "Extra"=w1839, "Command"=T2."Set Current Position", "VISA resource name"=w1835) -> ("error out"=w1836:errorcluster, "VISA resource name out"=w1834:refnum<visa-resource-name>)  [unwired: 3 in, 1 out]
          }
        }
        n970 = flat-sequence {
          tunnel: w1819 -> [w1844]
          tunnel: w1818 -> [w1843]
          tunnel: [w1842] -> w1817
          tunnel: [w1841] -> w1816
          frame #0 {
            n971 = property on="Reset Y Motor Steps" class="DigNum (strict)"() -> ("Value"=w1845:i32)  [unwired: 2 in, 2 out]
            n972 = Number To Decimal String(number=w1845) -> (decimal integer string=w1846:string)  [unwired: 1 in]
            n973 = call "mDrive Send Command.vi"("error in (no error)"=w1843, "Extra"=w1846, "Command"=T2."Set Current Position", "VISA resource name"=w1844) -> ("error out"=w1841:errorcluster, "VISA resource name out"=w1842:refnum<visa-resource-name>)  [unwired: 3 in, 1 out]
          }
        }
        n974 = flat-sequence {
          tunnel: [w1830] -> w1805
          tunnel: [w1829] -> w1804
          tunnel: w1811 -> [w1828]
          tunnel: w1810 -> [w1827]
          frame #0 {
            n975 = property on="Reset Z Motor Steps" class="DigNum (strict)"() -> ("Value"=w1831:i32)  [unwired: 2 in, 2 out]
            n976 = Number To Decimal String(number=w1831) -> (decimal integer string=w1832:string)  [unwired: 1 in]
            n977 = call "mDrive Send Command.vi"("error in (no error)"=w1827, "Extra"=w1832, "Command"=T2."Set Current Position", "VISA resource name"=w1828) -> ("error out"=w1829:errorcluster, "VISA resource name out"=w1830:refnum<visa-resource-name>)  [unwired: 3 in, 1 out]
          }
        }
        n978 = flat-sequence {
          tunnel: [w1821] -> w1807
          tunnel: [w1823] -> w1806
          tunnel: w1809 -> [w1822]
          tunnel: w1808 -> [w1820]
          frame #0 {
            n979 = property on="Reset R Motor Steps" class="DigNum (strict)"() -> ("Value"=w1824:i32)  [unwired: 2 in, 2 out]
            n980 = Number To Decimal String(number=w1824) -> (decimal integer string=w1825:string)  [unwired: 1 in]
            n981 = call "mDrive Send Command.vi"("error in (no error)"=w1820, "Extra"=w1825, "Command"=T2."Set Current Position", "VISA resource name"=w1822) -> ("error out"=w1823:errorcluster, "VISA resource name out"=w1821:refnum<visa-resource-name>)  [unwired: 3 in, 1 out]
          }
        }
      }
    }
    n982 = flat-sequence {
      frame #0 {
      }
    }
    n983 = flat-sequence {
      frame #0 {
      }
    }
    n984 = flat-sequence {
      frame #0 {
      }
    }
    n985 = flat-sequence {
      frame #0 {
      }
    }
    n986 = flat-sequence {
      frame #0 {
      }
    }
  }
  n987 = flat-sequence {
    tunnel: w60 -> [w1852]
    tunnel: w59 -> [w1849]
    frame #0 {
      n988 = call "mDrive Send Command.vi"("error in (no error)"=w1849, "Command"=T2."Stop", "VISA resource name"=w1852) -> ("error out"=w1850:errorcluster, "VISA resource name out"=w1851:refnum<visa-resource-name>)  [unwired: 4 in, 1 out]
      n989 = VISA Close(VISA resource name=w1851, error in (no error)=w1850) -> ()  [unwired: 1 out]
    }
  }
  n990 = flat-sequence {
    tunnel: w87 -> [w1857]
    tunnel: w86 -> [w1854]
    frame #0 {
      n991 = call "mDrive Send Command.vi"("error in (no error)"=w1854, "Command"=T2."Stop", "VISA resource name"=w1857) -> ("error out"=w1855:errorcluster, "VISA resource name out"=w1856:refnum<visa-resource-name>)  [unwired: 4 in, 1 out]
      n992 = VISA Close(VISA resource name=w1856, error in (no error)=w1855) -> ()  [unwired: 1 out]
    }
  }
  n993 = flat-sequence {
    tunnel: w14 -> [w1862]
    tunnel: w13 -> [w1859]
    frame #0 {
      n994 = call "mDrive Send Command.vi"("error in (no error)"=w1859, "Command"=T2."Stop", "VISA resource name"=w1862) -> ("error out"=w1860:errorcluster, "VISA resource name out"=w1861:refnum<visa-resource-name>)  [unwired: 4 in, 1 out]
      n995 = VISA Close(VISA resource name=w1861, error in (no error)=w1860) -> ()  [unwired: 1 out]
    }
  }
  n996 = flat-sequence {
    tunnel: w10 -> [w1867]
    tunnel: w9 -> [w1864]
    frame #0 {
      n997 = call "mDrive Send Command.vi"("error in (no error)"=w1864, "Command"=T2."Stop", "VISA resource name"=w1867) -> ("error out"=w1865:errorcluster, "VISA resource name out"=w1866:refnum<visa-resource-name>)  [unwired: 4 in, 1 out]
      n998 = VISA Close(VISA resource name=w1866, error in (no error)=w1865) -> ()  [unwired: 1 out]
    }
  }
  "Y COM PORT" <- w90
  "X COM PORT" <- w65
  "Z COM PORT" <- w52
  "R COM PORT" <- w19
